vi "Text control 2 v6.7_pump-specific.vi"() -> ()   [LabVIEW 2016]
panel:
  in  "Tab Control":enum32{"Main", "Other parameters"}(tab)
  out "Line running":i32
  out "Total lines":i32
  out "Path":path=path "C:/users/rlp38/09Apr2009LTtesting/test2.txt"
  out "I vs Vg":cluster{"Y data in":dbl[], "X data in":dbl[]}[](graph)
  out "Is max":dbl format="%.2e"
  out "Id max":dbl format="%.2e"
  out "Ig max":dbl format="%.2e"
  out "Imax vs time":cluster{"Y data in":dbl[], "X data in":dbl[]}[](graph)
  out "Imin vs time":cluster{"Y data in":dbl[], "X data in":dbl[]}[](graph)
  out "I vs Vd":cluster{"Y data in":dbl[], "X data in":dbl[]}[](graph)
  in  "Script":string="#-------------------------------------------------------\n# SPM pump cleaning script\n#\n# Version: 0.5\n# Author: Dimitrios Simatos\n# Last updated: 2018-01-05\n#-------------------------------------------------------\n# Description\n#\n# This script is designed to run the cleaning sequence of the SPM OEM pump.\n# This script needs to be run 4 times!\n#-------------------------------------------------------\n# Changes\n#\n# Placed initialization and hard stop commands in the beginning.\n#-------------------------------------------------------\n# Important points\n#\n# Never leave any liquid in the pump to dry after the experiments. If they dry, the residue may block the valve.\n# Always run the cleaning cycle after the experiments.\n# Use clockwise rotation when going up in valve port numbers and vice versa.\n#-------------------------------------------------------\n# Things to do before running the script\n#\n# Set time units to minutes.\n# Set filenames.\n# Replace the tubing, if necessary.\n#-------------------------------------------------------\n# Port connections\n#\n# Port 1: Waste\n# Port 2: Waste\n# Port 3: Various cleaning liquids\n# Port 4: Waste\n# Port 5: Waste\n# Port 6: Waste\n#\n# Between each of the 4 runs, the settings of Port 3 will change, according to the cleaning protocol.\n# The settings for Port 3 are:\n# 1st run: 1% v/v solution of sodium hypochlorite in ultrapure water\n# 2nd run: 0.1% w/v solution of sodium dodecyl sulfate in ultrapure water\n# 3rd run: Ultrapure water\n# 4th run: Waste (in air, not immersed in liquid)\n#-------------------------------------------------------\n# Cleaning protocol for the SPM OEM pump (from the manual)\n#\n# A cleaning procedure should be performed at the end of each day or in between two different experiments.\n# An effective cleaning can be performed in the following manner:\n# • Bleach solution to kill microorganisms\n# 1. Prepare a solution of 1% chlorine bleach and deionized water\n#    NOTE: Prepare a 1% v/v solution of sodium hypochlorite in deionized water\n# 2. Prepare a reservoir and place 1 tubing in the bleach solution and 5 tubings in a waste recipient\n# 3. Pick up the bleach solution through 1 port to entirely fill the syringe\n# 4. Sequentially output the syringe content through the remaining ports and throw it to the waste\n# 5. Repeat operation at least 2 times\n# • Detergent solution to remove debris\n# 1. Prepare a solution of 0.1% detergent and deionized water\n#    NOTE: Prepare a 0.1% w/v solution of sodium dodecyl sulfate in deionized water\n# 2. Move the tubing from the bleach solution reservoir and place it into a reservoir of detergent solution\n# 3. Pick up the detergent solution through 1 port to entirely fill the syringe\n# 4. Sequentially output the detergent solution through the remaining ports into the waste recipient\n# 5. Repeat operation at least 2 times\n# • Rinsing water to prepare the pump for your next experiment\n# 1. Move the tubing from the detergent solution reservoir and place it into a reservoir of deionized water\n# 2. Pick up the rinsing solution through 1 port to entirely fill the syringe\n# 3. Sequentially output the rinse water through the remaining ports into the waste recipient\n# 4. Repeat operation at least 2 times\n# • Replace the tubing, if necessary\n#-------------------------------------------------------\n# Pumping cycles and execution time\n#\n# Execution time for a single cycle: 6 x (1 min + 10 sec) = 7 minutes\n# Total execution time: 4 x 7 = 28 minutes\n# Since the script has to run 4 times, the cleaning lasts for: 4 x 28 = 112 minutes\n# Air must be the last to be pumped through the valve, to remove all liquids.\n# There are 4 pumping cycles. Each one draws a different liquid through port 3 and pumps it sequentially through ports 1,2,4,5,6.\n# During the sequential pumping, each port receives 200 ml of liquid (20% of the total syringe volume = 600 \"plunger units\")\n# The device must be disconnected from the port during the cleaning procedure.\n# All cycles are similar, except cycle 1 has the initialization command uncommented and the first report valve command commented.\n#-------------------------------------------------------\n# Volume of liquid needed\n#\n# Volume of liquid needed per cycle: 1 ml\n# Total volume of liquid needed per script run: 4 x 1 = 4 ml\n# Since the script has to run 4 times, the first 3 with different liquids, I need:\n# 4 ml of 1% v/v solution of sodium hypochlorite in ultrapure water\n# 4 ml of 0.1% w/v solution of sodium dodecyl sulfate in ultrapure water\n# 4 ml of ultrapure water\n#-------------------------------------------------------\n# Parameters\n#\n# Syringe size: 1 ml\n# Step resolution N = 0.01 mm\n# Drawing flow V = 300 pulses/second (6000 ul/min)\n# Pumping flow V = 300 pulses/second (6000 ul/min)\n#-------------------------------------------------------\n# Pump initialization\npump /1T #hard stop pump\npump /1ZR #initialize pump\n#-------------------------------------------------------\n# Cycle 1\n# Fill the syringe\npump /1Q #query pump\npump /1? #report absolute plunger position\n#pump /1?6 #report valve position\nwait-min 1 #wait 1 minute\npump /1N0R #set step resolution: 0.01 mm\npump /1Q #query pump\npump /1? #report absolute plunger position (the plunger should be at 0)\npump /1?6 #report valve position\nwait 1000 #wait 1 second\npump /1V300R #choose speed: 300 steps/s (6000 ul/min)\npump /1Q #query pump\nwait 1000 #wait 1 second\npump /1I3R #go to port 3, clockwise rotation\npump /1Q #query pump\npump /1?6 #report valve position\nwait 1000 #wait 1 second\npump /1A3000R #go to absolute position 3000 (= draw 1 ml)\nwait 30000 #wait 30 seconds\npump /1Q #query pump\npump /1? #report absolute plunger position (the plunger should have finished moving)\n#pump /1?6 #report valve position\n# The sequential pumping begins\n# Port 1\npump /1O1R #switch to port 1, counterclockwise rotation\npump /1Q #query pump\npump /1?6 #report valve position\npump /1A2400R #go to absolute position 2400 (= pump 200 ul)\npump /1Q #query pump\npump /1? #report absolute plunger position (the plunger should be moving to 0)\nwait-min 1 #wait 1 minute\npump /1? #report absolute plunger position (the plunger should have finished moving)\n# Port 2\npump /1I2R #switch to port 2, clockwise rotation\npump /1Q #query pump\npump /1?6 #report valve position\npump /1A1800R #go to absolute position 1800 (= pump 200 ul)\npump /1Q #query pump\npump /1? #report absolute plunger position (the plunger should be moving to 0)\nwait-min 1 #wait 1 minute\npump /1? #report absolute plunger position (the plunger should have finished moving)\n# Port 4\npump /1I4R #switch to port 4, clockwise rotation\npump /1Q #query pump\npump /1?6 #report valve position\npump /1A1200R #go to absolute position 1200 (= pump 200 ul)\npump /1Q #query pump\npump /1? #report absolute plunger position (the plunger should be moving to 0)\nwait-min 1 #wait 1 minute\npump /1? #report absolute plunger position (the plunger should have finished moving)\n# Port 5\npump /1I5R #switch to port 5, clockwise rotation\npump /1Q #query pump\npump /1?6 #report valve position\npump /1A600R #go to absolute position 600 (= pump 200 ul)\npump /1Q #query pump\npump /1? #report absolute plunger position (the plunger should be moving to 0)\nwait-min 1 #wait 1 minute\npump /1? #report absolute plunger position (the plunger should have finished moving)\n# Port 6\npump /1I6R #switch to port 6, clockwise rotation\npump /1Q #query pump\npump /1?6 #report valve position\npump /1A0R #go to absolute position 0 (= pump 200 ul)\npump /1Q #query pump\npump /1? #report absolute plunger position (the plunger should be moving to 0)\nwait-min 1 #wait 1 minute\npump /1? #report absolute plunger position (the plunger should have finished moving)\n#-------------------------------------------------------\n# Cycle 2\n# Fill the syringe\n#pump /1ZR #initialize pump\npump /1Q #query pump\npump /1? #report absolute plunger position\npump /1?6 #report valve position\nwait-min 1 #wait 1 minute\npump /1N0R #set step resolution: 0.01 mm\npump /1Q #query pump\npump /1? #report absolute plunger position (the plunger should be at 0)\npump /1?6 #report valve position\nwait 1000 #wait 1 second\npump /1V300R #choose speed: 300 steps/s (6000 ul/min)\npump /1Q #query pump\nwait 1000 #wait 1 second\npump /1O3R #go to port 3, counterclockwise rotation\npump /1Q #query pump\npump /1?6 #report valve position\nwait 1000 #wait 1 second\npump /1A3000R #go to absolute position 3000 (= draw 1 ml)\nwait 30000 #wait 30 seconds\npump /1Q #query pump\npump /1? #report absolute plunger position (the plunger should have finished moving)\n#pump /1?6 #report valve position\n# The sequential pumping begins\n# Port 1\npump /1O1R #switch to port 1, counterclockwise rotation\npump /1Q #query pump\npump /1?6 #report valve position\npump /1A2400R #go to absolute position 2400 (= pump 200 ul)\npump /1Q #query pump\npump /1? #report absolute plunger position (the plunger should be moving to 0)\nwait-min 1 #wait 1 minute\npump /1? #report absolute plunger position (the plunger should have finished moving)\n# Port 2\npump /1I2R #switch to port 2, clockwise rotation\npump /1Q #query pump\npump /1?6 #report valve position\npump /1A1800R #go to absolute position 1800 (= pump 200 ul)\npump /1Q #query pump\npump /1? #report absolute plunger position (the plunger should be moving to 0)\nwait-min 1 #wait 1 minute\npump /1? #report absolute plunger position (the plunger should have finished moving)\n# Port 4\npump /1I4R #switch to port 4, clockwise rotation\npump /1Q #query pump\npump /1?6 #report valve position\npump /1A1200R #go to absolute position 1200 (= pump 200 ul)\npump /1Q #query pump\npump /1? #report absolute plunger position (the plunger should be moving to 0)\nwait-min 1 #wait 1 minute\npump /1? #report absolute plunger position (the plunger should have finished moving)\n# Port 5\npump /1I5R #switch to port 5, clockwise rotation\npump /1Q #query pump\npump /1?6 #report valve position\npump /1A600R #go to absolute position 600 (= pump 200 ul)\npump /1Q #query pump\npump /1? #report absolute plunger position (the plunger should be moving to 0)\nwait-min 1 #wait 1 minute\npump /1? #report absolute plunger position (the plunger should have finished moving)\n# Port 6\npump /1I6R #switch to port 6, clockwise rotation\npump /1Q #query pump\npump /1?6 #report valve position\npump /1A0R #go to absolute position 0 (= pump 200 ul)\npump /1Q #query pump\npump /1? #report absolute plunger position (the plunger should be moving to 0)\nwait-min 1 #wait 1 minute\npump /1? #report absolute plunger position (the plunger should have finished moving)\n#-------------------------------------------------------\n# Cycle 3\n# Fill the syringe\n#pump /1ZR #initialize pump\npump /1Q #query pump\npump /1? #report absolute plunger position\npump /1?6 #report valve position\nwait-min 1 #wait 1 minute\npump /1N0R #set step resolution: 0.01 mm\npump /1Q #query pump\npump /1? #report absolute plunger position (the plunger should be at 0)\npump /1?6 #report valve position\nwait 1000 #wait 1 second\npump /1V300R #choose speed: 300 steps/s (6000 ul/min)\npump /1Q #query pump\nwait 1000 #wait 1 second\npump /1O3R #go to port 3, counterclockwise rotation\npump /1Q #query pump\npump /1?6 #report valve position\nwait 1000 #wait 1 second\npump /1A3000R #go to absolute position 3000 (= draw 1 ml)\nwait 30000 #wait 30 seconds\npump /1Q #query pump\npump /1? #report absolute plunger position (the plunger should have finished moving)\n#pump /1?6 #report valve position\n# The sequential pumping begins\n# Port 1\npump /1O1R #switch to port 1, counterclockwise rotation\npump /1Q #query pump\npump /1?6 #report valve position\npump /1A2400R #go to absolute position 2400 (= pump 200 ul)\npump /1Q #query pump\npump /1? #report absolute plunger position (the plunger should be moving to 0)\nwait-min 1 #wait 1 minute\npump /1? #report absolute plunger position (the plunger should have finished moving)\n# Port 2\npump /1I2R #switch to port 2, clockwise rotation\npump /1Q #query pump\npump /1?6 #report valve position\npump /1A1800R #go to absolute position 1800 (= pump 200 ul)\npump /1Q #query pump\npump /1? #report absolute plunger position (the plunger should be moving to 0)\nwait-min 1 #wait 1 minute\npump /1? #report absolute plunger position (the plunger should have finished moving)\n# Port 4\npump /1I4R #switch to port 4, clockwise rotation\npump /1Q #query pump\npump /1?6 #report valve position\npump /1A1200R #go to absolute position 1200 (= pump 200 ul)\npump /1Q #query pump\npump /1? #report absolute plunger position (the plunger should be moving to 0)\nwait-min 1 #wait 1 minute\npump /1? #report absolute plunger position (the plunger should have finished moving)\n# Port 5\npump /1I5R #switch to port 5, clockwise rotation\npump /1Q #query pump\npump /1?6 #report valve position\npump /1A600R #go to absolute position 600 (= pump 200 ul)\npump /1Q #query pump\npump /1? #report absolute plunger position (the plunger should be moving to 0)\nwait-min 1 #wait 1 minute\npump /1? #report absolute plunger position (the plunger should have finished moving)\n# Port 6\npump /1I6R #switch to port 6, clockwise rotation\npump /1Q #query pump\npump /1?6 #report valve position\npump /1A0R #go to absolute position 0 (= pump 200 ul)\npump /1Q #query pump\npump /1? #report absolute plunger position (the plunger should be moving to 0)\nwait-min 1 #wait 1 minute\npump /1? #report absolute plunger position (the plunger should have finished moving)\n#-------------------------------------------------------\n# Cycle 4\n# Fill the syringe\n#pump /1ZR #initialize pump\npump /1Q #query pump\npump /1? #report absolute plunger position\npump /1?6 #report valve position\nwait-min 1 #wait 1 minute\npump /1N0R #set step resolution: 0.01 mm\npump /1Q #query pump\npump /1? #report absolute plunger position (the plunger should be at 0)\npump /1?6 #report valve position\nwait 1000 #wait 1 second\npump /1V300R #choose speed: 300 steps/s (6000 ul/min)\npump /1Q #query pump\nwait 1000 #wait 1 second\npump /1O3R #go to port 3, counterclockwise rotation\npump /1Q #query pump\npump /1?6 #report valve position\nwait 1000 #wait 1 second\npump /1A3000R #go to absolute position 3000 (= draw 1 ml)\nwait 30000 #wait 30 seconds\npump /1Q #query pump\npump /1? #report absolute plunger position (the plunger should have finished moving)\n#pump /1?6 #report valve position\n# The sequential pumping begins\n# Port 1\npump /1O1R #switch to port 1, counterclockwise rotation\npump /1Q #query pump\npump /1?6 #report valve position\npump /1A2400R #go to absolute position 2400 (= pump 200 ul)\npump /1Q #query pump\npump /1? #report absolute plunger position (the plunger should be moving to 0)\nwait-min 1 #wait 1 minute\npump /1? #report absolute plunger position (the plunger should have finished moving)\n# Port 2\npump /1I2R #switch to port 2, clockwise rotation\npump /1Q #query pump\npump /1?6 #report valve position\npump /1A1800R #go to absolute position 1800 (= pump 200 ul)\npump /1Q #query pump\npump /1? #report absolute plunger position (the plunger should be moving to 0)\nwait-min 1 #wait 1 minute\npump /1? #report absolute plunger position (the plunger should have finished moving)\n# Port 4\npump /1I4R #switch to port 4, clockwise rotation\npump /1Q #query pump\npump /1?6 #report valve position\npump /1A1200R #go to absolute position 1200 (= pump 200 ul)\npump /1Q #query pump\npump /1? #report absolute plunger position (the plunger should be moving to 0)\nwait-min 1 #wait 1 minute\npump /1? #report absolute plunger position (the plunger should have finished moving)\n# Port 5\npump /1I5R #switch to port 5, clockwise rotation\npump /1Q #query pump\npump /1?6 #report valve position\npump /1A600R #go to absolute position 600 (= pump 200 ul)\npump /1Q #query pump\npump /1? #report absolute plunger position (the plunger should be moving to 0)\nwait-min 1 #wait 1 minute\npump /1? #report absolute plunger position (the plunger should have finished moving)\n# Port 6\npump /1I6R #switch to port 6, clockwise rotation\npump /1Q #query pump\npump /1?6 #report valve position\npump /1A0R #go to absolute position 0 (= pump 200 ul)\npump /1Q #query pump\npump /1? #report absolute plunger position (the plunger should be moving to 0)\nwait-min 1 #wait 1 minute\npump /1? #report absolute plunger position (the plunger should have finished moving)\n#-------------------------------------------------------"
  out "Command running:":string
  out "Serial port data":string
  out "Elapsed Time":dbl caption="Elapsed Time (s)"
  in  "Time Units":u16(ring)=1 items=["Seconds", "Minutes", "Hours"]
  in  "Time Offset":dbl caption="Set Start Time (s)"
  in  "Reset":bool
  in  "Auto Reset":bool
  in  "integration time":u32(slide) max=2 step=1 scale=0.0..2.0
  in  "Interrupt scan":bool
  out "Absolute plunger position vs time":cluster{"Y data in":dbl[], "X data in":dbl[]}[](graph)
  out "Valve position vs time":cluster{"Y data in":dbl[], "X data in":dbl[]}[](graph)
  out "Is on":dbl format="%.2e"
  out "Id on":dbl format="%.2e"
  out "Ig on":dbl format="%.2e"
  out "Ion vs time":cluster{"Y data in":dbl[], "X data in":dbl[]}[](graph)
  out "Ioff vs time":cluster{"Y data in":dbl[], "X data in":dbl[]}[](graph)
  out "Ig min":dbl format="%.2e"
  out "Id min":dbl format="%.2e"
  out "Is min":dbl format="%.2e"
  out "Is off":dbl format="%.2e"
  out "Id off":dbl format="%.2e"
  out "Ig off":dbl format="%.2e"
  in  "Integration time (long)":dbl=0.32 min=0.04 max=2.0 step=0.02 format="%.2f"
  in  "Integration time (short)":dbl=0.0019 min=8e-05 max=0.0019 step=8e-05 format="%^.0e"
  in  "Gate: Compliance":dbl=0.001 format="%.8f"
  in  "Drain: Compliance":dbl=0.001 format="%.8f"
  in  "Hard stop pump":bool
  in  "Halt pump":bool
  in  "Interrupt program":bool
  in  "Suffix (script)":string="step_1_up-H2O_initial_script.txt"
  in  "Filename (variable part)":string="step_1_up-H2O_initial_"
  in  "Plot output curve extrema vs time":bool
  in  "Plot transfer curve extrema vs time":bool=TRUE
  in  "Plot sample extrema vs time":bool
  out "I vs time (Bias Stress)":cluster{"Y data in":dbl[], "X data in":dbl[]}[](graph)
  in  "Gate Range\nmode":u16(ring) items=["Auto", "Limited", "Fixed"]
  in  "Gate Range":u8(slide)=6 max=11 scale=0.0..11.0
  in  "Source/Drain\nRange mode":u16(ring) items=["Auto", "Limited", "Fixed"]
  in  "Source/Drain Range":u8(slide)=6 max=11 scale=0.0..11.0
  in  "Panel Controls":T1={"Emergency Stop"=refnum, "TransGraph Max"=1e-05, "Text/Graph (text=false)"=TRUE} {"TransGraph Max" format="%.2e"}
  in  "Panel Controls 2":T2={"Emergency Stop"=refnum, "TransGraph Max"=1e-05, "Text/Graph (text=false)"=TRUE, "TransGraph Min"=1e-11} {"TransGraph Min" format="%.2e"; "TransGraph Max" format="%.2e"}
  in  "SMU4":cluster{"on/off":bool, "Voltage":dbl} {"Voltage" min=-100.0 max=100.0 format="%.2f"}
  in  "Full Reset":bool
  in  "Standby":T3
  out "error out":errorcluster
  in  "Delay before read (ms)":u32=1000
  in  "byte count":u32=64
  in  "Serial End Mode for Reads":u16(ring)=2 items=["None", "LastBit", "TermChar"]
  in  "Timeout (ms)":u32=10000
  in  "Enable Termination\nChar (T)":bool=TRUE
  in  "Termination char\n(0xA = '\\n' = LF)\n(0xD = '\\r' = CR)":u8=13 format="%.0x"
  in  "flow control":u16(ring) items=["None"=0, "XON/XOFF"=1, "RTS/CTS"=2, "DTR/DSR"=4]
  in  "stop bits":u16(ring)=10 items=["1.0"=10, "1.5"=15, "2.0"=20]
  in  "parity":u16(ring) items=["None", "Odd", "Even", "Mark", "Space"]
  in  "data bits":u16=8 min=5 max=8 step=1
  in  "VISA resource name":refnum<visa-resource-name>="COM6"
  in  "baud rate":u32=9600
  out "Timings Indicator":T4
  in  "Timings (overwritten by the Front Panel)":T5={"integration time"=0, "Short/Long integration time"=0.00064, "hold time (sec)"=0.0, "delay time (sec)"=0.0, "Step Time (0 disables)"=0.0, "sweep method"=0, "Pulse period"=0.005, "Base voltage"=0.0, "Pulse width"=0.0005} {"Pulse width" min=0.0005 max=0.1 step=0.0001 format="%.4f"; "Base voltage" format="%^.4e"; "Pulse period" min=0.005 max=1.0 step=0.0001 format="%.4f"; "sweep method" items=["Continuous", "Pulsed"]; "Step Time (0 disables)" format="%.2f"; "delay time (sec)" format="%.4f"; "hold time (sec)" format="%.4f"; "Short/Long integration time" format="%^.0e"; "integration time" scale=0.0..2.0}
  out "SMU4 Indicator":cluster{"on/off":bool, "Voltage":dbl} {"Voltage" min=-100.0 max=100.0 format="%.2f"}
  in  "Gate":T6={"Gate Start"=0.0, "Gate Stop"=2.0, "Gate Step (linear only)"=1.0, "Gate Compliance"=0.0001, "Gate PComp"=0.0, "Range mode"=0, "Range"=6} {"Range" max=11 scale=0.0..11.0; "Range mode" items=["Auto", "Limited", "Fixed"]; "Gate PComp" format="%^.2e"; "Gate Compliance" format="%^.2e"; "Gate Step (linear only)" format="%^.4e"; "Gate Stop" format="%^.4e"; "Gate Start" format="%^.4e"}
  in  "Drain 2":T7={"Drain Start"=0.0, "Drain Stop"=2.0, "Drain Compliance"=0.0001, "Drain Step"=1.0, "Drain PComp"=0.0, "Range mode"=0, "Range"=6} {"Range" max=11 scale=0.0..11.0; "Range mode" items=["Auto", "Limited", "Fixed"]; "Drain PComp" format="%^.2e"; "Drain Step" format="%^.4e"; "Drain Compliance" format="%^.2e"; "Drain Stop" format="%^.4e"; "Drain Start" format="%^.4e"}
  # "Syntax:\nitime [s|m|l] time(sec): [s|m|l] determines the integration time setting (small|medium|long) and time sets the value.\nNOTE: The value of the integration time has to be within the range allowed by its category (s|m|l), otherwise, the closest value will be used. (e.g. if the category is set to short but the time value is very long, the actual value used will be the maximum short integration time.\nIntegration times:\n    Short: Default: 640 us. Range: 8E-5 - 1.92E-3 seconds.\n    Medium: Fixed at 1 NPL cycle (0.02 seconds).\n    Long: Default: 16 NPL cycles (0.32 seconds). Range: 2-100 NPL cycles (0.04 seconds - 2 seconds).\ngaterangemode [a|l|f]\ndrainrangemode [a|l|f]\npulsed [on|off] PulsePeriod(sec) PulseBaseVoltage PulseONWidth(sec)\nstandby [on l off]\nwait NumMilliseconds\nwait-min NumMinutes\n# texthere = comment\nSMU4 [ON|OFF] Voltage\ntransfer [s|d] VgStart VgStop VgStep VdStart VdStop VdStep\noutput [s|d] VgStart VgStop VgStep VdStart VdStop VdStep\nsample Vg Vd NumSamples Time(s) SampleInterval(s)\nsamplei Idg NumSamples Time(s) SampleInterval(s) VDGcompliance\n100 samples is approximately 13 seconds with medium integration\n# If in doubt use SampleInterval(s) = 0.004\n    NOTE: When doing bias stress measurements, set the Time Units to \"Seconds\", as the \"sample\" command has been configured to give the output to seconds.\nstressV VG VD IGcompliance IDcompliance Duration(sec)\nstressI IDG VDGcompliance Duration(sec)\nvsu2pulse Bias Duration(s)\npulsedstressV [s|d] VEstop VgON VgOFF Period(s) PulseONwidth(s) Vd\nsample-fpp Vg Vd NumSamples Time\nresample-fpp Vg Vd\ntransfer-fpp [s|d] VgStart VgStop VgStep VdStart VdStop VdStep\noutput-fpp [s|d] VgStart VgStop VgStep VdStart VdStop VdStep\nserial SerialPortCommand\npump SerialPortCommand for the SPM pump\n\nSPM Pump Syntax (<x>: pump number, use 1 if only one pump):\nif the command syntax contains [R], then append the letter R to the command\n/<x>Q: query (a query command should follow each command)\n/<x>Z[R] or /<x>Y[R]: initialize pump\n/<x>N<n>[R] (<n>=0,1): <0> (<1>) microstep 0.01 mm (0.00125 mm) resolution\n/<x>I<n> (<n>=0-6): turn to port number n (clockwise)\n/<x>O<n> (<n>=0-6): turn to port number n (counterclockwise)\n/<x>X: Re-execute last command string\n/<x>G<n>[R] (<n>=0-60000): repeat command sequence (default: 0, 0=loop forever)\n/<x>g: Mark the start of a repeat sequence (max = 10)\n/<x>M<n>[R] (<n>=0-86400000): delay command execution by n milliseconds\n/<x>H: Halt; Pause the sequence after finishing the current move\n/<x>T: Hardstop; Interrupt the current move and suppress it from the sequence\n/<x>A<n>[R] (<n>=0-3000 with N=0, 0-24000 with N=1): absolute position\n/<x>P<n>[R] (<n>=0-3000 with N=0, 0-24000 with N=1): relative pickup\n/<x>D<n>[R] (<n>=0-3000 with N=0, 0-24000 with N=1): relative dispense\n/<x>V<n>[R] (<n>=1-1600 default: 150): set peak speed (pulses/sec)\nNOTE: The lowest speed limit is 1 pulse/sec, not 5, as the manual states.\n/<x>S<n>[R] (<n>=10-40 default: 22): set speed (NOT in pulses/sec, look in manual)\nNOTE: When controlled with absolute position, one does not need to pay special attention to the syringe that is mounted on the pump.\nWithdraw from lower stage (ports 3, 5), dispense from higher stage (ports 2, 4, 6).\nConnect Port 1 to waste."
  # "Time"
  # "1\n2\n3\n4\n5\n6\n7\n8\n9\n10\n11\n12\n13\n14\n15\n16\n17\n18\n19\n20"
  # "Serial port settings"
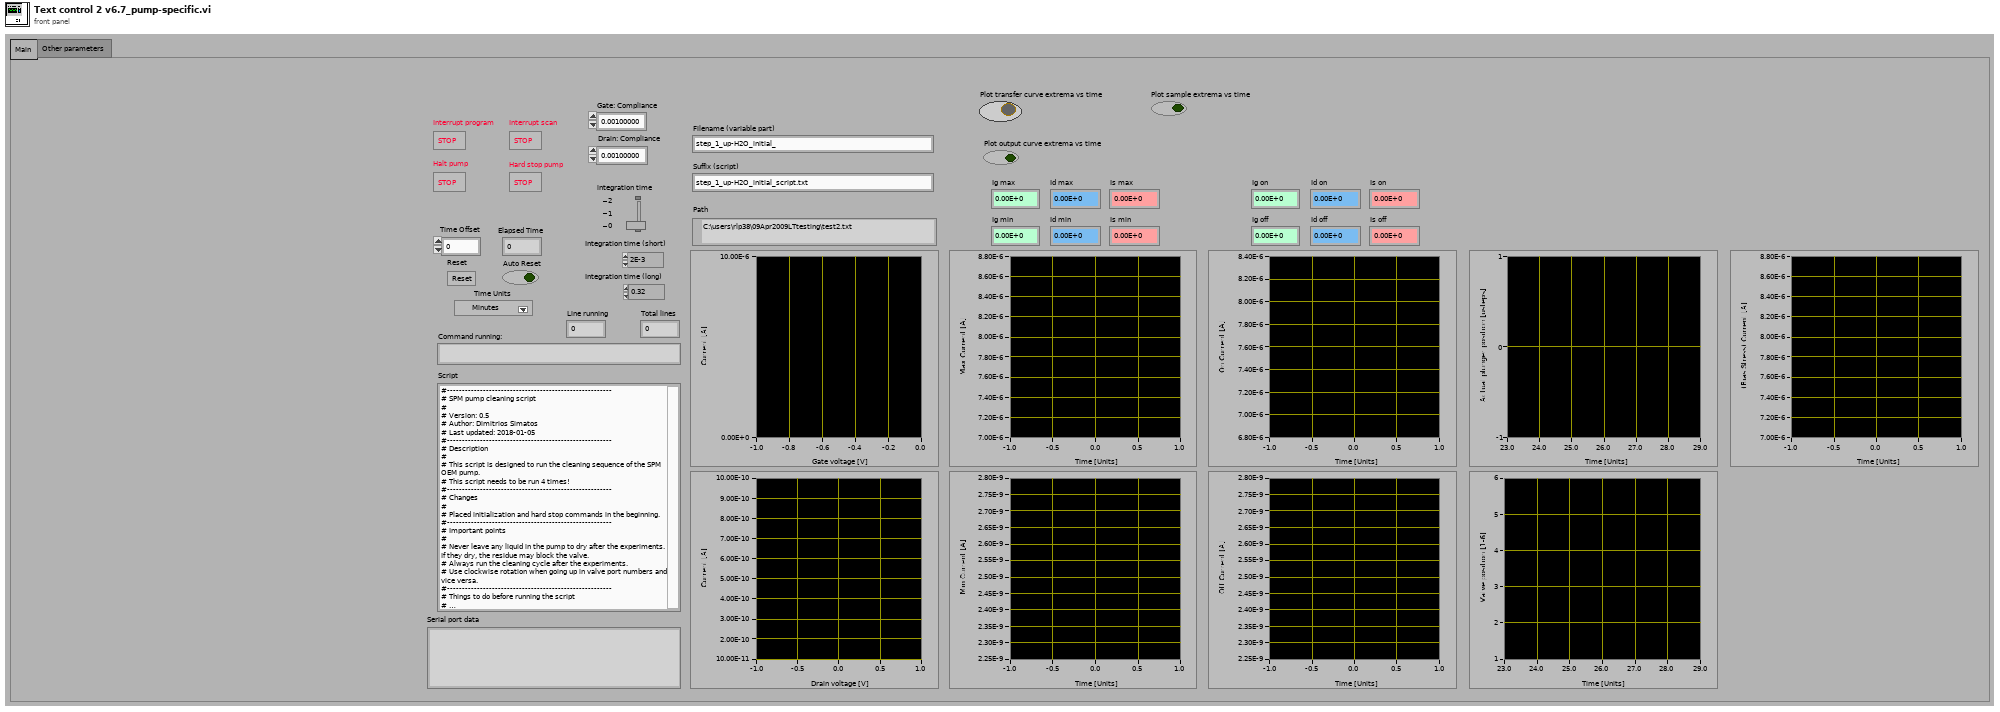
[diagram p1: front panel]
types:
  T1 = cluster{"Emergency Stop":refnum<vi>, "TransGraph Max":dbl, "Text/Graph (text=false)":bool}
  T2 = cluster{"Emergency Stop":refnum<vi>, "TransGraph Max":dbl, "Text/Graph (text=false)":bool, "TransGraph Min":dbl}
  T3 = cluster{"Gate Standby":bool, "Drain Standby":bool}
  T4 = cluster{"integration time (0:s, 1:m, 2:l)":u32, "Short/Long integration time":dbl, "hold time (sec)":dbl, "delay time (sec)":dbl, "Step Time (0 disables)":dbl, "sweep method":u16, "Pulse period":dbl, "Base voltage":dbl, "Pulse width":dbl}
  T5 = cluster{"integration time":u32, "Short/Long integration time":dbl, "hold time (sec)":dbl, "delay time (sec)":dbl, "Step Time (0 disables)":dbl, "sweep method":u16, "Pulse period":dbl, "Base voltage":dbl, "Pulse width":dbl}
  T6 = cluster{"Gate Start":dbl, "Gate Stop":dbl, "Gate Step (linear only)":dbl, "Gate Compliance":dbl, "Gate PComp":dbl, "Range mode":u16, "Range":u8}
  T7 = cluster{"Drain Start":dbl, "Drain Stop":dbl, "Drain Compliance":dbl, "Drain Step":dbl, "Drain PComp":dbl, "Range mode":u16, "Range":u8}
  T8 = enum16{"open", "replace", "create", "open or create", "replace or create", "replace or create with confirmation"}
  T9 = cluster{"V2 Start":dbl, "V2 Step":dbl, "Number of points":i32}
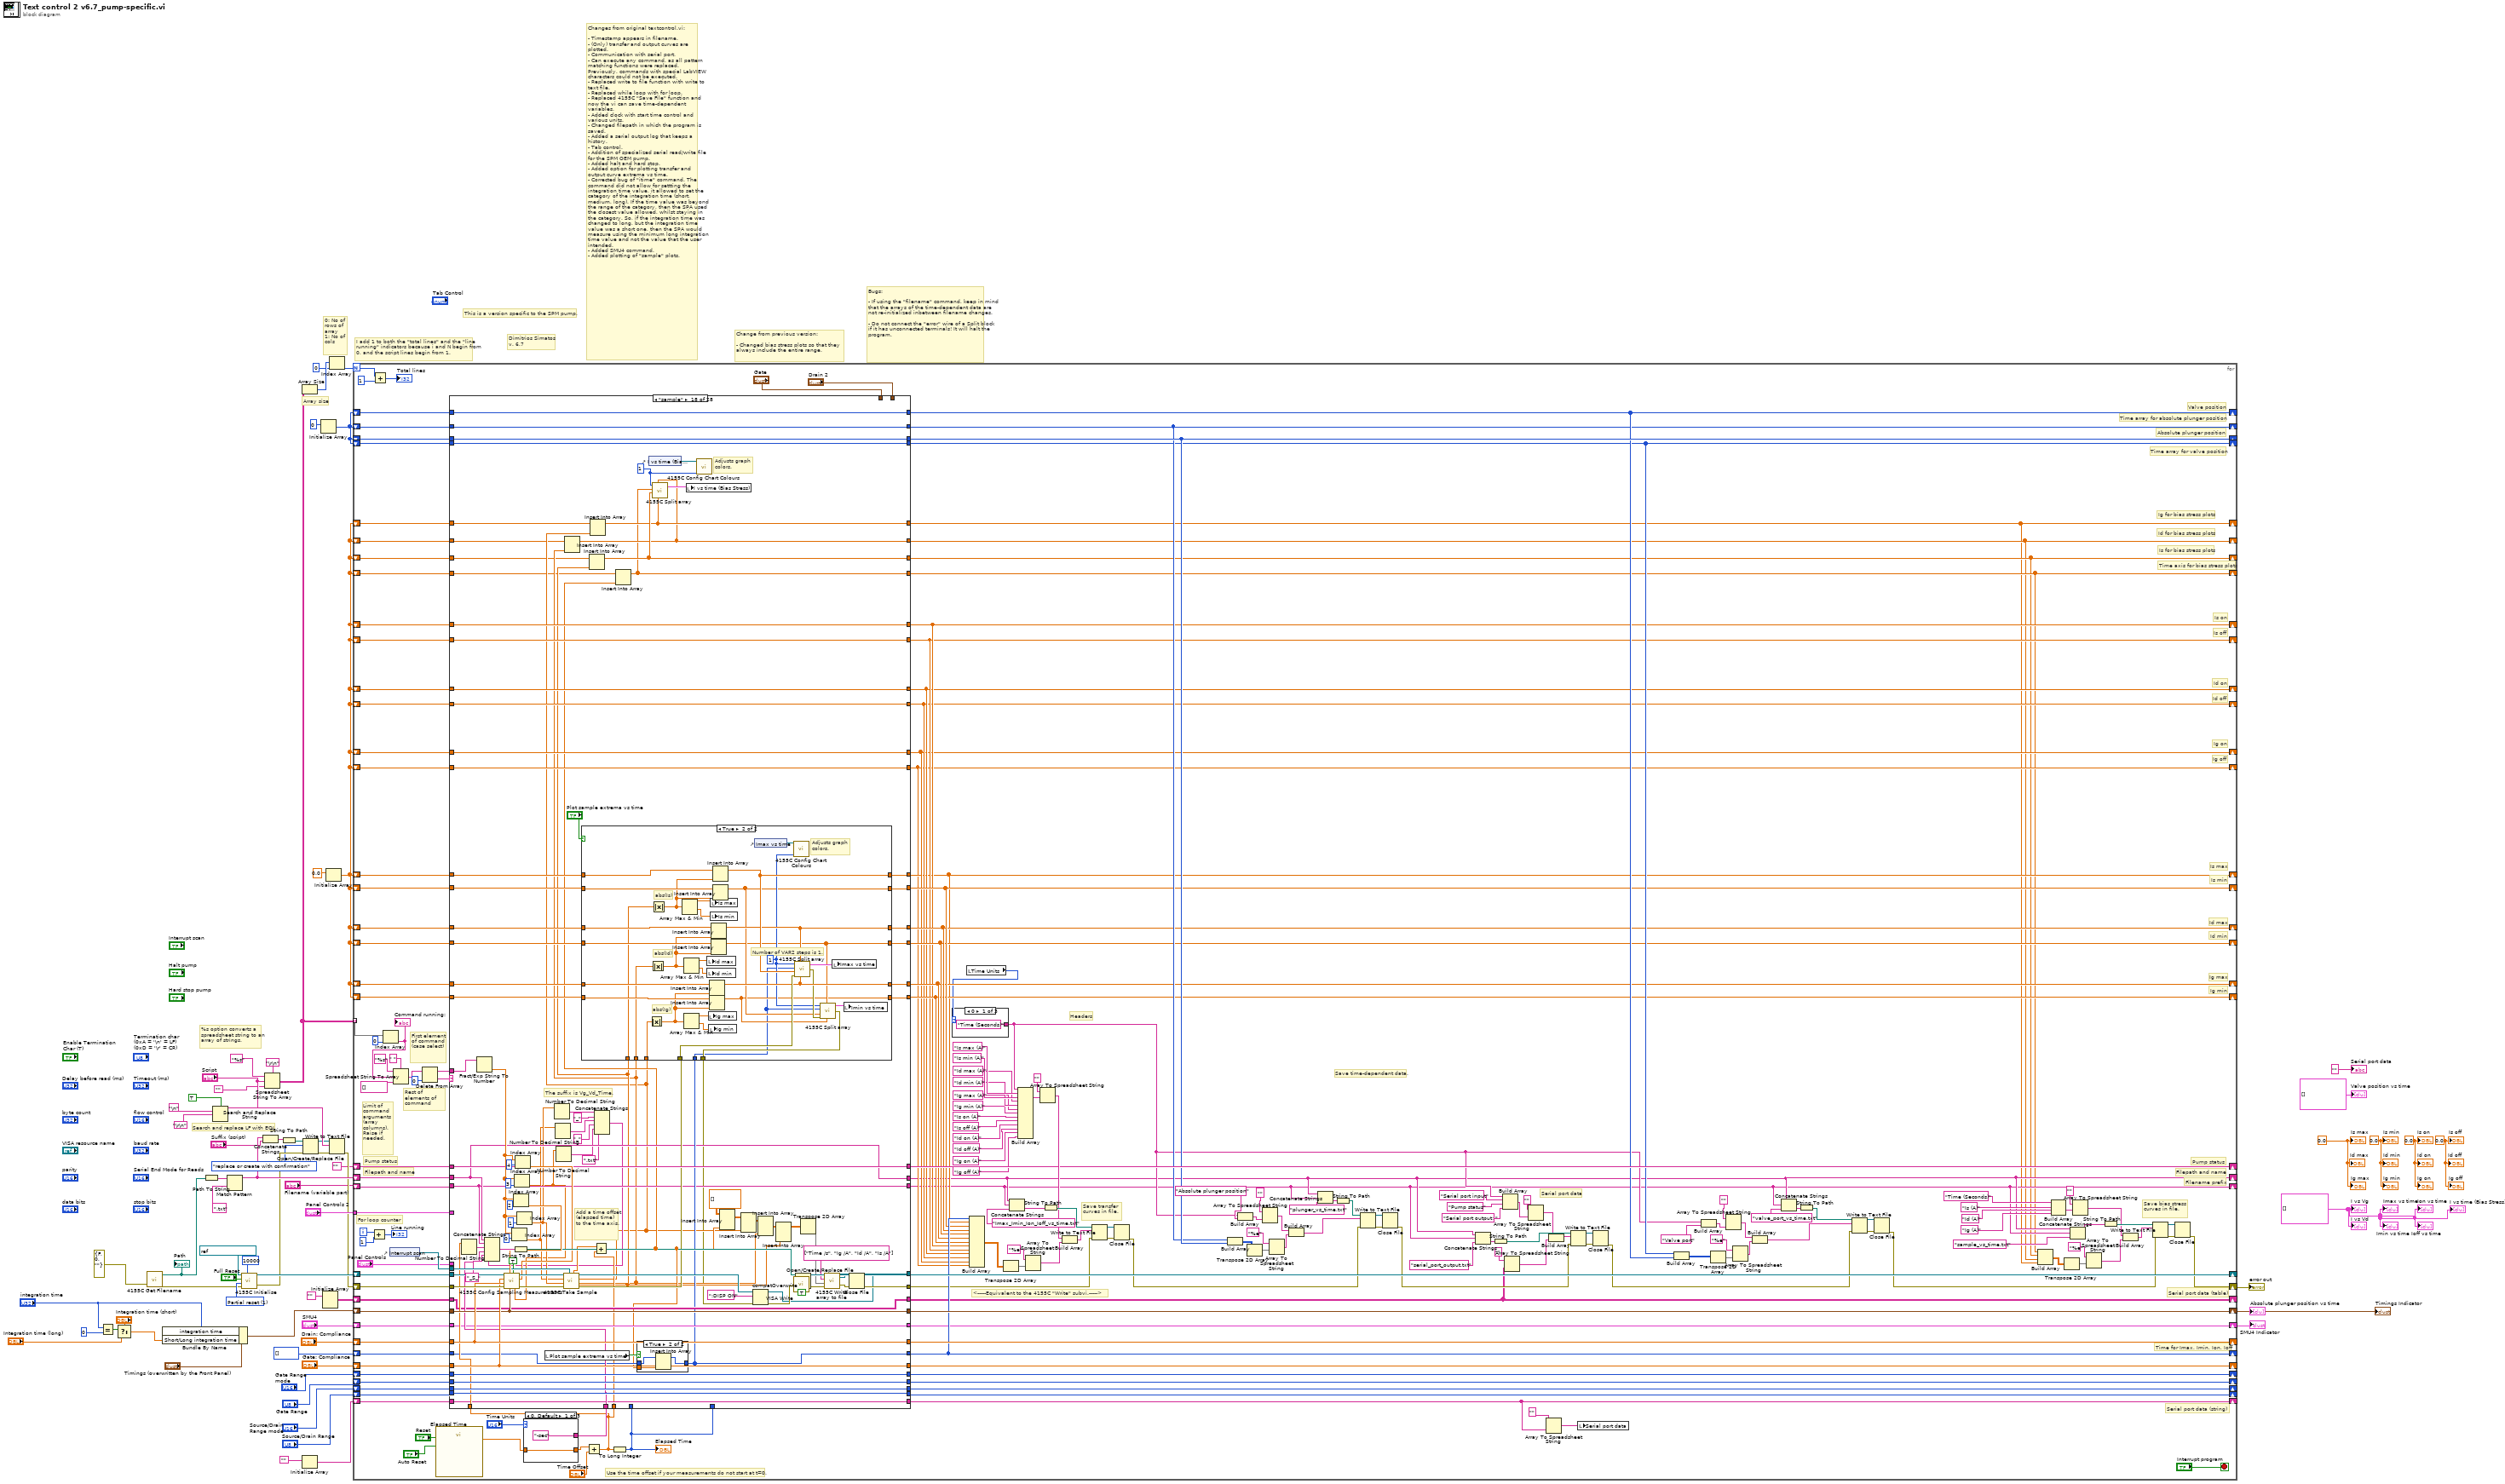
[diagram p0: block diagram]
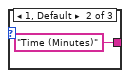
[diagram p2: hidden frame]
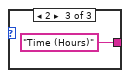
[diagram p3: hidden frame]
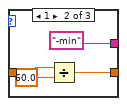
[diagram p4: hidden frame]
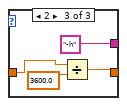
[diagram p5: hidden frame]
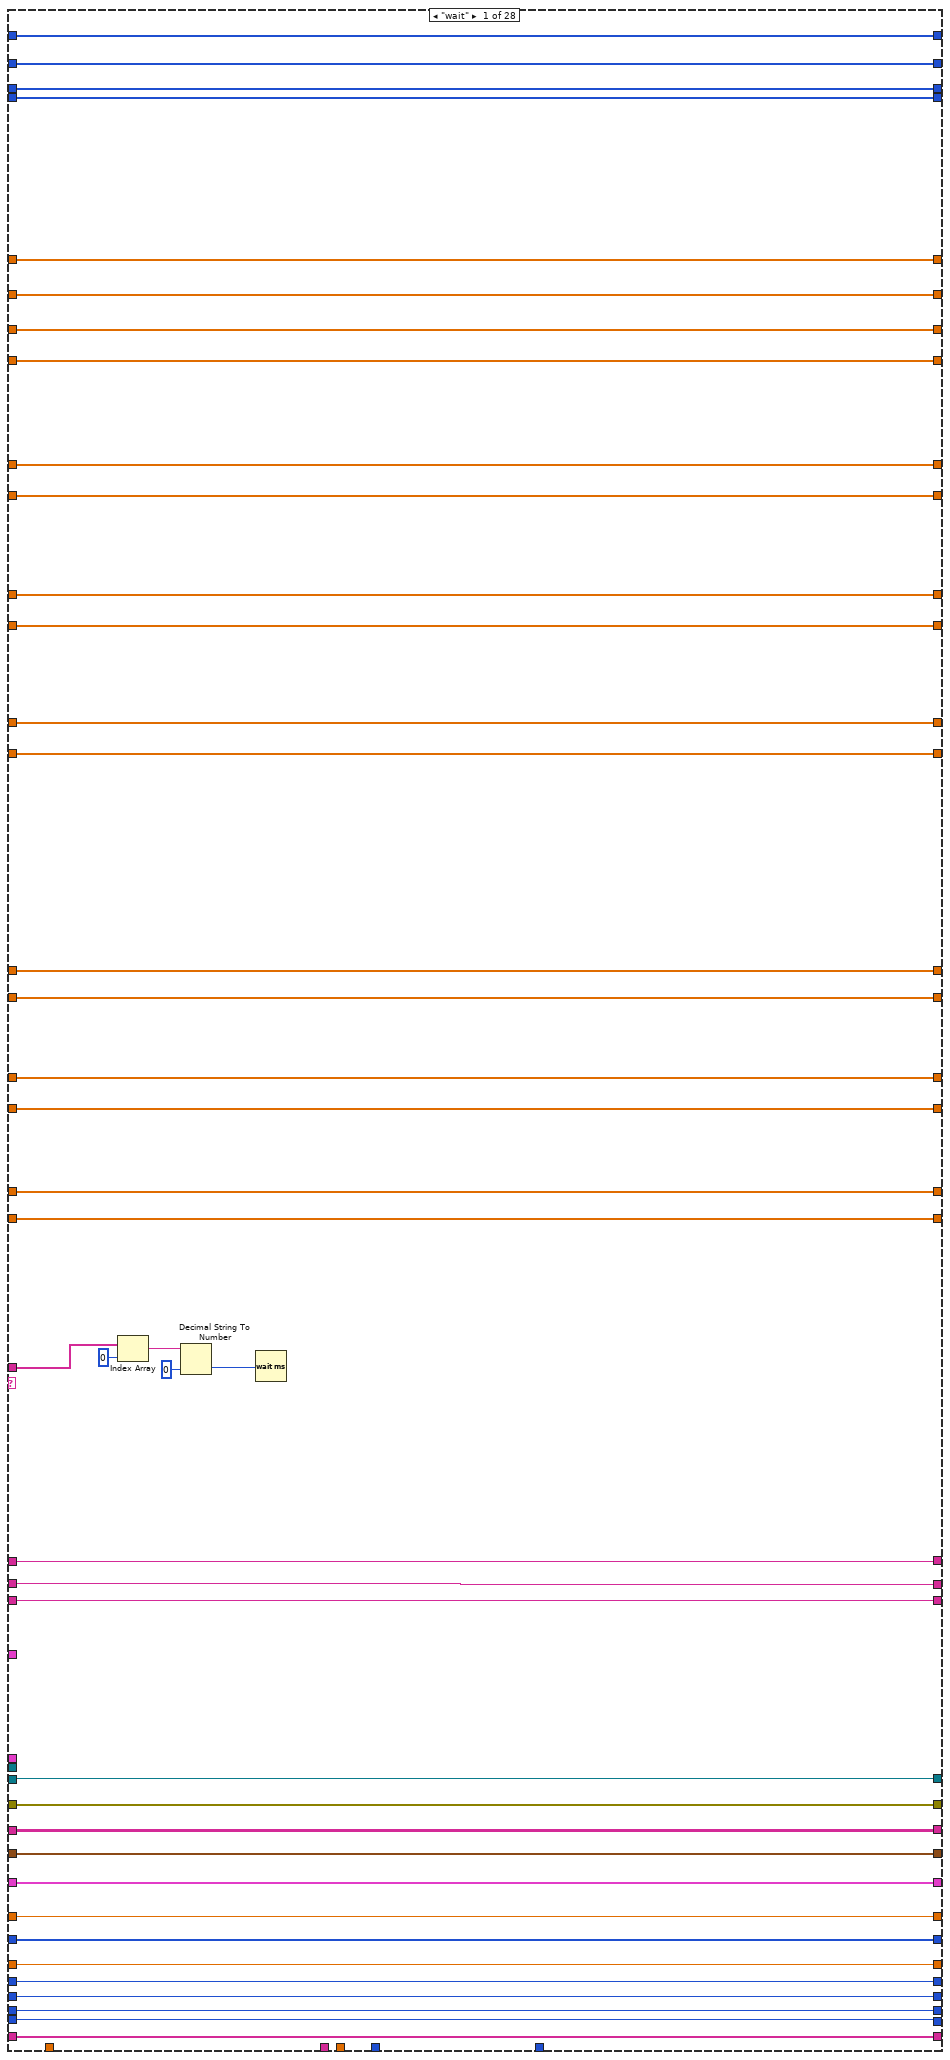
[diagram p6: hidden frame]
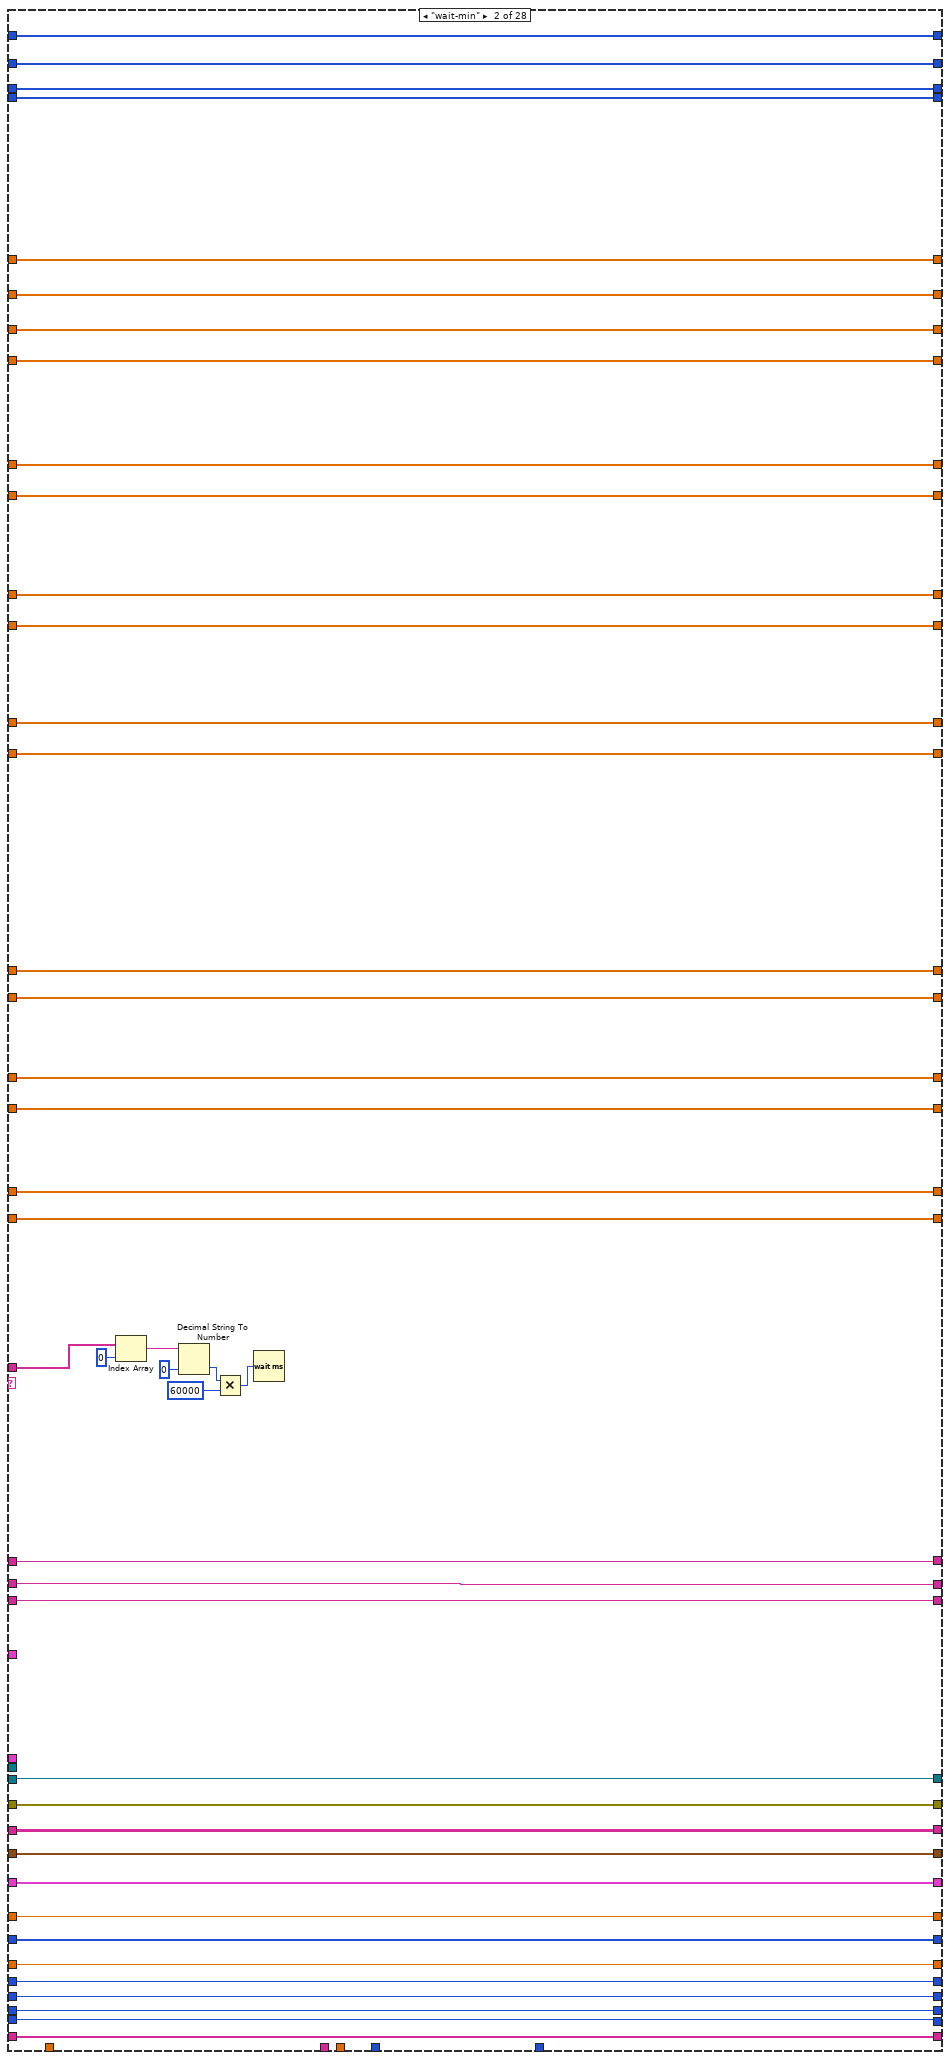
[diagram p7: hidden frame]
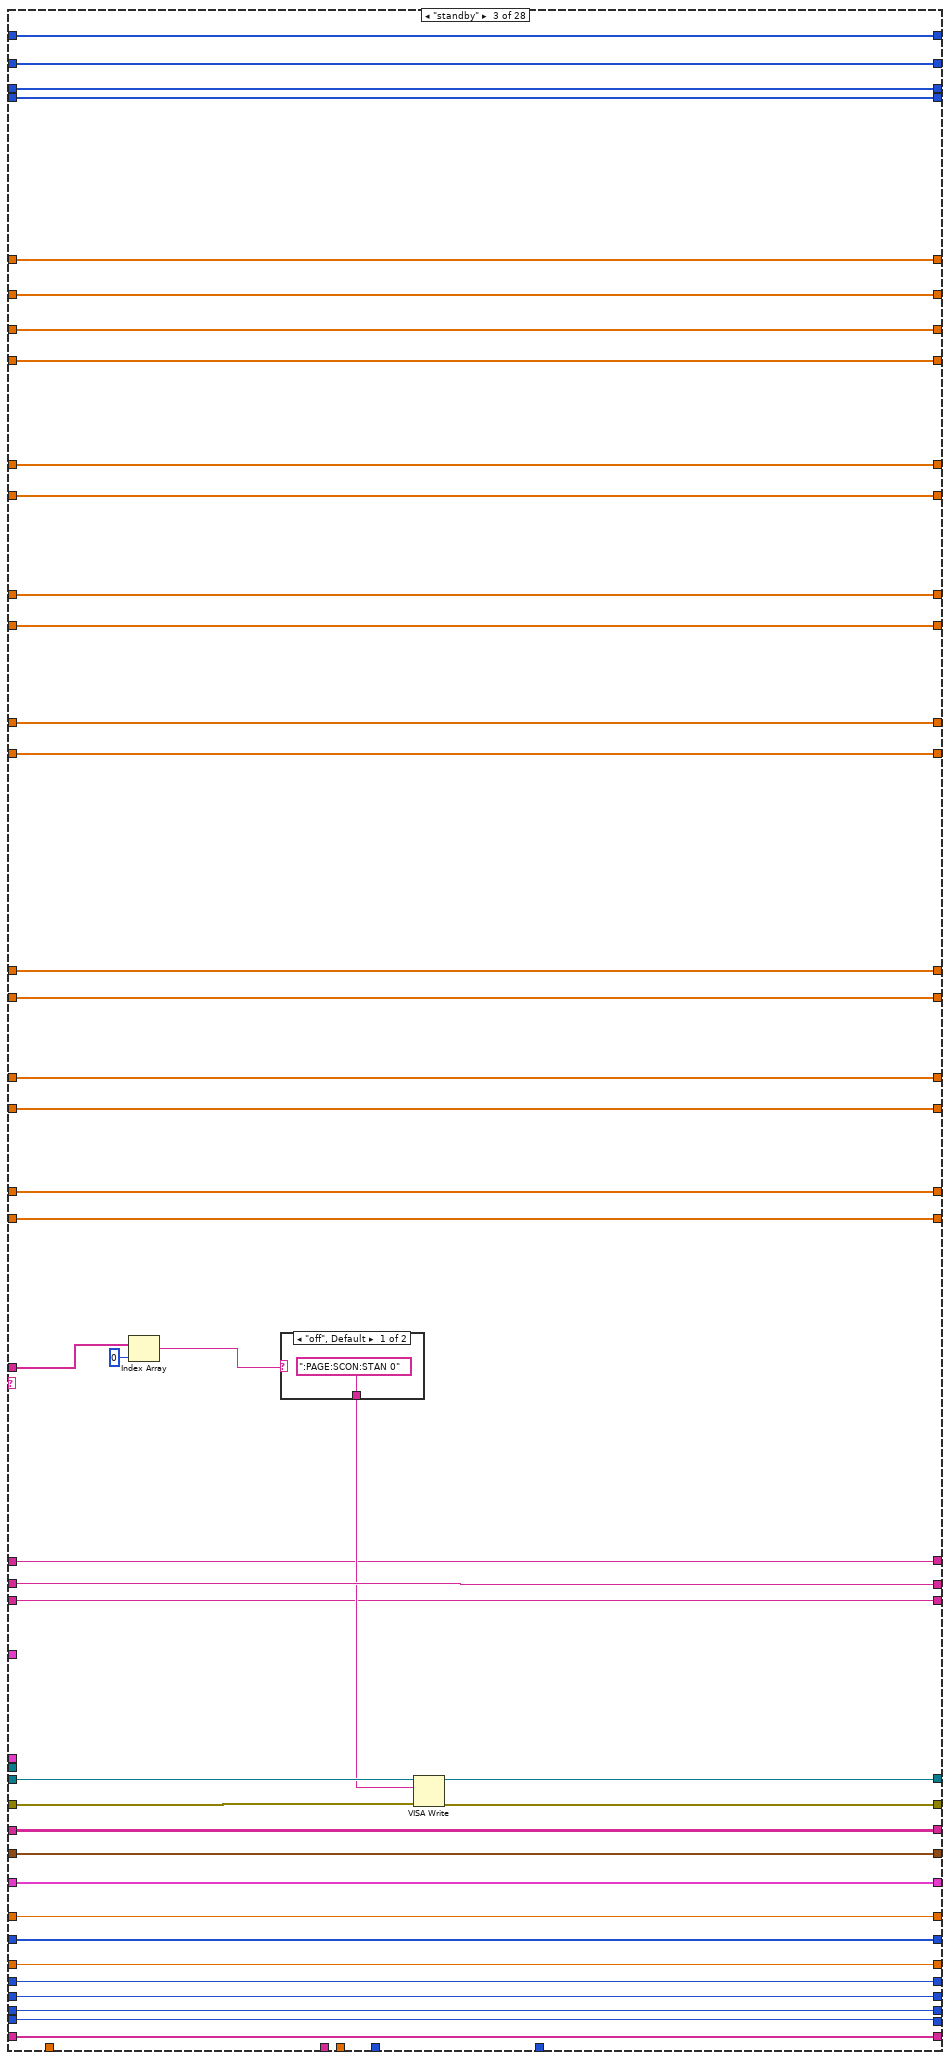
[diagram p8: hidden frame]
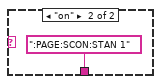
[diagram p9: hidden frame]
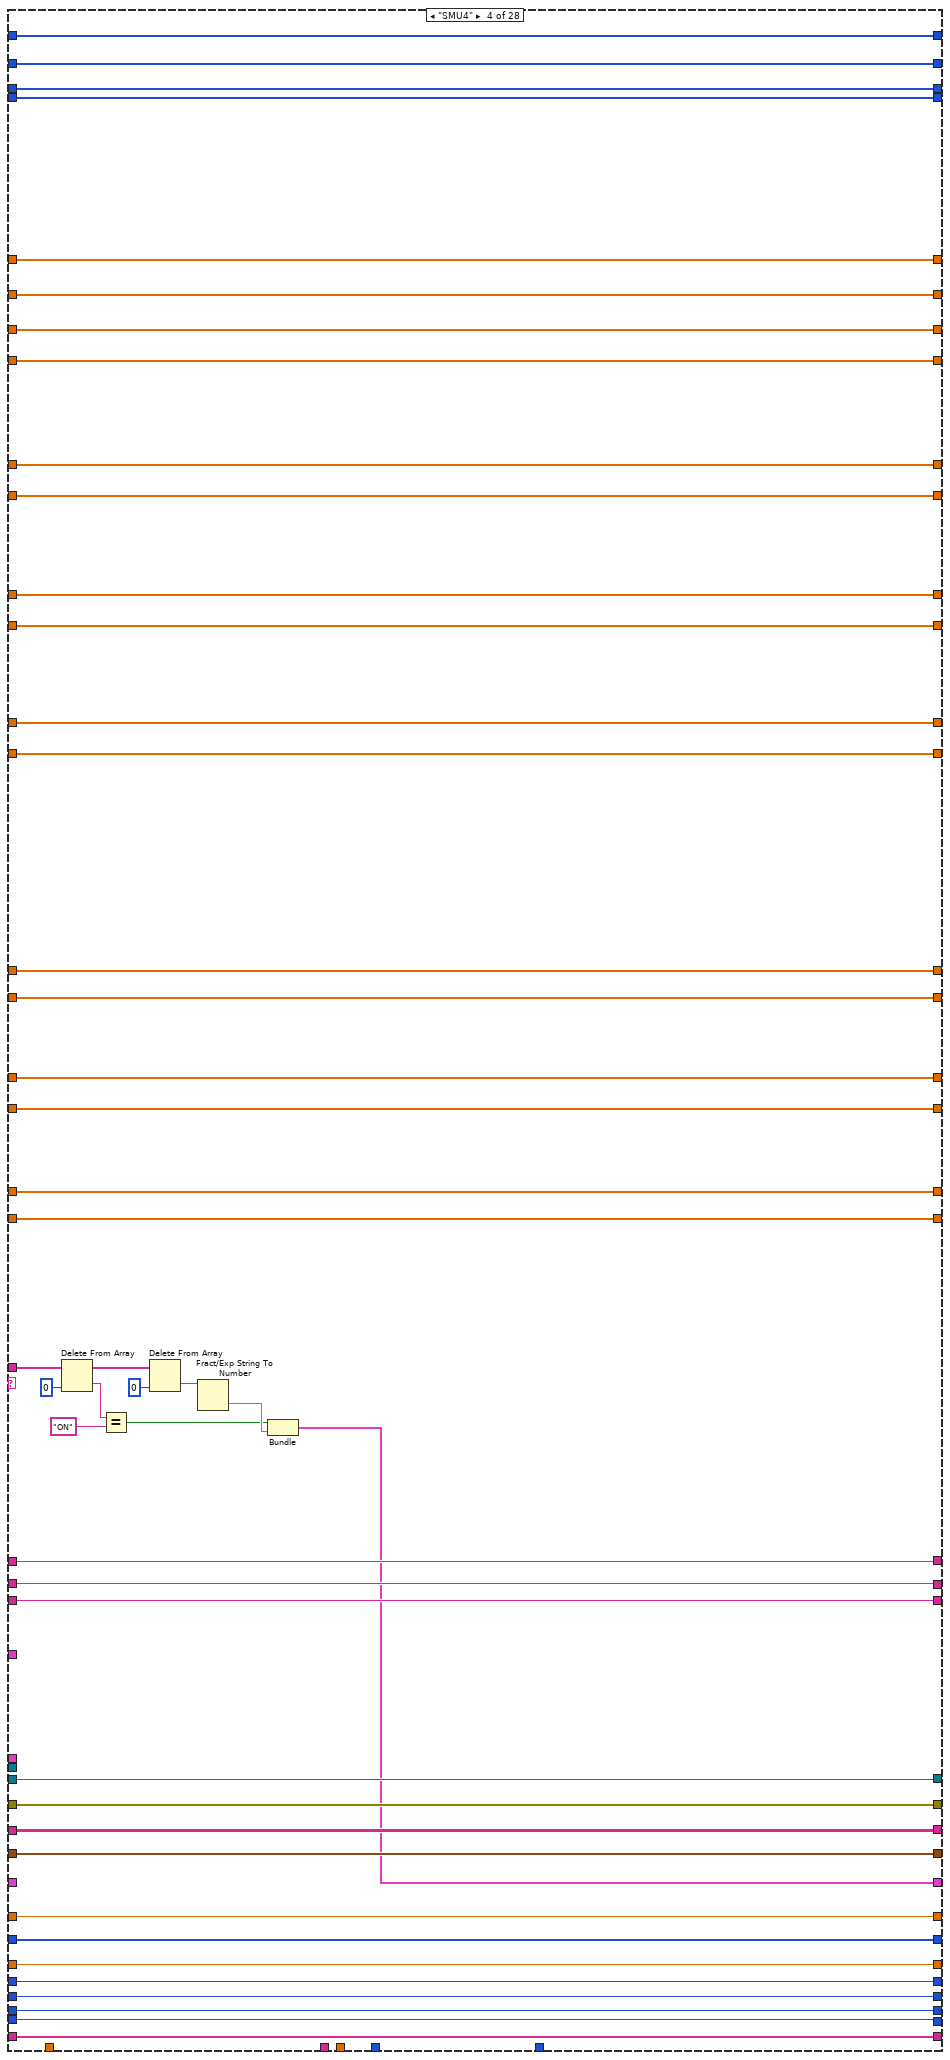
[diagram p10: hidden frame]
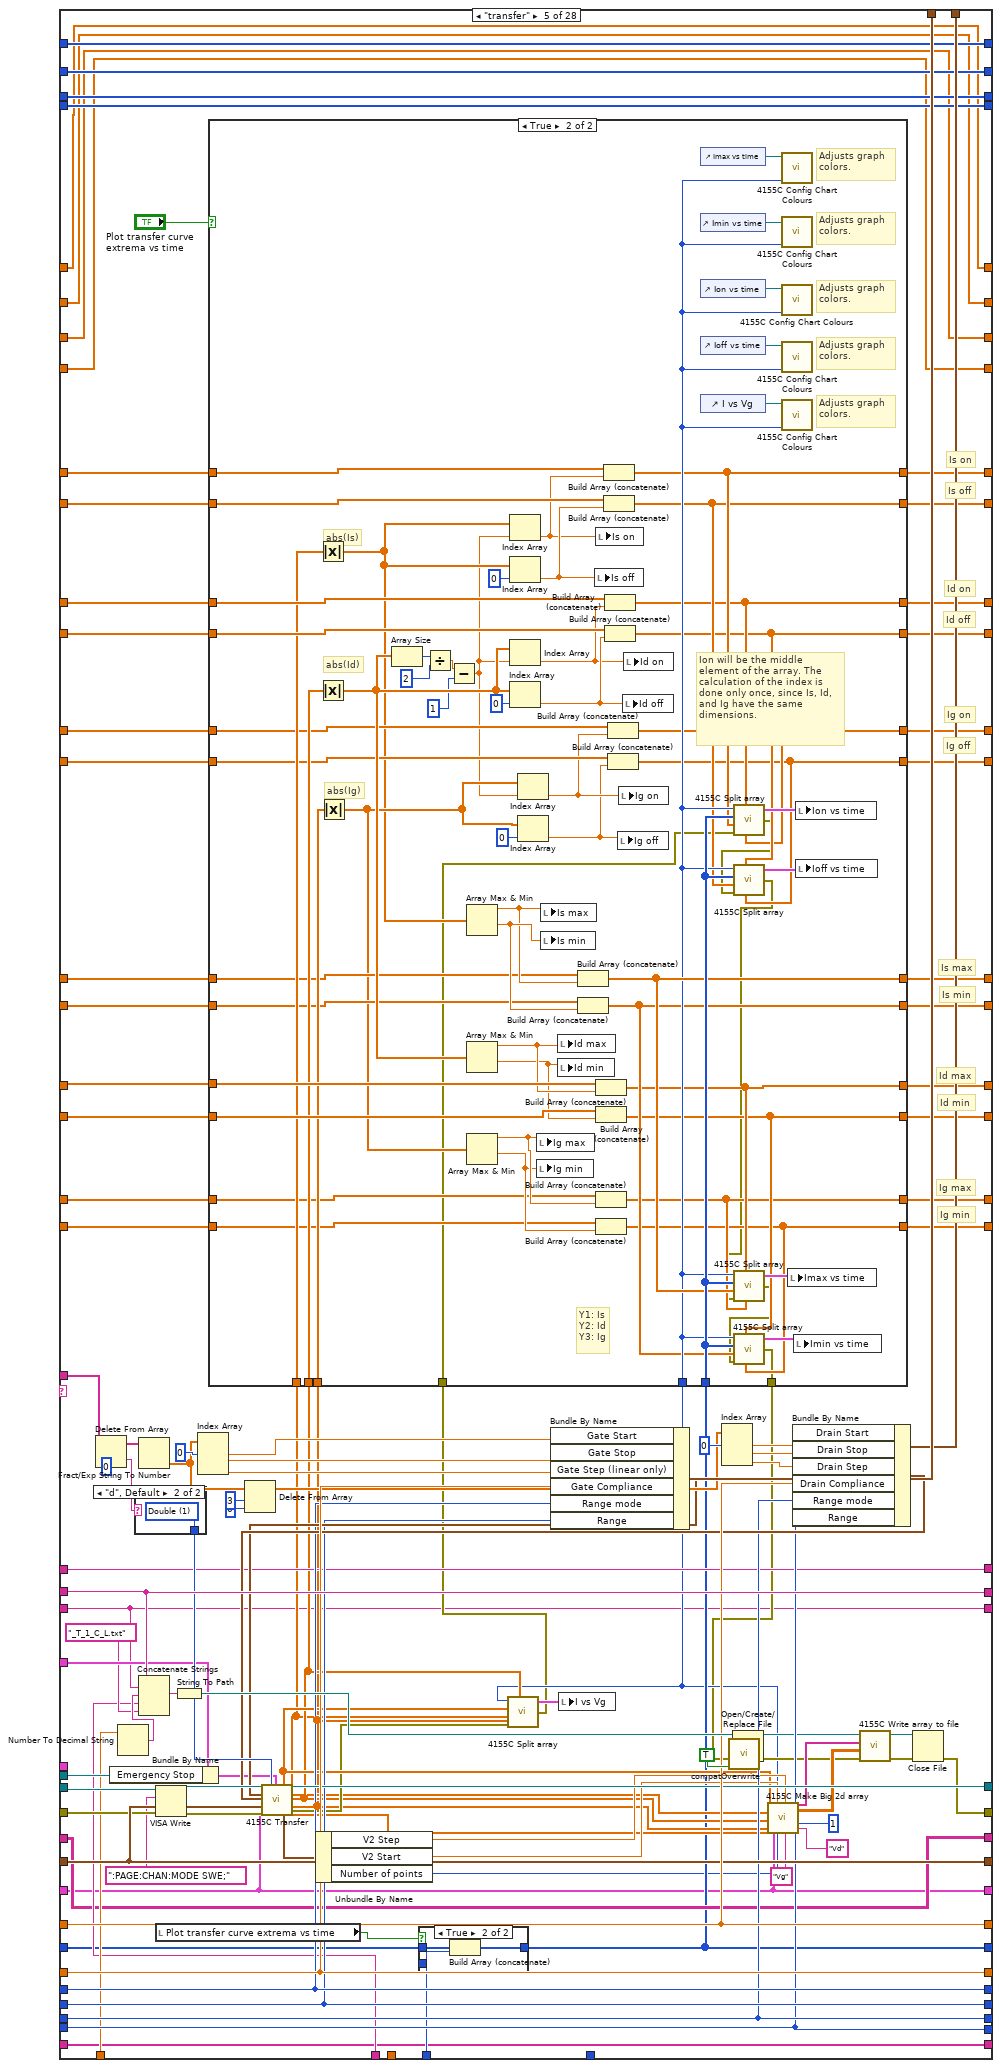
[diagram p11: hidden frame]
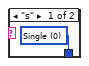
[diagram p14: hidden frame]
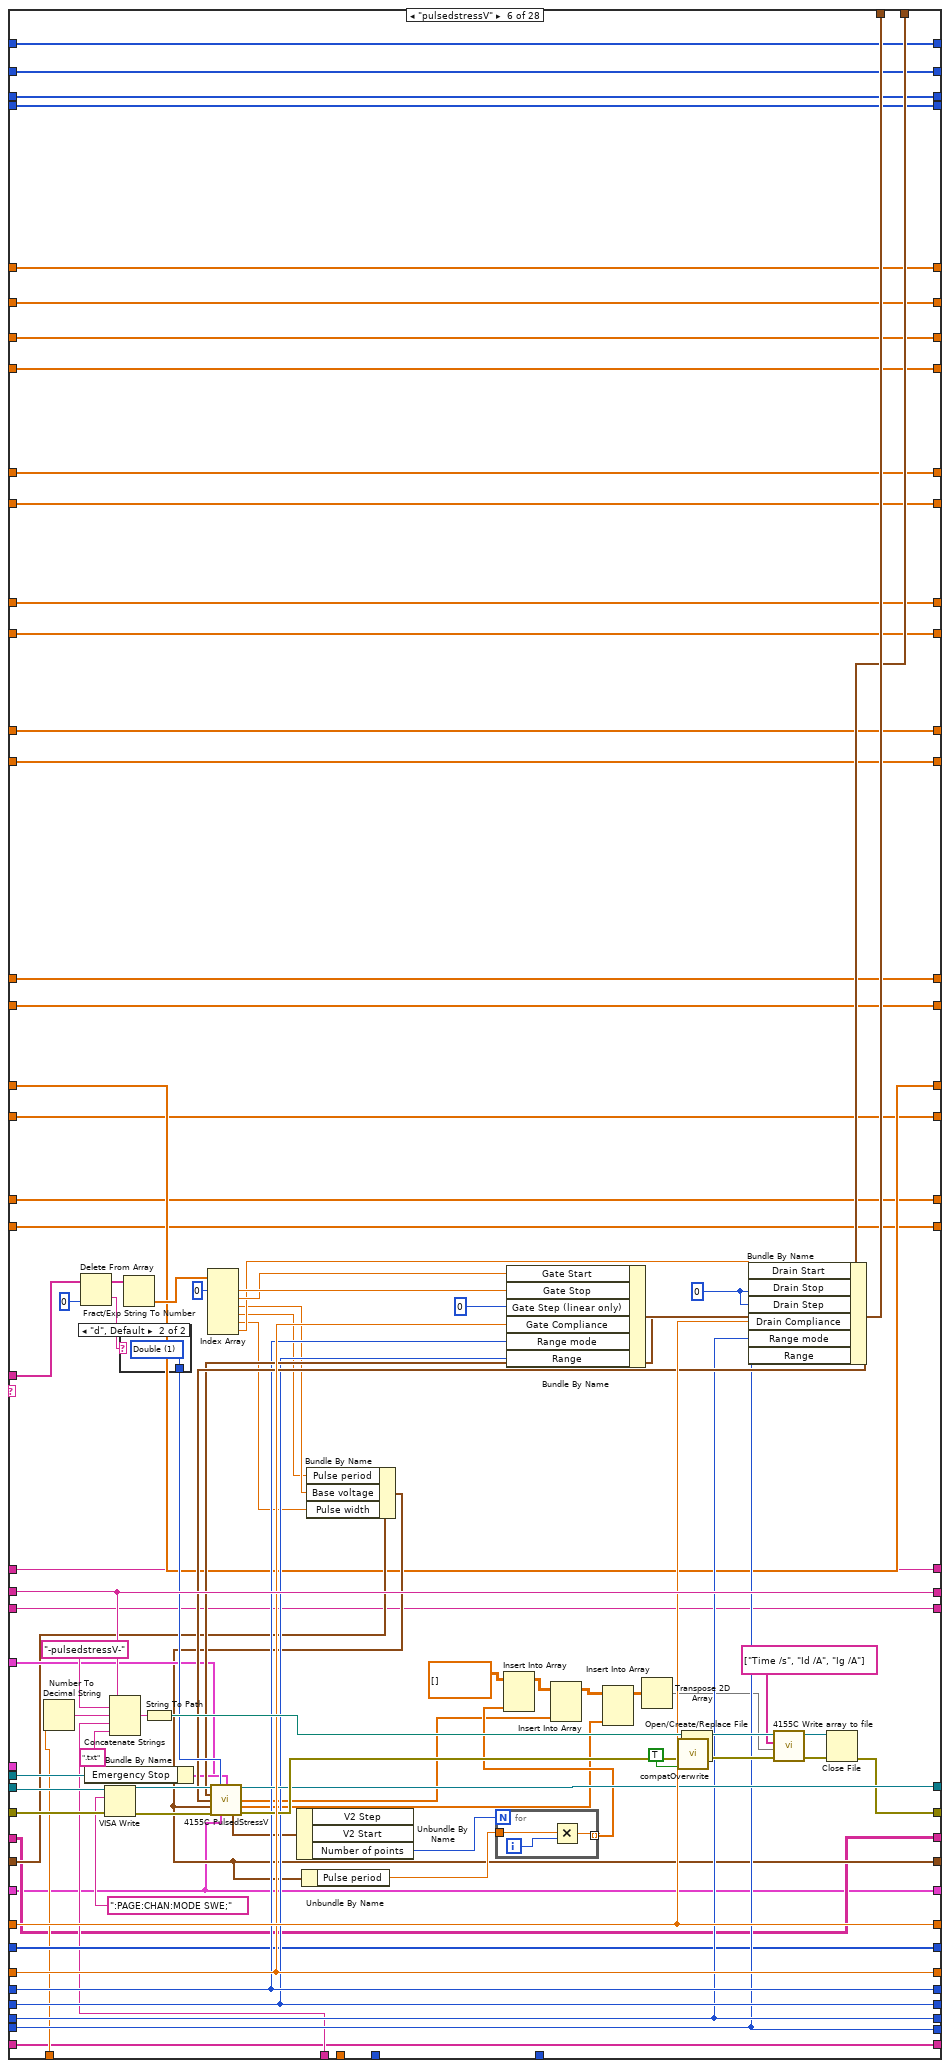
[diagram p15: hidden frame]
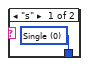
[diagram p16: hidden frame]
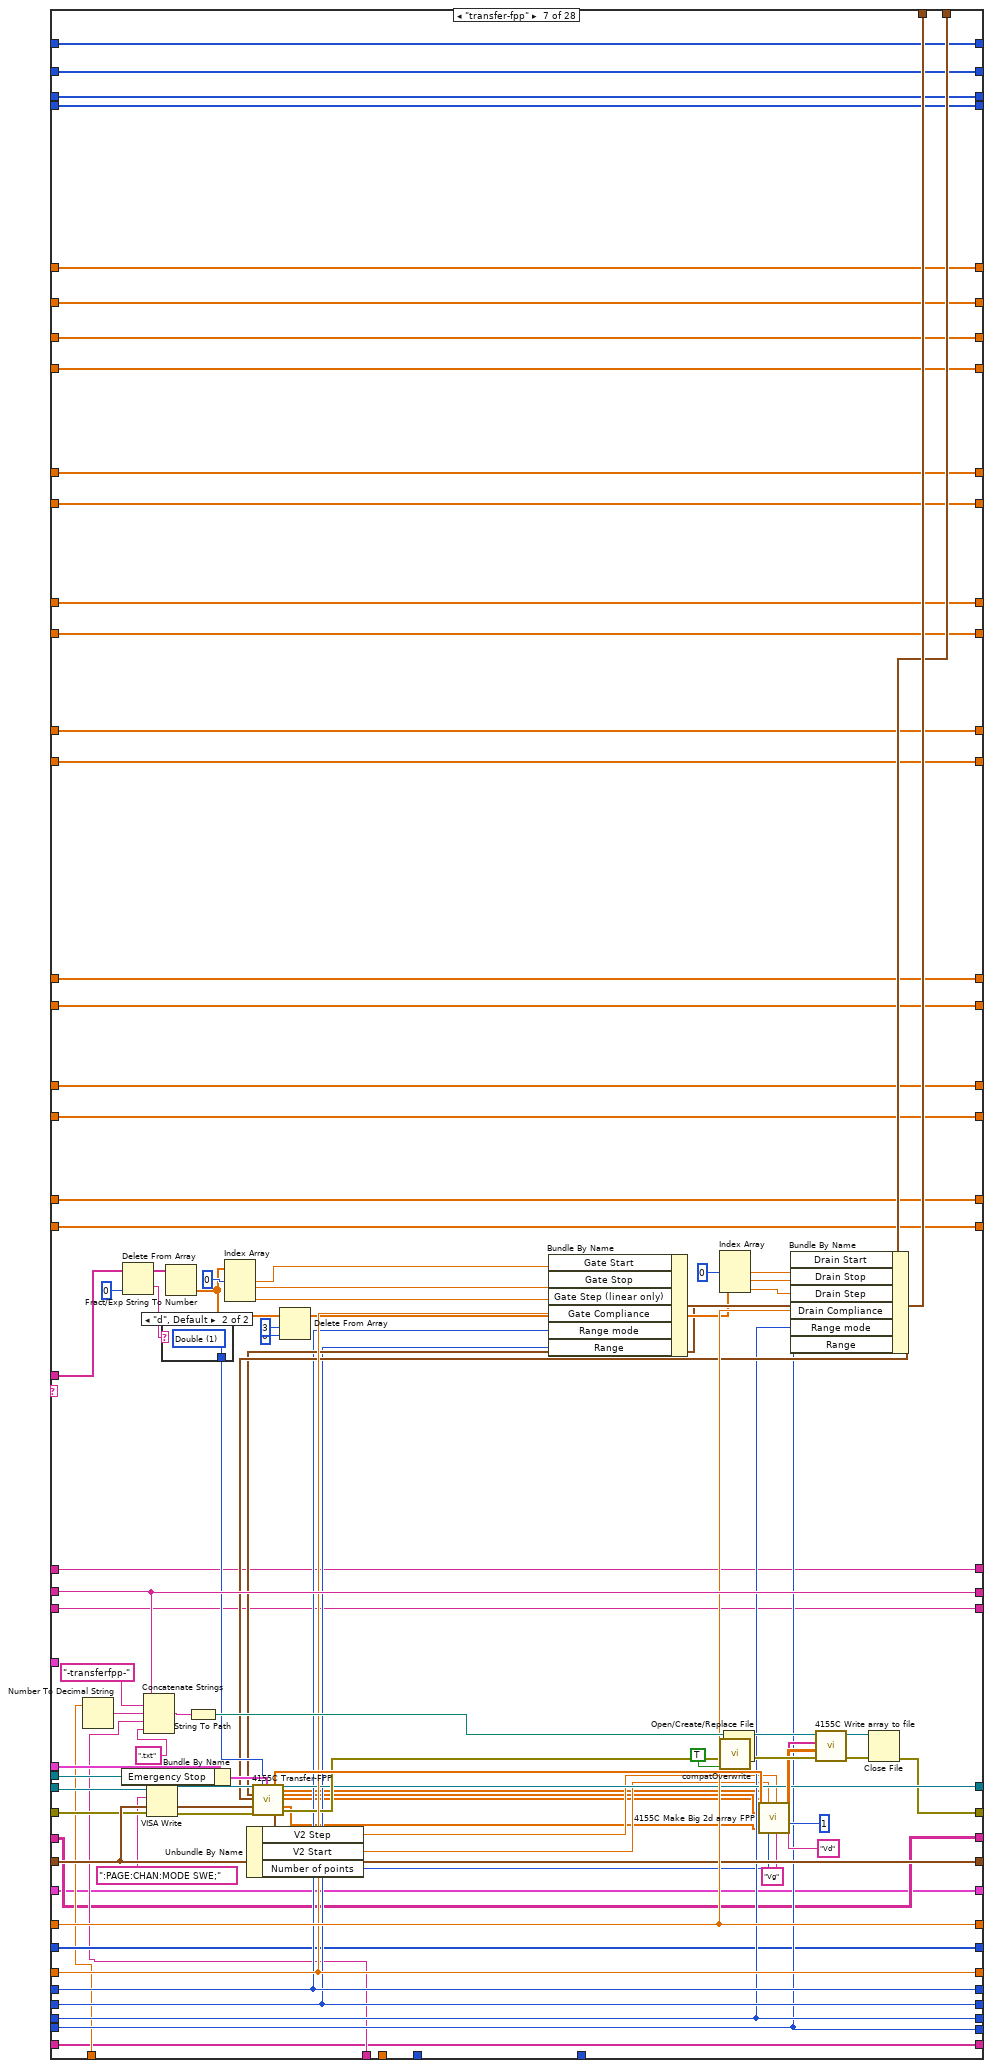
[diagram p17: hidden frame]
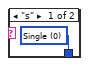
[diagram p18: hidden frame]
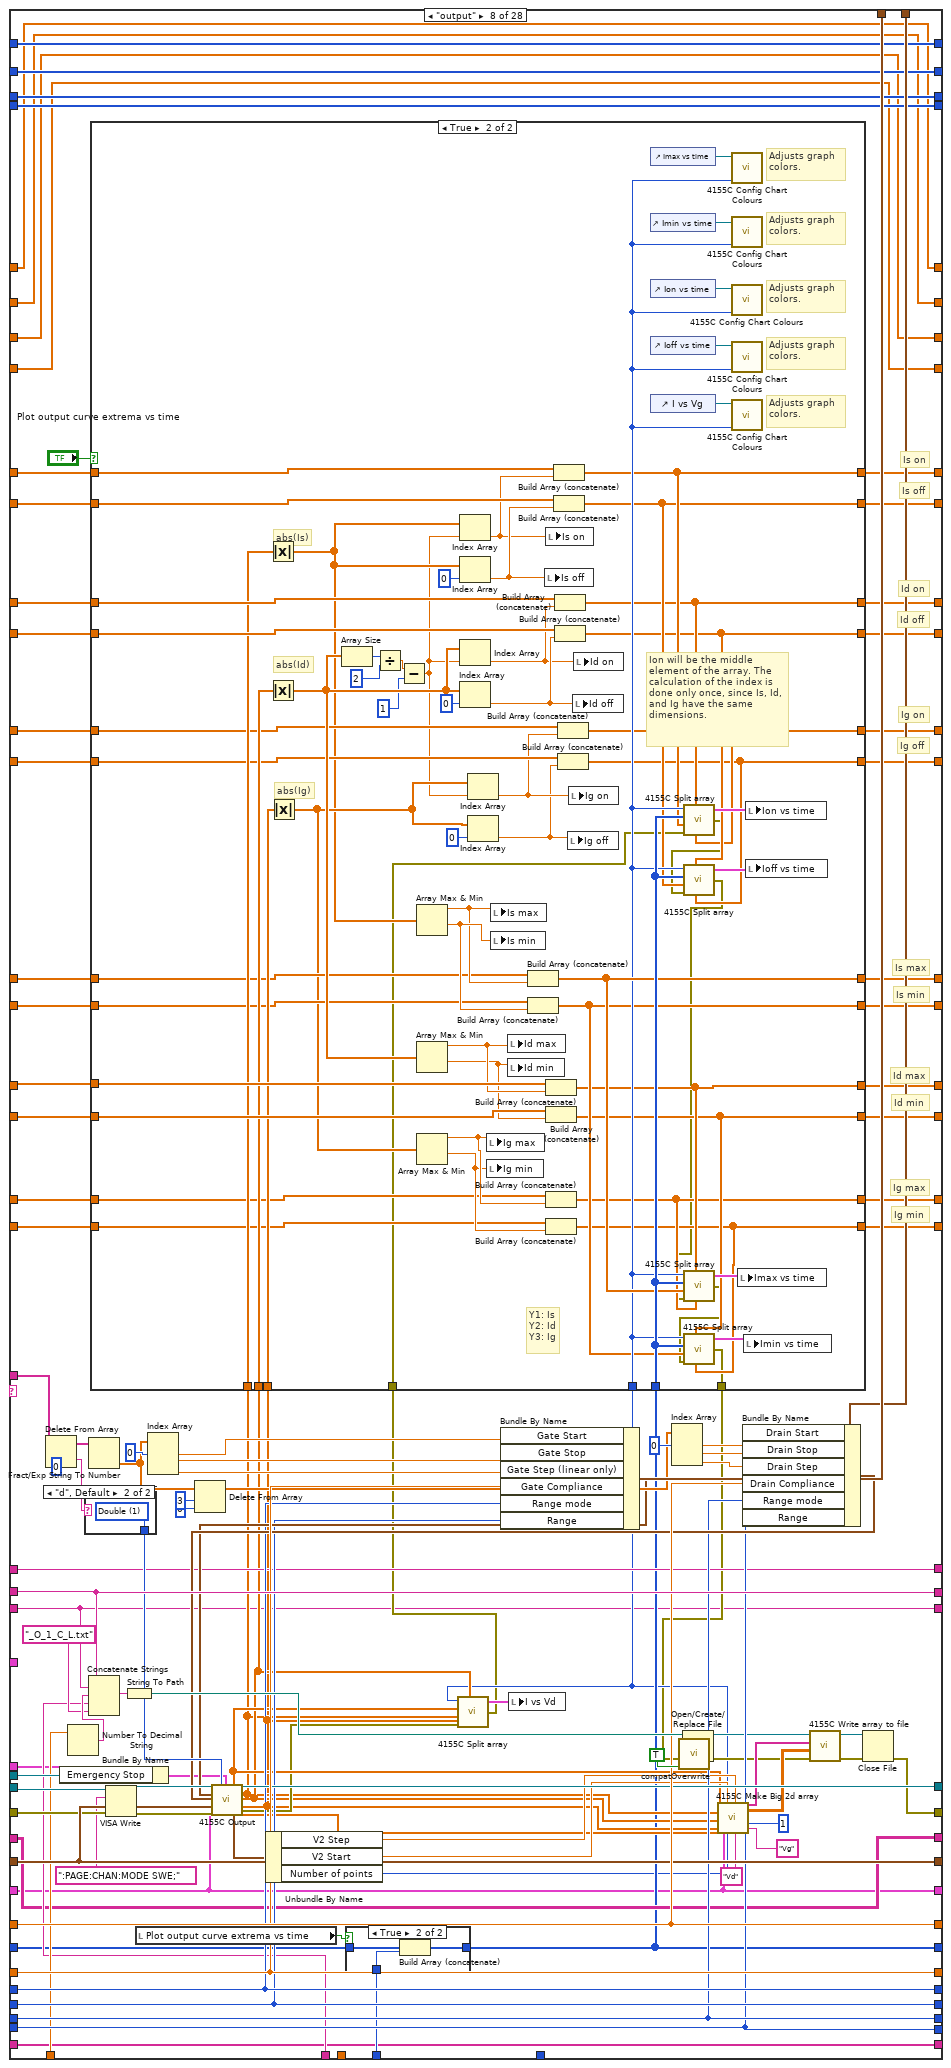
[diagram p19: hidden frame]
diagram:
  w1 = cluster{"Y data in":dbl[], "X data in":dbl[]}[] [] ("I vs Vg")
  w12 = 0.0 ("Is off")
  w13 = 0.0 ("Is on")
  w14 = 0.0 ("Is min")
  w15 = 0.0 ("Is max")
  w63 = u16 1 items=["Reset All", "Partial reset"] ("Type of reset")
  # "Change from previous version:\n\n- Changed bias stress plots so that they always include the entire range."
  # "This is a version specific to the SPM pump."
  # "I add 1 to both the \"total lines\" and the \"line running\" indicators because i and N begin from 0, and the script lines begin from 1."
  # "Bugs:\n\n- If using the \"filename\" command, keep in mind that the arrays of the time-dependent data are not re-initialized inbetween filename changes. \n\n- Do not connect the \"error\" wire of a Split block if it has unconnected terminals! It will halt the program."
  # "Array size"
  # "%s option converts a spreadsheet string to an array of strings."
  # "0: No of rows of array\n1: No of cols"
  # "Dimitrios Simatos\nv. 6.7"
  # "Changes from original textcontrol.vi:\n\n- Timestamp appears in filename.\n- (Only) transfer and output curves are plotted.\n- Communication with serial port.\n- Can execute any command, as all pattern matching functions were replaced. Previously, commands with special LabVIEW characters could not be executed.\n- Replaced write to file function with write to text file.\n- Replaced while loop with for loop.\n- Replaced 4155C \"Save File\" function and now the vi can save time-dependent variables.\n- Added clock with start time control and various units.\n- Changed filepath in which the program is saved.\n- Added a serial output log that keeps a history.\n- Tab control.\n- Addition of specialized serial read/write file for the SPM OEM pump.\n- Added halt and hard stop.\n- Added option for plotting transfer and output curve extrema vs time.\n- Corrected bug of \"itime\" command. The command did not allow for settting the integration time value, it allowed to set the category of the integration time (short, medium, long). If the time value was beyond the range of the category, then the SPA used the closest value allowed, whilst staying in the category. So, if the integration time was changed to long, but the integration time value was a short one, then the SPA would measure using the minimum long integration time value and not the value that the user intended.\n- Added SMU4 command.\n- Added plotting of \"sample\" plots."
  # "Search and replace LF with EOL"
  n1 = Equal?(x="integration time", y=u32 0) -> (x = y?=w64:bool)
  n2 = Select(t="Integration time (short)", s=w64, f="Integration time (long)") -> (s? t:f=w16:dbl)
  n3 = call "4155C Get Filename.vi"("error in (no error)"=errorcluster {"status"=FALSE, "code"=0, "source"=""}) -> ("error out"=w58:errorcluster, "path"=w33:path)  [unwired: 2 in, 1 out]
  "Path" <- w33
  n4 = Bundle By Name(cluster="Timings (overwritten by the Front Panel)", "integration time"="integration time", "Short/Long integration time"=w16) -> (w56:T5)
  n5 = Path To String(path=w33) -> (string=w34:string)
  n6 = Search and Replace String(replace all?=TRUE ("replace all? (F)"), input string="Script", search string="\n", replace string="\r\n") -> (result string=w46:string)  [unwired: 4 in, 3 out]
  n7 = Match Pattern(string=w34, regular expression=".txt") -> (before substring=w29:string)  [unwired: 1 in, 3 out]
  n8 = call "4155C Initialise.vi"("VISA resource name in"=refnum<visa-resource-name> "GPIB0::14::INSTR", "Reset"="Full Reset", "Type of reset"=w63, "error in (no error)"=w58, "VISA Timeout Value"=u32 10000) -> ("VISA Resource Name out"=w57:refnum<visa-resource-name>, "error out"=w5:errorcluster)
  n9 = Concatenate Strings(w29, "Suffix (script)") -> (w28:string)
  n10 = Spreadsheet String To Array(delimiter (Tab)="\r\n", format string="%s", spreadsheet string="Script", array type (2D Dbl)="") -> (array=w37:string[][])
  n11 = String To Path(string=w28) -> (path=w8:path)
  n12 = Array Size(array=w37) -> (size(s)=w41:i32[])
  n13 = Initialize Array("") -> (w21:string[])  [unwired: 1 in]
  n14 = Open/Create/Replace File(file path (use dialog)=w8, error in=w5, operation (0:open)=T8."replace or create with confirmation") -> (refnum out=w7:refnum<file>, error out=w6:errorcluster)  [unwired: 3 in, 1 out]
  n15 = Initialize Array(0 ("element")) -> (w23:i32[])  [unwired: 1 in]
  n16 = Initialize Array("") -> (w19:string[][])  [unwired: 2 in]
  n17 = Initialize Array(0.0 ("element")) -> (w2:dbl[])  [unwired: 1 in]
  n18 = Index Array(array=w41, index=0) -> (element=w39:i32)
  n19 = Write to Text File(file (use dialog)=w7, text=w46, error in=w6) -> (error out=w27:errorcluster)  [unwired: 1 in, 2 out]
  n20 = for {
    N: w39 -> [w207]
    shift-left: "Source/Drain Range" -> [w247]
    shift-right: [w243] -> _
    shift-left: "Source/Drain\nRange mode" -> [w248]
    shift-right: [w244] -> _
    shift-left: "Gate Range" -> [w249]
    shift-right: [w245] -> _
    shift-left: "Gate Range\nmode" -> [w250]
    shift-right: [w246] -> _
    shift-left: "Gate: Compliance" -> [w259]
    shift-right: [w255] -> _
    shift-left: "Drain: Compliance" -> [w260]
    shift-right: [w256] -> _
    shift-left: w56 -> [w261]
    shift-right: [w257] -> w17
    shift-left: w27 -> [w262]
    shift-right: [w75] -> w32
    shift-left: w57 -> [w263]
    shift-right: [w258] -> _
    shift-left: w29 -> [w264]
    shift-right: [w74] -> _
    tunnel: "Panel Controls 2" -> [w241]
    shift-right: [w119] -> _
    shift-left: w2 -> [w240]
    shift-right: [w177] -> _
    shift-left: i32[] [] -> [w236]
    tunnel: w37 -> [w235] mode=indexing
    shift-right: [w118] -> _
    shift-left: w2 -> [w212]
    shift-right: [w150] -> _
    shift-left: w21 -> [w199]
    shift-right: [w178] -> _
    shift-left: w23 -> [w194]
    shift-right: [w160] -> _
    shift-left: w23 -> [w193]
    shift-right: [w192] -> _
    shift-left: "" -> [w191]
    shift-right: [w155] -> _
    shift-left: w23 -> [w175]
    shift-right: [w154] -> _
    shift-left: w23 -> [w159]
    shift-right: [w151] -> _
    shift-left: w19 -> [w153]
    shift-right: [w112] -> _
    shift-left: w2 -> [w140]
    shift-right: [w113] -> _
    shift-left: w2 -> [w139]
    shift-right: [w117] -> _
    shift-left: w2 -> [w128]
    shift-right: [w116] -> _
    shift-left: w2 -> [w127]
    shift-right: [w110] -> _
    shift-left: w2 -> [w126]
    shift-right: [w120] -> _
    shift-left: w2 -> [w125]
    shift-right: [w111] -> _
    shift-left: w2 -> [w124]
    shift-right: [w109] -> _
    shift-left: w2 -> [w123]
    shift-right: [w115] -> _
    shift-left: w2 -> [w122]
    shift-right: [w114] -> _
    shift-left: w2 -> [w121]
    shift-right: [w73] -> _
    shift-left: "Filename (variable part)" -> [w104]
    shift-right: [w101] -> w3
    shift-left: "SMU4" -> [w242]
    shift-right: [w69] -> _
    shift-left: w2 -> [w98]
    shift-right: [w70] -> _
    shift-left: w2 -> [w97]
    shift-right: [w71] -> _
    shift-left: w2 -> [w96]
    shift-right: [w72] -> _
    shift-left: w2 -> [w95]
    i -> [w202]
    stop <- "Interrupt program" stop-if-true
    # "Ig for bias stress plots"
    # "Id for bias stress plots"
    # "Is for bias stress plots"
    # "Time axis for bias stress plots"
    # "Save bias stress curves in file."
    # "Filename prefix"
    # "Is off"
    # "Is on"
    # "Ig off"
    # "Ig on"
    # "Is min"
    # "Is max"
    # "Ig min"
    # "Ig max"
    # "Id min"
    # "Id max"
    # "Id off"
    # "Id on"
    # "Pump status"
    # "Filepath and name"
    # "Pump status"
    # "Limit of command arguments (array columns). Raise if needed."
    # "Serial port data (string)"
    # "Serial port data (table)"
    # "Time array for valve position"
    # "Time array for absolute plunger position"
    # "Valve position"
    # "Absolute plunger position"
    # "Serial port data"
    # "For loop counter"
    # "<-----Equivalent to the 4155C \"Write\" subvi.----->"
    # "Headers"
    # "Save transfer curves in file."
    # "Filepath and name"
    # "Save time-dependent data."
    # "Use the time offset if your measurements do not start at t=0."
    # "Time for Imax, Imin, Ion, Ioff"
    # "Rest of elements of command"
    # "First element of command\n(case select)"
    n21 = Add(x=w202, y=1) -> (x+y=→"Line running":i32)
    n22 = Add(x=w207, y=1) -> (x+y=→"Total lines":i32)
    n23 = Index Array(array=w235, index=0 ("line index")) -> (element=w230:string)
    "Command running:" <- w230
    n24 = control-ref of="Interrupt scan"() -> (w254:refnum<vi>)
    n25 = Spreadsheet String To Array(delimiter (Tab)=" ", format string="%s", spreadsheet string=w230, array type (2D Dbl)=string[] []) -> (array=w228:string[])
    n26 = Delete From Array(array=w228, index=0) -> (deleted portion=w141:string, array with subset deleted=w227:string[])  [unwired: 1 in]
    n27 = call "Elapsed Time"("Reset"="Reset", "Auto Reset"="Auto Reset") -> ("Elapsed Time (s)"=w237:dbl)  [unwired: 10 in, 7 out]
    n28 = case shown="0, Default" "Time Units" {
      tunnel: ["-sec" "-min" "-h"] -> w238
      tunnel: [w268 w272 w275] -> w208
      tunnel: w237 -> [w268 w271 w276]
      frame 0, Default {
      }
      frame 1 {
        n29 = Divide(x=w271, y=60.0) -> (x/y=w272:dbl)
      }
      frame 2 {
        n30 = Divide(x=w276, y=3600.0) -> (x/y=w275:dbl)
      }
    }
    n31 = Add(x=w208, y="Time Offset") -> (x+y=w99:dbl)
    n32 = To Long Integer(number=w99) -> (32bit integer=w100:i32)
    "Elapsed Time" <- w100
    n33 = case shown="\"sample\"" w141 {
      tunnel: w227 -> [w318 w361 w403 w411 w551 w663 w813 w937 w1103 w1135 w1220 w1271 w1320 w1365 w1403 _ _ w1607 w1732 _ w1845 w1913 w1979 w2073 w2159 w2203 w2278 w2337]
      tunnel: w264 -> [w313 w357 w401 w433 w558 w727 w821 w944 w1111 w1158 w1209 w1263 w1313 w1359 w1396 w1439 w1505 w1533 w1714 w1769 w1832 w1900 w1967 w2067 w2155 w2205 w2280 w2339]
      tunnel: w263 -> [w312 w356 w392 w431 w529 w712 w790 w915 w1079 w1159 w1210 w1264 w1314 w1360 w1397 w1444 w1507 w1612 w1738 w1773 w1851 w1919 w1985 w2079 w2113 w2209 w2284 w2341]
      tunnel: w262 -> [w311 w355 w391 w430 w528 w711 w789 w914 w1076 w1160 w1211 w1265 w1315 w1361 w1398 w1443 w1478 w1611 w1737 w1772 w1850 w1918 w1984 w2078 w2112 w2208 w2283 w2342]
      tunnel: w261 -> [w310 w354 w400 w428 w554 w688 w817 w940 w1107 w1168 w1219 w1262 w1312 w1358 w1395 w1442 w1502 w1582 w1706 w1778 w1825 w1893 w1960 w2066 w2154 w2210 w2285 w2344]
      tunnel: w260 -> [w309 w353 w399 w427 w556 w725 w819 w942 w1109 w1167 w1218 w1270 w1319 w1364 w1402 w1441 w1487 w1610 w1736 w1781 w1849 w1917 w1983 w2077 w2163 w2211 w2286 w2345]
      tunnel: w259 -> [w308 w352 w398 w425 w555 w724 w818 w941 w1108 w1166 w1217 w1269 w1318 w1363 w1401 w1440 w1488 w1590 w1715 w1780 w1833 w1901 w1968 w2068 w2156 w2213 w2287 w2347]
      tunnel: [w312 w356 w390 w431 w553 w722 w815 w939 w1105 w1159 w1210 w1264 w1314 w1360 w1397 w1444 w1507 w1583 w1688 w1771 w1826 w1894 w1961 w2019 w2115 w2209 w2284 w2341] -> w258
      tunnel: [w311 w355 w389 w430 w552 w721 w814 w938 w1104 w1160 w1211 w1265 w1315 w1361 w1398 w1443 w1477 w1591 w1689 w1770 w1834 w1902 w1969 w2018 w2114 w2207 w2282 w2342] -> w174
      tunnel: [w310 w354 w400 w428 w554 w684 w817 w940 w1107 w1161 w1212 w1262 w1312 w1358 w1395 w1442 w1502 w1582 w1706 w1778 w1825 w1893 w1960 w2066 w2154 w2210 w2285 w2344] -> w257
      tunnel: [w309 w353 w399 w427 w556 w725 w819 w942 w1109 w1167 w1218 w1270 w1319 w1364 w1402 w1441 w1487 w1610 w1736 w1781 w1849 w1917 w1983 w2077 w2163 w2211 w2286 w2345] -> w256
      tunnel: [w308 w352 w398 w425 w555 w724 w818 w941 w1108 w1166 w1217 w1269 w1318 w1363 w1401 w1440 w1488 w1590 w1715 w1780 w1833 w1901 w1968 w2068 w2156 w2213 w2287 w2347] -> w255
      tunnel: [w313 w357 w401 w433 w558 w727 w821 w944 w1111 w1158 w1209 w1263 w1313 w1359 w1396 w1439 w1505 w1533 w1714 w1769 w1832 w1900 w1967 w2067 w2155 w2205 w2280 w2339] -> w74
      tunnel: w254 -> [_ _ _ _ w560 w731 w826 w946 w1115 _ _ _ _ _ _ _ _ w1587 w1711 _ w1831 w1899 w1966 w2039 w2131 _ _ _]
      tunnel: "Gate" -> [_ _ _ _ w538 w715 w800 w924 w1090 _ _ _ _ _ _ _ _ _ _ _ _ _ _ _ _ _ _ _]
      tunnel: "Drain 2" -> [_ _ _ _ w537 w714 w799 w923 w1089 _ _ _ _ _ _ _ _ _ _ _ _ _ _ _ _ _ _ _]
      tunnel: "Panel Controls" -> [_ _ _ _ _ _ w798 w844 w1088 _ _ _ _ _ _ _ _ _ _ _ _ _ _ _ _ _ _ _]
      tunnel: w250 -> [w307 w351 w397 w424 w522 w705 w783 w908 w1074 w1165 w1216 _ w1311 w1357 w1394 w1438 w1489 w1578 w1702 w1774 w1821 w1889 w1956 w2062 w2150 w2214 w2288 w2348]
      tunnel: w249 -> [w306 w350 w396 w423 w521 w704 w782 w907 w1073 w1164 w1215 w1268 _ w1348 w1400 w1437 w1490 w1579 w1703 w1775 w1822 w1890 w1957 w2063 w2151 w2215 w2289 w2349]
      tunnel: w248 -> [w305 w349 w395 w422 w520 w703 w781 w906 w1072 w1163 w1214 w1267 w1317 w1362 _ w1436 w1491 w1580 w1704 w1776 w1823 w1891 w1958 w2064 w2152 w2216 w2290 w2350]
      tunnel: w247 -> [w304 w348 w394 w421 w519 w702 w780 w905 w1075 w1162 w1213 w1266 w1316 _ w1399 w1435 w1492 w1581 w1705 w1777 w1824 w1892 w1959 w2065 w2153 w2217 w2291 w2351]
      tunnel: [w307 w351 w397 w424 w522 w705 w783 w908 w1074 w1165 w1216 w1261 w1311 w1357 w1394 w1438 w1489 w1578 w1702 w1774 w1821 w1889 w1956 w2062 w2150 w2214 w2288 w2348] -> w246
      tunnel: [w306 w350 w396 w423 w521 w704 w782 w907 w1073 w1164 w1215 w1268 w1303 w1348 w1400 w1437 w1490 w1579 w1703 w1775 w1822 w1890 w1957 w2063 w2151 w2215 w2289 w2349] -> w245
      tunnel: [w305 w349 w395 w422 w520 w703 w781 w906 w1072 w1163 w1214 w1267 w1317 w1362 w1393 w1436 w1491 w1580 w1704 w1776 w1823 w1891 w1958 w2064 w2152 w2216 w2290 w2350] -> w244
      tunnel: [w304 w348 w394 w421 w519 w702 w780 w905 w1075 w1162 w1213 w1266 w1316 w1349 w1399 w1435 w1492 w1581 w1705 w1777 w1824 w1892 w1959 w2065 w2153 w2217 w2291 w2351] -> w243
      tunnel: w242 -> [w282 w323 w366 _ w455 w651 w746 w841 w1037 w1132 w1186 w1239 w1281 w1326 w1371 w1413 w1449 w1555 w1662 w1747 w1786 w1858 w1926 w1992 w2084 w2168 w2222 w2335]
      tunnel: w241 -> [_ _ _ _ w513 w699 _ _ _ _ _ _ _ _ _ _ _ _ _ _ _ _ _ _ _ _ _ _]
      tunnel: [w303 w344 w387 w438 w470 w676 w770 w857 w1061 w1157 w1207 w1260 w1302 w1347 w1392 w1434 w1473 w1544 w1667 w1768 w1810 w1882 w1950 w2016 w2108 w2206 w2281 w2356] -> w119
      tunnel: w240 -> [w303 w344 w387 w438 w510 w676 w770 w897 w1061 w1157 w1207 w1260 w1302 w1347 w1392 w1434 w1473 w1551 w1667 w1768 w1810 w1882 w1950 w2016 w2108 w2206 w2281 w2356]
      tunnel: w99 -> [_ _ _ _ w509 w673 w768 w896 w1058 _ _ _ _ _ _ _ w1471 w1571 w1684 _ w1807 w1879 w1947 w2013 w2104 _ _ _]
      tunnel: w238 -> [_ _ _ _ w506 w672 w766 w893 w1057 _ _ _ _ _ _ _ w1469 w1569 w1683 _ w1806 w1878 w1946 w2012 w2105 _ w2249 _]
      tunnel: w100 -> [_ _ _ _ w502 _ _ w889 _ _ _ _ _ _ _ _ _ _ _ _ _ _ _ _ _ _ w2252 _]
      tunnel: [w302 w343 w386 w426 w474 w675 w769 w861 w1060 w1156 w1206 w1259 w1301 w1346 w1391 w1433 w1472 w1536 w1686 w1767 w1809 w1881 w1949 w2015 w2107 w2212 w2261 w2346] -> w177
      tunnel: w236 -> [w302 w343 w386 w426 w505 w675 w769 w892 w1060 w1156 w1206 w1259 w1301 w1346 w1391 w1433 w1472 w1540 w1686 w1767 w1809 w1881 w1949 w2015 w2107 w2212 w2261 w2346]
      tunnel: [w301 w342 w385 w437 w469 w671 w765 w856 w1056 w1155 w1205 w1258 w1300 w1345 w1390 w1432 w1468 w1543 w1666 w1766 w1805 w1877 w1945 w2011 w2103 w2201 w2277 w2355] -> w118
      tunnel: w212 -> [w301 w342 w385 w437 w501 w671 w765 w888 w1056 w1155 w1205 w1258 w1300 w1345 w1390 w1432 w1468 w1550 w1666 w1766 w1805 w1877 w1945 w2011 w2103 w2201 w2277 w2355]
      tunnel: [w300 w341 w384 w420 w494 w670 w764 w881 w1055 w1154 w1204 w1257 w1299 w1344 w1389 w1431 w1467 w1568 w1682 w1765 w1804 w1876 w1944 w2010 w2102 w2200 w2276 w2352] -> w150
      tunnel: w199 -> [w300 w341 w384 w420 w494 w670 w764 w881 w1055 w1154 w1204 w1257 w1299 w1344 w1389 w1431 w1467 w1568 w1682 w1765 w1804 w1876 w1944 w2010 w2102 w2199 w2250 w2352]
      tunnel: [w299 w340 w383 w448 w493 w669 w763 w880 w1054 w1153 w1203 w1256 w1298 w1343 w1388 w1430 w1466 w1567 w1681 w1764 w1803 w1875 w1943 w2009 w2101 w2185 w2263 w2366] -> w178
      tunnel: w194 -> [w299 w340 w383 w448 w493 w669 w763 w880 w1054 w1153 w1203 w1256 w1298 w1343 w1388 w1430 w1466 w1567 w1681 w1764 w1803 w1875 w1943 w2009 w2101 w2185 w2262 w2366]
      tunnel: [w298 w339 w382 w450 w492 w668 w762 w879 w1053 w1152 w1202 w1255 w1297 w1342 w1387 w1429 w1465 w1566 w1680 w1763 w1802 w1874 w1942 w2008 w2100 w2184 w2245 w2368] -> w160
      tunnel: w193 -> [w298 w339 w382 w450 w492 w668 w762 w879 w1053 w1152 w1202 w1255 w1297 w1342 w1387 w1429 w1465 w1566 w1680 w1763 w1802 w1874 w1942 w2008 w2100 w2184 w2243 w2368]
      tunnel: [w297 w338 w381 w434 w491 w667 w761 w878 w1052 w1151 w1201 w1254 w1296 w1341 w1386 w1428 w1464 w1565 w1679 w1762 w1801 w1873 w1941 w2007 w2099 w2183 w2242 w2340] -> w192
      tunnel: w191 -> [w297 w338 w381 w434 w491 w667 w761 w878 w1052 w1151 w1201 w1254 w1296 w1341 w1386 w1428 w1464 w1565 w1679 w1762 w1801 w1873 w1941 w2007 w2099 w2183 w2253 w2340]
      tunnel: w100 -> [_ _ _ _ _ _ _ _ _ _ _ _ _ _ _ _ _ _ _ _ _ _ _ _ _ _ w2241 _]
      tunnel: w175 -> [w296 w337 w380 w449 w490 w666 w760 w877 w1051 w1150 w1200 w1253 w1295 w1340 w1385 w1427 w1463 w1564 w1678 w1761 w1800 w1872 w1940 w2006 w2098 w2182 w2240 w2367]
      tunnel: [w296 w337 w380 w449 w490 w666 w760 w877 w1051 w1150 w1200 w1253 w1295 w1340 w1385 w1427 w1463 w1564 w1678 w1761 w1800 w1872 w1940 w2006 w2098 w2182 w2239 w2367] -> w155
      tunnel: [w295 w336 w379 w447 w489 w665 w759 w876 w1050 w1149 w1199 w1252 w1294 w1339 w1384 w1426 w1462 w1563 w1677 w1760 w1799 w1871 w1939 w2005 w2097 w2181 w2238 w2365] -> w154
      tunnel: w159 -> [w295 w336 w379 w447 w489 w665 w759 w876 w1050 w1149 w1199 w1252 w1294 w1339 w1384 w1426 w1462 w1563 w1677 w1760 w1799 w1871 w1939 w2005 w2097 w2181 w2237 w2365]
      tunnel: [w294 w335 w378 w429 w488 w664 w758 w875 w1049 w1148 w1198 w1251 w1293 w1338 w1383 w1425 w1461 w1562 w1676 w1759 w1798 w1870 w1938 w2004 w2096 w2180 w2235 w2343] -> w151
      tunnel: w153 -> [w294 w335 w378 w429 w488 w664 w758 w875 w1049 w1148 w1198 w1251 w1293 w1338 w1383 w1425 w1461 w1562 w1676 w1759 w1798 w1870 w1938 w2004 w2096 w2180 w2234 w2343]
      tunnel: [w292 w333 w376 w443 w463 w661 w756 w850 w1047 w1146 w1197 w1250 w1291 w1336 w1381 w1423 w1459 w1561 w1675 w1758 w1797 w1869 w1936 w2003 w2095 w2179 w2233 w2361] -> w112
      tunnel: w140 -> [w292 w333 w376 w443 w487 w661 w756 w874 w1047 w1146 w1197 w1250 w1291 w1336 w1381 w1423 w1459 w1561 w1675 w1758 w1797 w1869 w1936 w2003 w2095 w2179 w2233 w2361]
      tunnel: [w293 w334 w377 w444 w464 w662 w757 w851 w1048 w1147 w1196 w1249 w1292 w1337 w1382 w1424 w1460 w1560 w1674 w1757 w1796 w1868 w1937 w2002 w2094 w2178 w2232 w2362] -> w113
      tunnel: w139 -> [w293 w334 w377 w444 w486 w662 w757 w873 w1048 w1147 w1196 w1249 w1292 w1337 w1382 w1424 w1460 w1560 w1674 w1757 w1796 w1868 w1937 w2002 w2094 w2178 w2232 w2362]
      tunnel: [w285 w326 w369 w436 w468 w658 w754 w855 w1045 w1139 w1194 w1247 w1289 w1334 w1379 w1421 w1452 w1542 w1665 w1756 w1789 w1861 w1929 w1995 w2089 w2171 w2231 w2354] -> w117
      tunnel: w128 -> [w285 w326 w369 w436 w482 w658 w754 w869 w1045 w1139 w1194 w1247 w1289 w1334 w1379 w1421 w1452 w1549 w1665 w1756 w1789 w1861 w1929 w1995 w2089 w2171 w2231 w2354]
      tunnel: [w284 w325 w368 w435 w467 w659 w755 w854 w1046 w1138 w1195 w1248 w1290 w1335 w1380 w1422 w1451 w1541 w1664 w1755 w1788 w1860 w1928 w1994 w2088 w2170 w2230 w2353] -> w116
      tunnel: w127 -> [w284 w325 w368 w435 w481 w659 w755 w868 w1046 w1138 w1195 w1248 w1290 w1335 w1380 w1422 w1451 w1548 w1664 w1755 w1788 w1860 w1928 w1994 w2088 w2170 w2230 w2353]
      tunnel: [w287 w328 w371 w440 w473 w657 w752 w860 w1043 w1144 w1192 w1245 w1287 w1332 w1377 w1419 w1454 w1546 w1669 w1750 w1791 w1863 w1931 w1997 w2087 w2175 w2228 w2358] -> w110
      tunnel: w126 -> [w287 w328 w371 w440 w480 w657 w752 w867 w1043 w1144 w1192 w1245 w1287 w1332 w1377 w1419 w1454 w1553 w1669 w1750 w1791 w1863 w1931 w1997 w2087 w2175 w2228 w2358]
      tunnel: [w286 w327 w370 w439 w471 w660 w753 w858 w1044 w1145 w1193 w1246 w1288 w1333 w1378 w1420 w1453 w1545 w1668 w1749 w1790 w1862 w1930 w1996 w2086 w2174 w2229 w2357] -> w120
      tunnel: w125 -> [w286 w327 w370 w439 w479 w660 w753 w866 w1044 w1145 w1193 w1246 w1288 w1333 w1378 w1420 w1453 w1552 w1668 w1749 w1790 w1862 w1930 w1996 w2086 w2174 w2229 w2357]
      tunnel: [w289 w330 w373 w442 w462 w656 w750 w849 w1041 w1142 w1190 w1243 w1285 w1330 w1375 w1417 w1456 w1557 w1671 w1752 w1793 w1865 w1933 w1999 w2091 w2177 w2226 w2360] -> w111
      tunnel: w124 -> [w289 w330 w373 w442 w478 w656 w750 w865 w1041 w1142 w1190 w1243 w1285 w1330 w1375 w1417 w1456 w1557 w1671 w1752 w1793 w1865 w1933 w1999 w2091 w2177 w2226 w2360]
      tunnel: [w288 w329 w372 w441 w461 w655 w751 w848 w1042 w1143 w1191 w1244 w1286 w1331 w1376 w1418 w1455 w1556 w1670 w1751 w1792 w1864 w1932 w1998 w2090 w2176 w2227 w2359] -> w109
      tunnel: w123 -> [w288 w329 w372 w441 w477 w655 w751 w864 w1042 w1143 w1191 w1244 w1286 w1331 w1376 w1418 w1455 w1556 w1670 w1751 w1792 w1864 w1932 w1998 w2090 w2176 w2227 w2359]
      tunnel: [w291 w332 w375 w446 w466 w654 w748 w853 w1039 w1140 w1188 w1241 w1283 w1328 w1373 w1415 w1458 w1559 w1673 w1754 w1795 w1867 w1935 w2001 w2093 w2173 w2224 w2364] -> w115
      tunnel: w122 -> [w291 w332 w375 w446 w476 w654 w748 w863 w1039 w1140 w1188 w1241 w1283 w1328 w1373 w1415 w1458 w1559 w1673 w1754 w1795 w1867 w1935 w2001 w2093 w2173 w2224 w2364]
      tunnel: [w290 w331 w374 w445 w465 w653 w749 w852 w1040 w1141 w1189 w1242 w1284 w1329 w1374 w1416 w1457 w1558 w1672 w1753 w1794 w1866 w1934 w2000 w2092 w2172 w2225 w2363] -> w114
      tunnel: w121 -> [w290 w331 w374 w445 w475 w653 w749 w862 w1040 w1141 w1189 w1242 w1284 w1329 w1374 w1416 w1457 w1558 w1672 w1753 w1794 w1866 w1934 w2000 w2092 w2172 w2225 w2363]
      tunnel: w104 -> [w283 w324 w367 w432 w458 w652 w747 w845 w1038 w1137 w1187 w1240 w1282 w1327 w1372 w1414 w1450 w1532 w1663 w1748 w1787 w1859 w1927 w1993 w2085 w2169 w2223 _]
      tunnel: [w283 w324 w367 w432 w458 w652 w747 w845 w1038 w1137 w1187 w1240 w1282 w1327 w1372 w1414 w1450 w1532 w1663 w1748 w1787 w1859 w1927 w1993 w2085 w2169 w2223 w2336] -> w73
      tunnel: [w282 w323 w366 w410 w455 w651 w746 w841 w1037 w1132 w1186 w1239 w1281 w1326 w1371 w1413 w1449 w1555 w1662 w1747 w1786 w1858 w1926 w1992 w2084 w2168 w2222 w2335] -> w101
      tunnel: w99 -> [_ _ _ _ _ _ _ _ _ _ _ _ _ _ _ _ _ w1531 _ _ _ _ _ _ _ _ _ _]
      tunnel: [w281 w322 w365 w409 w454 w650 w745 w840 w1036 w1131 w1185 w1238 w1280 w1325 w1370 w1412 w1448 w1515 w1661 w1746 w1785 w1857 w1925 w1991 w2083 w2167 w2221 w2334] -> w69
      tunnel: [w280 w321 w364 w408 w453 w649 w744 w839 w1035 w1130 w1184 w1237 w1279 w1324 w1369 w1411 w1447 w1514 w1660 w1745 w1784 w1856 w1924 w1990 w2082 w2166 w2220 w2333] -> w70
      tunnel: [w279 w320 w363 w407 w452 w648 w743 w838 w1034 w1129 w1183 w1236 w1278 w1323 w1368 w1410 w1446 w1516 w1659 w1744 w1783 w1855 w1923 w1989 w2081 w2165 w2219 w2332] -> w71
      tunnel: [w278 w319 w362 w406 w451 w647 w742 w837 w1033 w1128 w1182 w1235 w1277 w1322 w1367 w1409 w1445 w1513 w1658 w1743 w1782 w1854 w1922 w1988 w2080 w2164 w2218 w2331] -> w72
      tunnel: w98 -> [w281 w322 w365 w409 w454 w650 w745 w840 w1036 w1131 w1185 w1238 w1280 w1325 w1370 w1412 w1448 w1512 w1661 w1746 w1785 w1857 w1925 w1991 w2083 w2167 w2221 w2334]
      tunnel: w97 -> [w280 w321 w364 w408 w453 w649 w744 w839 w1035 w1130 w1184 w1237 w1279 w1324 w1369 w1411 w1447 w1511 w1660 w1745 w1784 w1856 w1924 w1990 w2082 w2166 w2220 w2333]
      tunnel: w96 -> [w279 w320 w363 w407 w452 w648 w743 w838 w1034 w1129 w1183 w1236 w1278 w1323 w1368 w1410 w1446 w1510 w1659 w1744 w1783 w1855 w1923 w1989 w2081 w2165 w2219 w2332]
      tunnel: w95 -> [w278 w319 w362 w406 w451 w647 w742 w837 w1033 w1128 w1182 w1235 w1277 w1322 w1367 w1409 w1445 w1509 w1658 w1743 w1782 w1854 w1922 w1988 w2080 w2164 w2218 w2331]
      frame "wait" {
        n34 = Index Array(array=w318, index=0 ("Index")) -> (element=w316:string)
        n35 = Decimal String To Number(string=w316, default (0L)=u32 0) -> (number=w315:u32)  [unwired: 1 in, 1 out]
        n36 = Wait (ms)(milliseconds to wait=w315) -> ()  [unwired: 1 out]
      }
      frame "wait-min" {
        n37 = Index Array(array=w361, index=0 ("Index")) -> (element=w359:string)
        n38 = Decimal String To Number(string=w359, default (0L)=u32 0) -> (number=w347:u32)  [unwired: 1 in, 1 out]
        n39 = Multiply(x=w347, y=u32 60000) -> (x*y=w346:u32)
        n40 = Wait (ms)(milliseconds to wait=w346) -> ()  [unwired: 1 out]
      }
      frame "standby" {
        n41 = Index Array(array=w403, index=0 ("Index")) -> (element=w393:string)
        n42 = case shown="\"off\", Default" w393 {
          tunnel: [":PAGE:SCON:STAN 0" ":PAGE:SCON:STAN 1"] -> w388
          frame "off", Default {
          }
          frame "on" {
          }
        }
        n43 = VISA Write(VISA resource name=w392, write buffer=w388, error in (no error)=w391) -> (VISA resource name out=w390:refnum<visa-resource-name>, error out=w389:errorcluster)  [unwired: 1 out]
      }
      frame "SMU4" {
        n44 = Delete From Array(array=w411, index=0) -> (deleted portion=w414:string, array with subset deleted=w417:string[])  [unwired: 1 in]
        n45 = Equal?(x=w414, y="ON") -> (x = y?=w412:bool)
        n46 = Delete From Array(array=w417, index=0) -> (deleted portion=w416:string)  [unwired: 1 in, 1 out]
        n47 = Fract/Exp String To Number(string=w416) -> (number=w413:dbl)  [unwired: 3 in, 1 out]
        n48 = Bundle(w412, w413) -> (w410:cluster{bool, dbl})  [unwired: 1 in]
      }
      frame "transfer" {
        # "Is off"
        # "Is on"
        # "Ig off"
        # "Ig on"
        # "Is min"
        # "Is max"
        # "Ig min"
        # "Ig max"
        # "Id min"
        # "Id max"
        # "Id off"
        # "Id on"
        n49 = Delete From Array(array=w551, index=0 ("Index")) -> (deleted portion=w549:string, array with subset deleted=w548:string[])  [unwired: 1 in]
        n50 = Bundle By Name(cluster=w513, "Emergency Stop"=w560) -> (w514:T2)
        n51 = Number To Decimal String(number=w509) -> (decimal integer string=w508:string)  [unwired: 1 in]
        n52 = case shown="\"d\", Default" w549 {
          tunnel: [w645 w646] -> w547
          frame "s" {
            w645 = u16 0 items=["Single", "Double"] ("sweep mode")
          }
          frame "d", Default {
            w646 = u16 1 items=["Single", "Double"] ("sweep mode")
          }
        }
        n53 = Fract/Exp String To Number(string=w548) -> (number=w533:dbl[])  [unwired: 3 in, 1 out]
        n54 = Concatenate Strings(w558, w458, w508, w506, "_T_1_C_L.txt" ("Suffix (transfer)")) -> (w559:string)
        n55 = VISA Write(VISA resource name=w529, write buffer=":PAGE:CHAN:MODE SWE;" ("write buffer (\"\")"), error in (no error)=w528) -> (VISA resource name out=w526:refnum<visa-resource-name>, error out=w527:errorcluster)  [unwired: 1 out]
        n56 = local read "Plot transfer curve extrema vs time"() -> (w456:bool)
        n57 = String To Path(string=w559) -> (path=w557:path)
        n58 = Index Array(array=w533, index #1=0 ("Index")) -> (element #1=w546:dbl, element #2=w545:dbl, element #3=w544:dbl)  [unwired: 2 in]
        n59 = Delete From Array(array=w533, length=3 ("Length"), index=0 ("Index")) -> (array with subset deleted=w531:dbl[])  [unwired: 1 out]
        n60 = case shown="True" w456 {
          tunnel: w505 -> [w562 w565]
          tunnel: w502 -> [_ w564]
          tunnel: [w562 w563] -> w474
          frame False {
          }
          frame True {
            n61 = Build Array (concatenate)(w565, w564) -> (w563:i32[])
          }
        }
        n62 = Bundle By Name(cluster=w538, "Gate Start"=w546, "Gate Stop"=w545, "Gate Step (linear only)"=w544, "Gate Compliance"=w555, "Range mode"=w522, "Range"=w521) -> (w523:T6)
        n63 = Index Array(array=w531, index #1=0 ("Index")) -> (element #1=w541:dbl, element #2=w540:dbl, element #3=w539:dbl)  [unwired: 2 in]
        n64 = call <vilib>:"compatOverwrite.vi"("overwrite (F)"=TRUE) -> ("overwrite?"=w512:T8)
        n65 = Bundle By Name(cluster=w537, "Drain Start"=w541, "Drain Stop"=w540, "Drain Step"=w539, "Drain Compliance"=w556, "Range mode"=w520, "Range"=w519) -> (w524:T7)
        n66 = call "4155C Transfer.vi"("VISA resource name in"=w526, "Gate"=w523, "Drain"=w524, "Timings"=w554, "error in (no error)"=w527, "SMU4"=w455, "sweep mode"=w547, "Panel Controls"=w514) -> ("VG"=w511:dbl[], "Outparams"=w518:T9, "VISA Resource Name out"=w553:refnum<visa-resource-name>, "IS"=w484:dbl[], "ID"=w485:dbl[], "IG"=w483:dbl[], "error out"=w503:errorcluster, "SMU4"=w515:dbl[])  [unwired: 12 in]
        n67 = Unbundle By Name(w518) -> ("V2 Step"=w517:dbl, "V2 Start"=w516:dbl, "Number of points"=w472:i32)
        n68 = call "4155C Split array.vi"("Number of VAR2 steps"=w472, "Y2 data in"=w485, "X data in"=w511, "Y1 data in"=w484, "Y3 data in"=w483, "error in (no error)"=w503) -> ("Array of clusters"=w504:cluster{"Y data in":dbl[], "X data in":dbl[]}[], "error out"=w460:errorcluster)  [unwired: 1 in]
        n69 = case shown="True" "Plot transfer curve extrema vs time" {
          tunnel: w510 -> [w574 w644]
          tunnel: w501 -> [w575 w639]
          tunnel: w487 -> [w568 w635]
          tunnel: w486 -> [w569 w634]
          tunnel: w485 -> [_ w631]
          tunnel: w484 -> [_ w629]
          tunnel: w483 -> [_ w628]
          tunnel: w482 -> [w576 w624]
          tunnel: w481 -> [w577 w623]
          tunnel: w480 -> [w572 w620]
          tunnel: w479 -> [w573 w619]
          tunnel: w478 -> [w567 w616]
          tunnel: w477 -> [w566 w615]
          tunnel: w476 -> [w571 w612]
          tunnel: w475 -> [w570 w611]
          tunnel: w474 -> [_ w604]
          tunnel: [w572 w599] -> w473
          tunnel: w472 -> [_ w598]
          tunnel: [w573 w597] -> w471
          tunnel: [w574 w596] -> w470
          tunnel: [w575 w595] -> w469
          tunnel: [w576 w594] -> w468
          tunnel: [w577 w593] -> w467
          tunnel: [w571 w592] -> w466
          tunnel: [w570 w591] -> w465
          tunnel: [w569 w590] -> w464
          tunnel: [w568 w589] -> w463
          tunnel: [w567 w588] -> w462
          tunnel: [w566 w587] -> w461
          tunnel: w460 -> [w578 w586]
          tunnel: [w578 w582] -> w459
          frame False {
          }
          frame True {
            # "Adjusts graph colors."
            # "Adjusts graph colors."
            # "Ion will be the middle element of the array. The calculation of the index is done only once, since Is, Id, and Ig have the same dimensions."
            # "abs(Ig)"
            # "abs(Is)"
            # "Y1: Is\nY2: Id\nY3: Ig"
            # "abs(Id)"
            # "Adjusts graph colors."
            # "Adjusts graph colors."
            # "Adjusts graph colors."
            n70 = Absolute Value(x=w629) -> (abs(x)=w614:dbl[])
            n71 = Absolute Value(x=w631) -> (abs(x)=w630:dbl[])
            n72 = Absolute Value(x=w628) -> (abs(x)=w617:dbl[])
            n73 = Array Size(array=w630) -> (size(s)=w638:i32)
            n74 = Divide(x=w638, y=2) -> (x/y=w581:dbl)
            n75 = Subtract(x=w581, y=1) -> (x-y=w580:dbl)
            n76 = Array Max & Min(array=w614) -> (max value=w621:dbl, min value=w622:dbl)  [unwired: 2 out]
            n77 = Array Max & Min(array=w630) -> (max value=w643:dbl, min value=w627:dbl)  [unwired: 2 out]
            n78 = Array Max & Min(array=w617) -> (max value=w626:dbl, min value=w625:dbl)  [unwired: 2 out]
            n79 = Index Array(array=w614, index=w580) -> (element=w605:dbl)
            n80 = Index Array(array=w614, index=0) -> (element=w606:dbl)
            n81 = Index Array(array=w630, index=w580) -> (element=w607:dbl)
            n82 = Index Array(array=w630, index=0) -> (element=w608:dbl)
            n83 = Index Array(array=w617, index=w580) -> (element=w610:dbl)
            n84 = Index Array(array=w617, index=0) -> (element=w609:dbl)
            n85 = local write "Ig max"(w626) -> ()
            n86 = local write "Ig min"(w625) -> ()
            n87 = local write "Is max"(w621) -> ()
            n88 = local write "Is min"(w622) -> ()
            n89 = local write "Id max"(w643) -> ()
            n90 = local write "Id min"(w627) -> ()
            n91 = Build Array (concatenate)(w620, w621) -> (w599:dbl[])
            n92 = Build Array (concatenate)(w619, w622) -> (w597:dbl[])
            n93 = local write "Is off"(w606) -> ()
            n94 = local write "Is on"(w605) -> ()
            n95 = Build Array (concatenate)(w644, w643) -> (w596:dbl[])
            n96 = Build Array (concatenate)(w639, w627) -> (w595:dbl[])
            n97 = Build Array (concatenate)(w624, w626) -> (w594:dbl[])
            n98 = Build Array (concatenate)(w623, w625) -> (w593:dbl[])
            n99 = Build Array (concatenate)(w612, w605) -> (w592:dbl[])
            n100 = Build Array (concatenate)(w611, w606) -> (w591:dbl[])
            n101 = Build Array (concatenate)(w634, w607) -> (w590:dbl[])
            n102 = Build Array (concatenate)(w635, w608) -> (w589:dbl[])
            n103 = Build Array (concatenate)(w616, w610) -> (w588:dbl[])
            n104 = Build Array (concatenate)(w615, w609) -> (w587:dbl[])
            n105 = local write "Ig off"(w609) -> ()
            n106 = local write "Ig on"(w610) -> ()
            n107 = local write "Id off"(w608) -> ()
            n108 = local write "Id on"(w607) -> ()
            n109 = control-ref of="Imax vs time"() -> (w633:refnum<vi>)
            n110 = control-ref of="Imin vs time"() -> (w632:refnum<vi>)
            n111 = control-ref of="Ion vs time"() -> (w601:refnum<vi>)
            n112 = control-ref of="Ioff vs time"() -> (w600:refnum<vi>)
            n113 = control-ref of="I vs Vg"() -> (w642:refnum<vi>)
            n114 = call "4155C Split array.vi"("Number of VAR2 steps"=w598, "Y2 data in"=w590, "X data in"=w604, "Y1 data in"=w592, "Y3 data in"=w588, "error in (no error)"=w586) -> ("Array of clusters"=w602:cluster{"Y data in":dbl[], "X data in":dbl[]}[], "error out"=w585:errorcluster)  [unwired: 1 in]
            n115 = call "4155C Split array.vi"("Number of VAR2 steps"=w598, "Y2 data in"=w589, "X data in"=w604, "Y1 data in"=w591, "Y3 data in"=w587, "error in (no error)"=w585) -> ("Array of clusters"=w603:cluster{"Y data in":dbl[], "X data in":dbl[]}[], "error out"=w584:errorcluster)  [unwired: 1 in]
            n116 = call "4155C Split array.vi"("Number of VAR2 steps"=w598, "Y2 data in"=w596, "X data in"=w604, "Y1 data in"=w599, "Y3 data in"=w594, "error in (no error)"=w584) -> ("Array of clusters"=w641:cluster{"Y data in":dbl[], "X data in":dbl[]}[], "error out"=w583:errorcluster)  [unwired: 1 in]
            n117 = call "4155C Split array.vi"("Number of VAR2 steps"=w598, "Y2 data in"=w595, "X data in"=w604, "Y1 data in"=w597, "Y3 data in"=w593, "error in (no error)"=w583) -> ("Array of clusters"=w640:cluster{"Y data in":dbl[], "X data in":dbl[]}[], "error out"=w582:errorcluster)  [unwired: 1 in]
            n118 = call "4155C Config Chart Colours.vi"("Numeric"=w598, "XY Graph 2"=w633) -> ()  [unwired: 6 in]
            n119 = call "4155C Config Chart Colours.vi"("Numeric"=w598, "XY Graph 2"=w632) -> ()  [unwired: 6 in]
            n120 = call "4155C Config Chart Colours.vi"("Numeric"=w598, "XY Graph 2"=w601) -> ()  [unwired: 6 in]
            n121 = call "4155C Config Chart Colours.vi"("Numeric"=w598, "XY Graph 2"=w600) -> ()  [unwired: 6 in]
            n122 = call "4155C Config Chart Colours.vi"("Numeric"=w598, "XY Graph 2"=w642) -> ()  [unwired: 6 in]
            n123 = local write "Imax vs time"(w641) -> ()
            n124 = local write "Imin vs time"(w640) -> ()
            n125 = local write "Ion vs time"(w602) -> ()
            n126 = local write "Ioff vs time"(w603) -> ()
          }
        }
        n127 = local write "I vs Vg"(w504) -> ()
        n128 = Open/Create/Replace File(file path (use dialog)=w557, error in=w459, operation (0:open)=w512) -> (refnum out=w499:refnum<file>, error out=w497:errorcluster)  [unwired: 3 in, 1 out]
        n129 = call "4155C Make Big 2d array.vi"("1D Var1"=w511, "1d IS"=w484, "1d ID"=w485, "1d IG"=w483, "1d SMU4"=w515, "SMU4"=w455, "VAR2 START"=w516, "Number of VAR2 steps"=w472, "VAR2 STEP"=w517, "VAR1 Name"="Vg", "Decimal places in header"=i8 1, "VAR2 Name"="Vd") -> ("Header array"=w500:string[], "Data array"=w498:dbl[][])  [unwired: 14 in]
        n130 = call "4155C Write array to file.vi"("Byte Stream File Refnum"=w499, "Header"=w500, "Data Array"=w498, "error in (no error)"=w497) -> ("dup refnum"=w496:refnum<file>, "error out"=w495:errorcluster)  [unwired: 1 in]
        n131 = Close File(refnum=w496, error in=w495) -> (error out=w552:errorcluster)  [unwired: 1 out]
      }
      frame "pulsedstressV" {
        w682 = 0
        n132 = Number To Decimal String(number=w673) -> (decimal integer string=w728:string)  [unwired: 1 in]
        n133 = Delete From Array(array=w663, index=0 ("Index")) -> (deleted portion=w719:string, array with subset deleted=w718:string[])  [unwired: 1 in]
        n134 = Bundle By Name(cluster=w699, "Emergency Stop"=w731) -> (w700:T2)
        n135 = VISA Write(VISA resource name=w712, write buffer=":PAGE:CHAN:MODE SWE;" ("write buffer (\"\")"), error in (no error)=w711) -> (VISA resource name out=w709:refnum<visa-resource-name>, error out=w710:errorcluster)  [unwired: 1 out]
        n136 = Concatenate Strings(w727, "-pulsedstressV-" ("Substring"), w728, w672, ".txt" ("Substring")) -> (w730:string)
        n137 = case shown="\"d\", Default" w719 {
          tunnel: [w740 w741] -> w717
          frame "s" {
            w740 = u16 0 items=["Single", "Double"] ("sweep mode")
          }
          frame "d", Default {
            w741 = u16 1 items=["Single", "Double"] ("sweep mode")
          }
        }
        n138 = Fract/Exp String To Number(string=w718) -> (number=w713:dbl[])  [unwired: 3 in, 1 out]
        n139 = String To Path(string=w730) -> (path=w726:path)
        n140 = Index Array(array=w713, index #1=0 ("Index")) -> (element #1=w691:dbl, element #2=w690:dbl, element #3=w687:dbl, element #4=w686:dbl, element #5=w685:dbl, element #6=w689:dbl)  [unwired: 5 in]
        n141 = Bundle By Name(cluster=w688, "Pulse period"=w686, "Base voltage"=w687, "Pulse width"=w685) -> (w684:T5)
        n142 = Unbundle By Name(w684) -> ("Pulse period"=w692:dbl)
        n143 = Bundle By Name(cluster=w715, "Gate Start"=w690, "Gate Stop"=w691, "Gate Step (linear only)"=0, "Gate Compliance"=w724, "Range mode"=w705, "Range"=w704) -> (w706:T6)
        n144 = call <vilib>:"compatOverwrite.vi"("overwrite (F)"=TRUE) -> ("overwrite?"=w677:T8)
        n145 = Bundle By Name(cluster=w714, "Drain Start"=w689, "Drain Stop"=w682, "Drain Step"=w682, "Drain Compliance"=w725, "Range mode"=w703, "Range"=w702) -> (w707:T7)
        n146 = call "4155C PulsedStressV.vi"("VISA resource name in"=w709, "sweep mode"=w717, "Panel Controls"=w700, "Gate"=w706, "Drain"=w707, "Timings"=w684, "error in (no error)"=w710, "SMU4"=w651) -> ("VISA Resource Name out"=w722:refnum<visa-resource-name>, "ID"=w680:dbl[], "IG"=w678:dbl[], "Outparams"=w701:T9, "error out"=w723:errorcluster)  [unwired: 3 in]
        n147 = Unbundle By Name(w701) -> ("Number of points"=w679:i32)  [unwired: 2 out]
        n148 = for {
          N: w679 -> [_]
          tunnel: [w737] -> w681 mode=indexing
          tunnel: w692 -> [w739]
          i -> [w738]
          n149 = Multiply(x=w739, y=w738) -> (x*y=w737:dbl)
        }
        n150 = Insert Into Array(array=dbl[][] [] ("Input Array"), new element=w681) -> (w693:dbl[][])  [unwired: 2 in]
        n151 = Insert Into Array(array=w693, new element=w680) -> (w698:dbl[][])  [unwired: 2 in]
        n152 = Insert Into Array(array=w698, new element=w678) -> (w697:dbl[][])  [unwired: 2 in]
        n153 = Transpose 2D Array(2D array=w697) -> (transposed array=w696:dbl[][])
        n154 = Open/Create/Replace File(file path (use dialog)=w726, error in=w723, operation (0:open)=w677) -> (refnum out=w734:refnum<file>, error out=w735:errorcluster)  [unwired: 3 in, 1 out]
        n155 = call "4155C Write array to file.vi"("Byte Stream File Refnum"=w734, "Header"=string[] ["Time /s", "Id /A", "Ig /A"], "Data Array"=w696, "error in (no error)"=w735) -> ("dup refnum"=w732:refnum<file>, "error out"=w733:errorcluster)  [unwired: 1 in]
        n156 = Close File(refnum=w732, error in=w733) -> (error out=w721:errorcluster)  [unwired: 1 out]
      }
      frame "transfer-fpp" {
        n157 = Number To Decimal String(number=w768) -> (decimal integer string=w822:string)  [unwired: 1 in]
        n158 = Bundle By Name(cluster=w798, "Emergency Stop"=w826) -> (w834:T1)
        n159 = Delete From Array(array=w813, index=0 ("Index")) -> (deleted portion=w811:string, array with subset deleted=w810:string[])  [unwired: 1 in]
        n160 = Concatenate Strings(w821, "-transferfpp-" ("Substring"), w822, w766, ".txt" ("Substring")) -> (w824:string)
        n161 = VISA Write(VISA resource name=w790, write buffer=":PAGE:CHAN:MODE SWE;" ("write buffer (\"\")"), error in (no error)=w789) -> (VISA resource name out=w787:refnum<visa-resource-name>, error out=w788:errorcluster)  [unwired: 1 out]
        n162 = case shown="\"d\", Default" w811 {
          tunnel: [w835 w836] -> w809
          frame "s" {
            w835 = u16 0 items=["Single", "Double"] ("sweep mode")
          }
          frame "d", Default {
            w836 = u16 1 items=["Single", "Double"] ("sweep mode")
          }
        }
        n163 = Fract/Exp String To Number(string=w810) -> (number=w794:dbl[])  [unwired: 3 in, 1 out]
        n164 = String To Path(string=w824) -> (path=w820:path)
        n165 = Index Array(array=w794, index #1=0 ("Index")) -> (element #1=w808:dbl, element #2=w807:dbl, element #3=w806:dbl)  [unwired: 2 in]
        n166 = Delete From Array(array=w794, length=3 ("Length"), index=0 ("Index")) -> (array with subset deleted=w792:dbl[])  [unwired: 1 out]
        n167 = Bundle By Name(cluster=w800, "Gate Start"=w808, "Gate Stop"=w807, "Gate Step (linear only)"=w806, "Gate Compliance"=w818, "Range mode"=w783, "Range"=w782) -> (w784:T6)
        n168 = Index Array(array=w792, index #1=0 ("Index")) -> (element #1=w803:dbl, element #2=w802:dbl, element #3=w801:dbl)  [unwired: 2 in]
        n169 = call <vilib>:"compatOverwrite.vi"("overwrite (F)"=TRUE) -> ("overwrite?"=w771:T8)
        n170 = Bundle By Name(cluster=w799, "Drain Start"=w803, "Drain Stop"=w802, "Drain Step"=w801, "Drain Compliance"=w819, "Range mode"=w781, "Range"=w780) -> (w785:T7)
        n171 = call "4155C Transfer-FPP.vi"("VISA resource name in"=w787, "Gate"=w784, "Drain"=w785, "Timings"=w817, "error in (no error)"=w788, "sweep mode"=w809, "Panel Controls"=w834) -> ("VG"=w825:dbl[], "Outparams"=w779:T9, "VISA Resource Name out"=w815:refnum<visa-resource-name>, "Vprobe2"=w775:dbl[], "ID"=w774:dbl[], "IG"=w773:dbl[], "Vprobe1"=w772:dbl[], "error out"=w816:errorcluster)  [unwired: 13 in]
        n172 = Unbundle By Name(w779) -> ("V2 Step"=w778:dbl, "V2 Start"=w777:dbl, "Number of points"=w776:i32)
        n173 = Open/Create/Replace File(file path (use dialog)=w820, error in=w816, operation (0:open)=w771) -> (refnum out=w831:refnum<file>, error out=w832:errorcluster)  [unwired: 3 in, 1 out]
        n174 = call "4155C Make Big 2d array FPP.vi"("1D Var1"=w825, "1d ID"=w774, "1d Vp2"=w775, "1d IG"=w773, "1d Vp1"=w772, "VAR2 START"=w777, "Number of VAR2 steps"=w776, "VAR2 STEP"=w778, "VAR1 Name"="Vg", "Decimal places in header"=i8 1, "VAR2 Name"="Vd") -> ("Header array"=w827:string[], "Data array"=w828:dbl[][])  [unwired: 15 in]
        n175 = call "4155C Write array to file.vi"("Byte Stream File Refnum"=w831, "Header"=w827, "Data Array"=w828, "error in (no error)"=w832) -> ("dup refnum"=w829:refnum<file>, "error out"=w830:errorcluster)  [unwired: 1 in]
        n176 = Close File(refnum=w829, error in=w830) -> (error out=w814:errorcluster)  [unwired: 1 out]
      }
      frame "output" {
        # "Is off"
        # "Is on"
        # "Ig off"
        # "Ig on"
        # "Is min"
        # "Is max"
        # "Ig min"
        # "Ig max"
        # "Id min"
        # "Id max"
        # "Id off"
        # "Id on"
        n177 = Delete From Array(array=w937, index=0 ("Index")) -> (deleted portion=w935:string, array with subset deleted=w934:string[])  [unwired: 1 in]
        n178 = Bundle By Name(cluster=w844, "Emergency Stop"=w946) -> (w900:T1)
        n179 = Number To Decimal String(number=w896) -> (decimal integer string=w895:string)  [unwired: 1 in]
        n180 = case shown="\"d\", Default" w935 {
          tunnel: [w1031 w1032] -> w933
          frame "s" {
            w1031 = u16 0 items=["Single", "Double"] ("sweep mode")
          }
          frame "d", Default {
            w1032 = u16 1 items=["Single", "Double"] ("sweep mode")
          }
        }
        n181 = Fract/Exp String To Number(string=w934) -> (number=w919:dbl[])  [unwired: 3 in, 1 out]
        n182 = Concatenate Strings(w944, w845, w895, w893, "_O_1_C_L.txt" ("Suffix (transfer)")) -> (w945:string)
        n183 = VISA Write(VISA resource name=w915, write buffer=":PAGE:CHAN:MODE SWE;" ("write buffer (\"\")"), error in (no error)=w914) -> (VISA resource name out=w912:refnum<visa-resource-name>, error out=w913:errorcluster)  [unwired: 1 out]
        n184 = String To Path(string=w945) -> (path=w943:path)
        n185 = local read "Plot output curve extrema vs time"() -> (w842:bool)
        n186 = Index Array(array=w919, index #1=0 ("Index")) -> (element #1=w932:dbl, element #2=w931:dbl, element #3=w930:dbl)  [unwired: 2 in]
        n187 = Delete From Array(array=w919, length=3 ("Length"), index=0 ("Index")) -> (array with subset deleted=w917:dbl[])  [unwired: 1 out]
        n188 = case shown="True" w842 {
          tunnel: w892 -> [w948 w951]
          tunnel: w889 -> [_ w950]
          tunnel: [w948 w949] -> w861
          frame False {
          }
          frame True {
            n189 = Build Array (concatenate)(w951, w950) -> (w949:i32[])
          }
        }
        n190 = Bundle By Name(cluster=w924, "Gate Start"=w932, "Gate Stop"=w931, "Gate Step (linear only)"=w930, "Gate Compliance"=w941, "Range mode"=w908, "Range"=w907) -> (w909:T6)
        n191 = Index Array(array=w917, index #1=0 ("Index")) -> (element #1=w927:dbl, element #2=w926:dbl, element #3=w925:dbl)  [unwired: 2 in]
        n192 = call <vilib>:"compatOverwrite.vi"("overwrite (F)"=TRUE) -> ("overwrite?"=w899:T8)
        n193 = Bundle By Name(cluster=w923, "Drain Start"=w927, "Drain Stop"=w926, "Drain Step"=w925, "Drain Compliance"=w942, "Range mode"=w906, "Range"=w905) -> (w910:T7)
        n194 = call "4155C Output.vi"("VISA resource name in"=w912, "Gate"=w909, "Drain"=w910, "Timings"=w940, "error in (no error)"=w913, "SMU4"=w841, "sweep mode"=w933, "Panel controls"=w900) -> ("VD"=w898:dbl[], "Outparams"=w904:T9, "VISA Resource Name out"=w939:refnum<visa-resource-name>, "IS"=w871:dbl[], "ID"=w872:dbl[], "IG"=w870:dbl[], "error out"=w890:errorcluster, "SMU4"=w901:dbl[])  [unwired: 12 in]
        n195 = Unbundle By Name(w904) -> ("V2 Step"=w903:dbl, "V2 Start"=w902:dbl, "Number of points"=w859:i32)
        n196 = call "4155C Split array.vi"("Number of VAR2 steps"=w859, "Y2 data in"=w872, "X data in"=w898, "Y1 data in"=w871, "Y3 data in"=w870, "error in (no error)"=w890) -> ("Array of clusters"=w891:cluster{"Y data in":dbl[], "X data in":dbl[]}[], "error out"=w847:errorcluster)  [unwired: 1 in]
        n197 = case shown="True" "Plot output curve extrema vs time" {
          tunnel: w897 -> [w955 w1030]
          tunnel: w888 -> [w954 w1025]
          tunnel: w874 -> [w960 w1021]
          tunnel: w873 -> [w961 w1020]
          tunnel: w872 -> [_ w1017]
          tunnel: w871 -> [_ w1015]
          tunnel: w870 -> [_ w1014]
          tunnel: w869 -> [w953 w1010]
          tunnel: w868 -> [w952 w1009]
          tunnel: w867 -> [w957 w1006]
          tunnel: w866 -> [w956 w1005]
          tunnel: w865 -> [w959 w1002]
          tunnel: w864 -> [w958 w1001]
          tunnel: w863 -> [w963 w998]
          tunnel: w862 -> [w962 w997]
          tunnel: w861 -> [_ w990]
          tunnel: [w957 w985] -> w860
          tunnel: w859 -> [_ w984]
          tunnel: [w956 w983] -> w858
          tunnel: [w955 w982] -> w857
          tunnel: [w954 w981] -> w856
          tunnel: [w953 w980] -> w855
          tunnel: [w952 w979] -> w854
          tunnel: [w963 w978] -> w853
          tunnel: [w962 w977] -> w852
          tunnel: [w961 w976] -> w851
          tunnel: [w960 w975] -> w850
          tunnel: [w959 w974] -> w849
          tunnel: [w958 w973] -> w848
          tunnel: w847 -> [w964 w972]
          tunnel: [w964 w968] -> w846
          frame False {
          }
          frame True {
            # "Adjusts graph colors."
            # "Adjusts graph colors."
            # "Ion will be the middle element of the array. The calculation of the index is done only once, since Is, Id, and Ig have the same dimensions."
            # "abs(Ig)"
            # "abs(Is)"
            # "Y1: Is\nY2: Id\nY3: Ig"
            # "abs(Id)"
            # "Adjusts graph colors."
            # "Adjusts graph colors."
            # "Adjusts graph colors."
            n198 = Absolute Value(x=w1015) -> (abs(x)=w1000:dbl[])
            n199 = Absolute Value(x=w1017) -> (abs(x)=w1016:dbl[])
            n200 = Absolute Value(x=w1014) -> (abs(x)=w1003:dbl[])
            n201 = Array Size(array=w1016) -> (size(s)=w1024:i32)
            n202 = Divide(x=w1024, y=2) -> (x/y=w967:dbl)
            n203 = Subtract(x=w967, y=1) -> (x-y=w966:dbl)
            n204 = Array Max & Min(array=w1000) -> (max value=w1007:dbl, min value=w1008:dbl)  [unwired: 2 out]
            n205 = Array Max & Min(array=w1016) -> (max value=w1029:dbl, min value=w1013:dbl)  [unwired: 2 out]
            n206 = Array Max & Min(array=w1003) -> (max value=w1012:dbl, min value=w1011:dbl)  [unwired: 2 out]
            n207 = Index Array(array=w1000, index=w966) -> (element=w991:dbl)
            n208 = Index Array(array=w1000, index=0) -> (element=w992:dbl)
            n209 = Index Array(array=w1016, index=w966) -> (element=w993:dbl)
            n210 = Index Array(array=w1016, index=0) -> (element=w994:dbl)
            n211 = Index Array(array=w1003, index=w966) -> (element=w996:dbl)
            n212 = Index Array(array=w1003, index=0) -> (element=w995:dbl)
            n213 = local write "Ig max"(w1012) -> ()
            n214 = local write "Ig min"(w1011) -> ()
            n215 = local write "Is max"(w1007) -> ()
            n216 = local write "Is min"(w1008) -> ()
            n217 = local write "Id max"(w1029) -> ()
            n218 = local write "Id min"(w1013) -> ()
            n219 = Build Array (concatenate)(w1006, w1007) -> (w985:dbl[])
            n220 = Build Array (concatenate)(w1005, w1008) -> (w983:dbl[])
            n221 = local write "Is off"(w992) -> ()
            n222 = local write "Is on"(w991) -> ()
            n223 = Build Array (concatenate)(w1030, w1029) -> (w982:dbl[])
            n224 = Build Array (concatenate)(w1025, w1013) -> (w981:dbl[])
            n225 = Build Array (concatenate)(w1010, w1012) -> (w980:dbl[])
            n226 = Build Array (concatenate)(w1009, w1011) -> (w979:dbl[])
            n227 = Build Array (concatenate)(w998, w991) -> (w978:dbl[])
            n228 = Build Array (concatenate)(w997, w992) -> (w977:dbl[])
            n229 = Build Array (concatenate)(w1020, w993) -> (w976:dbl[])
            n230 = Build Array (concatenate)(w1021, w994) -> (w975:dbl[])
            n231 = Build Array (concatenate)(w1002, w996) -> (w974:dbl[])
            n232 = Build Array (concatenate)(w1001, w995) -> (w973:dbl[])
            n233 = local write "Ig off"(w995) -> ()
            n234 = local write "Ig on"(w996) -> ()
            n235 = local write "Id off"(w994) -> ()
            n236 = local write "Id on"(w993) -> ()
            n237 = control-ref of="Imax vs time"() -> (w1019:refnum<vi>)
            n238 = control-ref of="Imin vs time"() -> (w1018:refnum<vi>)
            n239 = control-ref of="Ion vs time"() -> (w987:refnum<vi>)
            n240 = control-ref of="Ioff vs time"() -> (w986:refnum<vi>)
            n241 = control-ref of="I vs Vg"() -> (w1028:refnum<vi>)
            n242 = call "4155C Split array.vi"("Number of VAR2 steps"=w984, "Y2 data in"=w976, "X data in"=w990, "Y1 data in"=w978, "Y3 data in"=w974, "error in (no error)"=w972) -> ("Array of clusters"=w988:cluster{"Y data in":dbl[], "X data in":dbl[]}[], "error out"=w971:errorcluster)  [unwired: 1 in]
            n243 = call "4155C Split array.vi"("Number of VAR2 steps"=w984, "Y2 data in"=w975, "X data in"=w990, "Y1 data in"=w977, "Y3 data in"=w973, "error in (no error)"=w971) -> ("Array of clusters"=w989:cluster{"Y data in":dbl[], "X data in":dbl[]}[], "error out"=w970:errorcluster)  [unwired: 1 in]
            n244 = call "4155C Split array.vi"("Number of VAR2 steps"=w984, "Y2 data in"=w982, "X data in"=w990, "Y1 data in"=w985, "Y3 data in"=w980, "error in (no error)"=w970) -> ("Array of clusters"=w1027:cluster{"Y data in":dbl[], "X data in":dbl[]}[], "error out"=w969:errorcluster)  [unwired: 1 in]
            n245 = call "4155C Split array.vi"("Number of VAR2 steps"=w984, "Y2 data in"=w981, "X data in"=w990, "Y1 data in"=w983, "Y3 data in"=w979, "error in (no error)"=w969) -> ("Array of clusters"=w1026:cluster{"Y data in":dbl[], "X data in":dbl[]}[], "error out"=w968:errorcluster)  [unwired: 1 in]
            n246 = call "4155C Config Chart Colours.vi"("Numeric"=w984, "XY Graph 2"=w1019) -> ()  [unwired: 6 in]
            n247 = call "4155C Config Chart Colours.vi"("Numeric"=w984, "XY Graph 2"=w1018) -> ()  [unwired: 6 in]
            n248 = call "4155C Config Chart Colours.vi"("Numeric"=w984, "XY Graph 2"=w987) -> ()  [unwired: 6 in]
            n249 = call "4155C Config Chart Colours.vi"("Numeric"=w984, "XY Graph 2"=w986) -> ()  [unwired: 6 in]
            n250 = call "4155C Config Chart Colours.vi"("Numeric"=w984, "XY Graph 2"=w1028) -> ()  [unwired: 6 in]
            n251 = local write "Imax vs time"(w1027) -> ()
            n252 = local write "Imin vs time"(w1026) -> ()
            n253 = local write "Ion vs time"(w988) -> ()
            n254 = local write "Ioff vs time"(w989) -> ()
          }
        }
        n255 = local write "I vs Vd"(w891) -> ()
        n256 = Open/Create/Replace File(file path (use dialog)=w943, error in=w846, operation (0:open)=w899) -> (refnum out=w886:refnum<file>, error out=w884:errorcluster)  [unwired: 3 in, 1 out]
        n257 = call "4155C Make Big 2d array.vi"("1D Var1"=w898, "1d IS"=w871, "1d ID"=w872, "1d IG"=w870, "1d SMU4"=w901, "SMU4"=w841, "VAR2 START"=w902, "Number of VAR2 steps"=w859, "VAR2 STEP"=w903, "VAR1 Name"="Vd", "Decimal places in header"=i8 1, "VAR2 Name"="Vg") -> ("Header array"=w887:string[], "Data array"=w885:dbl[][])  [unwired: 14 in]
        n258 = call "4155C Write array to file.vi"("Byte Stream File Refnum"=w886, "Header"=w887, "Data Array"=w885, "error in (no error)"=w884) -> ("dup refnum"=w883:refnum<file>, "error out"=w882:errorcluster)  [unwired: 1 in]
        n259 = Close File(refnum=w883, error in=w882) -> (error out=w938:errorcluster)  [unwired: 1 out]
      }
      frame "output-fpp" {
        n260 = Number To Decimal String(number=w1058) -> (decimal integer string=w1112:string)  [unwired: 1 in]
        n261 = Bundle By Name(cluster=w1088, "Emergency Stop"=w1115) -> (w1125:T1)
        n262 = Delete From Array(array=w1103, index=0 ("Index")) -> (deleted portion=w1101:string, array with subset deleted=w1100:string[])  [unwired: 1 in]
        n263 = VISA Write(VISA resource name=w1079, write buffer=":PAGE:CHAN:MODE SWE;" ("write buffer (\"\")"), error in (no error)=w1076) -> (VISA resource name out=w1078:refnum<visa-resource-name>, error out=w1077:errorcluster)  [unwired: 1 out]
        n264 = Concatenate Strings(w1111, "-outputfpp-" ("Substring"), w1112, w1057, ".txt" ("Substring")) -> (w1114:string)
        n265 = case shown="\"d\", Default" w1101 {
          tunnel: [w1126 w1127] -> w1099
          frame "s" {
            w1126 = u16 0 items=["Single", "Double"] ("sweep mode")
          }
          frame "d", Default {
            w1127 = u16 1 items=["Single", "Double"] ("sweep mode")
          }
        }
        n266 = Fract/Exp String To Number(string=w1100) -> (number=w1082:dbl[])  [unwired: 3 in, 1 out]
        n267 = String To Path(string=w1114) -> (path=w1110:path)
        n268 = Index Array(array=w1082, index #1=0 ("Index")) -> (element #1=w1098:dbl, element #2=w1097:dbl, element #3=w1096:dbl)  [unwired: 2 in]
        n269 = Delete From Array(array=w1082, length=3 ("Length"), index=0 ("Index")) -> (array with subset deleted=w1081:dbl[])  [unwired: 1 out]
        n270 = Bundle By Name(cluster=w1090, "Gate Start"=w1098, "Gate Stop"=w1097, "Gate Step (linear only)"=w1096, "Gate Compliance"=w1108, "Range mode"=w1074, "Range"=w1073) -> (w1124:T6)
        n271 = Index Array(array=w1081, index #1=0 ("Index")) -> (element #1=w1093:dbl, element #2=w1092:dbl, element #3=w1091:dbl)  [unwired: 2 in]
        n272 = call <vilib>:"compatOverwrite.vi"("overwrite (F)"=TRUE) -> ("overwrite?"=w1062:T8)
        n273 = Bundle By Name(cluster=w1089, "Drain Start"=w1093, "Drain Stop"=w1092, "Drain Step"=w1091, "Drain Compliance"=w1109, "Range mode"=w1072, "Range"=w1075) -> (w1123:T7)
        n274 = call "4155C Output-FPP.vi"("VISA resource name in"=w1078, "Gate"=w1124, "Drain"=w1123, "Timings"=w1107, "error in (no error)"=w1077, "sweep mode"=w1099, "Panel controls"=w1125) -> ("VD"=w1067:dbl[], "Outparams"=w1070:T9, "VISA Resource Name out"=w1105:refnum<visa-resource-name>, "Vprobe2"=w1066:dbl[], "ID"=w1065:dbl[], "IG"=w1064:dbl[], "Vprobe1"=w1063:dbl[], "error out"=w1106:errorcluster)  [unwired: 13 in]
        n275 = Unbundle By Name(w1070) -> ("V2 Step"=w1071:dbl, "V2 Start"=w1069:dbl, "Number of points"=w1068:i32)
        n276 = Open/Create/Replace File(file path (use dialog)=w1110, error in=w1106, operation (0:open)=w1062) -> (refnum out=w1120:refnum<file>, error out=w1121:errorcluster)  [unwired: 3 in, 1 out]
        n277 = call "4155C Make Big 2d array FPP.vi"("1D Var1"=w1067, "1d ID"=w1065, "1d Vp2"=w1066, "1d IG"=w1064, "1d Vp1"=w1063, "VAR2 START"=w1069, "Number of VAR2 steps"=w1068, "VAR2 STEP"=w1071, "VAR1 Name"="Vd", "Decimal places in header"=i8 1, "VAR2 Name"="Vg") -> ("Header array"=w1116:string[], "Data array"=w1117:dbl[][])  [unwired: 15 in]
        n278 = call "4155C Write array to file.vi"("Byte Stream File Refnum"=w1120, "Header"=w1116, "Data Array"=w1117, "error in (no error)"=w1121) -> ("dup refnum"=w1118:refnum<file>, "error out"=w1119:errorcluster)  [unwired: 1 in]
        n279 = Close File(refnum=w1118, error in=w1119) -> (error out=w1104:errorcluster)  [unwired: 1 out]
      }
      frame "itime" {
        n280 = Delete From Array(array=w1135, index=1) -> (deleted portion=w1134:string)  [unwired: 1 in, 1 out]
        n281 = Delete From Array(array=w1135, index=0 ("Index")) -> (deleted portion=w1169:string)  [unwired: 1 in, 1 out]
        n282 = Fract/Exp String To Number(string=w1134) -> (number=w1133:dbl)  [unwired: 3 in, 1 out]
        n283 = case shown="\"l\"" w1169 {
          tunnel: w1168 -> [w1174 w1176 w1180]
          tunnel: [w1173 w1175 w1179] -> w1161
          tunnel: w1133 -> [w1171 _ w1178]
          frame "s" {
            w1172 = u32 0 items=["short  ", "medium  ", "long  "] ("integration time 2")
            n284 = Bundle By Name(cluster=w1174, "integration time"=w1172, "Short/Long integration time"=w1171) -> (w1173:T5)
          }
          frame "m", Default {
            w1177 = u32 1 items=["short  ", "medium  ", "long  "] ("integration time 2")
            n285 = Bundle By Name(cluster=w1176, "integration time"=w1177) -> (w1175:T5)
          }
          frame "l" {
            w1181 = u32 2 items=["short  ", "medium  ", "long  "] ("integration time 2")
            n286 = Bundle By Name(cluster=w1180, "integration time"=w1181, "Short/Long integration time"=w1178) -> (w1179:T5)
          }
        }
      }
      frame "pulsed" {
        n287 = Delete From Array(array=w1220, index=0 ("Index")) -> (deleted portion=w1221:string, array with subset deleted=w1208:string[])  [unwired: 1 in]
        n288 = case shown="\"on\", Default" w1221 {
          tunnel: w1219 -> [w1231 w1234]
          tunnel: [w1230 w1233] -> w1212
          tunnel: w1208 -> [w1228 _]
          frame "on", Default {
            w1229 = u16 1 items=["Continuous", "Pulsed"] ("sweep method")
            n289 = Fract/Exp String To Number(string=w1228) -> (number=w1226:dbl[])  [unwired: 3 in, 1 out]
            n290 = Index Array(array=w1226, index #1=0 ("Index")) -> (element #1=w1225:dbl, element #2=w1224:dbl, element #3=w1223:dbl)  [unwired: 2 in]
            n291 = Bundle By Name(cluster=w1231, "sweep method"=w1229, "Pulse period"=w1225, "Base voltage"=w1224, "Pulse width"=w1223) -> (w1230:T5)
          }
          frame "off" {
            w1232 = u16 0 items=["Continuous", "Pulsed"] ("sweep method")
            n292 = Bundle By Name(cluster=w1234, "sweep method"=w1232) -> (w1233:T5)
          }
        }
      }
      frame "gaterangemode" {
        n293 = Delete From Array(array=w1271, index=0 ("Index")) -> (deleted portion=w1272:string)  [unwired: 1 in, 1 out]
        n294 = case shown="\"f\"" w1272 {
          tunnel: [w1274 w1275 w1276] -> w1261
          frame "a", Default {
            w1274 = u16 0 items=["Auto", "Limited", "Fixed"] ("Gate Range\nmode 2")
          }
          frame "f" {
            w1275 = u16 2 items=["Auto", "Limited", "Fixed"] ("Gate Range\nmode 2")
          }
          frame "l" {
            w1276 = u16 1 items=["Auto", "Limited", "Fixed"] ("Gate Range\nmode 2")
          }
        }
      }
      frame "gaterange" {
        (unwired) u8 11 items=["10fA  ", "100fA  ", "1nA  ", "10nA", "100nA", "1uA", "10uA", "100uA", "1mA", "10mA", "100mA", "1A"] ("Gate Range 2")
        n295 = Delete From Array(array=w1320, index=0 ("Index")) -> (deleted portion=w1310:string)  [unwired: 1 in, 1 out]
        n296 = Scan Value(string=w1310, format string="") -> (value=w1308:dbl)  [unwired: 1 in, 1 out]
        n297 = Logarithm Base 10(1:w1308) -> (0:w1307:dbl)
        n298 = Round To Nearest(number=w1307) -> (nearest integer value=w1306:dbl)
        n299 = Add(x=w1306, y=11.0) -> (x+y=w1304:dbl)
        n300 = To Unsigned Byte Integer(number=w1304) -> (unsigned 8bit integer=w1303:u8)
      }
      frame "drainrange" {
        (unwired) u8 11 items=["10fA  ", "100fA  ", "1nA  ", "10nA", "100nA", "1uA", "10uA", "100uA", "1mA", "10mA", "100mA", "1A"] ("Gate Range 2")
        n301 = Delete From Array(array=w1365, index=0 ("Index")) -> (deleted portion=w1356:string)  [unwired: 1 in, 1 out]
        n302 = Scan Value(string=w1356, format string="") -> (value=w1354:dbl)  [unwired: 1 in, 1 out]
        n303 = Logarithm Base 10(1:w1354) -> (0:w1353:dbl)
        n304 = Round To Nearest(number=w1353) -> (nearest integer value=w1352:dbl)
        n305 = Add(x=w1352, y=11.0) -> (x+y=w1350:dbl)
        n306 = To Unsigned Byte Integer(number=w1350) -> (unsigned 8bit integer=w1349:u8)
      }
      frame "drainrangemode" {
        n307 = Delete From Array(array=w1403, index=0 ("Index")) -> (deleted portion=w1404:string)  [unwired: 1 in, 1 out]
        n308 = case shown="\"f\"" w1404 {
          tunnel: [w1406 w1407 w1408] -> w1393
          frame "a", Default {
            w1406 = u16 0 items=["Auto", "Limited", "Fixed"] ("Gate Range\nmode 2")
          }
          frame "f" {
            w1407 = u16 2 items=["Auto", "Limited", "Fixed"] ("Gate Range\nmode 2")
          }
          frame "l" {
            w1408 = u16 1 items=["Auto", "Limited", "Fixed"] ("Gate Range\nmode 2")
          }
        }
      }
      frame "Error", Default {
      }
      frame "logfile" {
        n309 = Number To Decimal String(number=w1471) -> (decimal integer string=w1506:string)  [unwired: 1 in]
        n310 = Concatenate Strings(w1505, "logfile" ("Substring"), w1506, w1469, ".txt" ("Substring")) -> (w1503:string)
        n311 = String To Path(string=w1503) -> (path=w1476:path)
        n312 = Unbundle(w1502) -> ("integration time"=w1501:u32, "Short/Long integration time"=w1500:dbl, "hold time (sec)"=w1499:dbl, "delay time (sec)"=w1498:dbl, "Step Time (0 disables)"=w1497:dbl, "sweep method"=w1496:u16, "Pulse period"=w1495:dbl, "Base voltage"=w1494:dbl, "Pulse width"=w1493:dbl)
        n313 = Build Array(w1501, w1500, w1499, w1498, w1497, w1496, w1495, w1494, w1493, w1487, w1488, w1489, w1490, w1491, w1492) -> (w1480:dbl[])
        n314 = Insert Into Array(array=dbl[][] [] ("Input Array"), new element=w1480) -> (w1479:dbl[][])  [unwired: 2 in]
        n315 = call <vilib>:"compatOverwrite.vi"("overwrite (F)"=TRUE) -> ("overwrite?"=w1474:T8)
        n316 = Open/Create/Replace File(file path (use dialog)=w1476, error in=w1478, operation (0:open)=w1474) -> (refnum out=w1484:refnum<file>, error out=w1483:errorcluster)  [unwired: 3 in, 1 out]
        n317 = call "4155C Write array to file.vi"("Byte Stream File Refnum"=w1484, "Header"=string[] ["Int Time", "Short/Long Itime", "Hold time", "Delay time", "Step time", "Sweep method", "Pulse period", "Base Voltage", "Pulse width", "Drain compliance", "Gate compliance", "Gate range mode", "Gate range", "S/D range mode", "S/D range"], "Data Array"=w1479, "error in (no error)"=w1483) -> ("dup refnum"=w1486:refnum<file>, "error out"=w1485:errorcluster)  [unwired: 1 in]
        n318 = Close File(refnum=w1486, error in=w1485) -> (error out=w1477:errorcluster)  [unwired: 1 out]
      }
      frame "sample" {
        w1537 = 1
        # "The suffix is Vg_Vd_Time."
        # "Add a time offset (elapsed time) to the time axis."
        # "Adjusts graph colors."
        n319 = Number To Decimal String(number=w1571) -> (decimal integer string=w1609:string)  [unwired: 1 in]
        n320 = Fract/Exp String To Number(string=w1607) -> (number=w1575:dbl[])  [unwired: 3 in, 1 out]
        n321 = Index Array(array=w1575, index=0 ("Index")) -> (element=w1527:dbl)
        n322 = Index Array(array=w1575, index=2 ("Index")) -> (element=w1603:dbl)
        n323 = Index Array(array=w1575, index=3 ("Index")) -> (element=w1524:dbl)
        n324 = Index Array(array=w1575, index=4 ("Index")) -> (element=w1574:dbl)
        n325 = call "4155C Config Sampling Measurements.vi"("Sampling interval"=w1574, "Sample time"=w1524, "Display on/off"=TRUE, "Timings"=w1582, "Num Points"=w1603, "error in (no error)"=w1611, "Drain Compliance"=w1610, "Gate Compliance"=w1590, "VISA session"=w1612) -> ("error out"=w1613:errorcluster, "dup VISA resource name"=w1614:refnum<visa-resource-name>)  [unwired: 1 in]
        n326 = Index Array(array=w1575, index=1 ("Index")) -> (element=w1529:dbl)
        n327 = local read "Plot sample extrema vs time"() -> (w1539:bool)
        n328 = Number To Decimal String(number=w1529) -> (decimal integer string=w1530:string)  [unwired: 1 in]
        n329 = Number To Decimal String(number=w1527) -> (decimal integer string=w1526:string)  [unwired: 1 in]
        n330 = Number To Decimal String(number=w1524) -> (decimal integer string=w1523:string)  [unwired: 1 in]
        n331 = call "4155C Take Sample.vi"("Emergency Stop"=w1587, "error in (no error)"=w1613, "Vd"=w1529, "Vg"=w1527, "VISA resource name in"=w1614) -> ("error out"=w1547:errorcluster, "Id"=w1518:dbl[], "Ig"=w1517:dbl[], "VISA Resource Name out"=w1584:refnum<visa-resource-name>, "Is"=w1519:dbl[], "Time"=w1535:dbl[])  [unwired: 1 in]
        n332 = Insert Into Array(array=w1511, new element=w1518) -> (w1514:dbl[])  [unwired: 1 in]
        n333 = Insert Into Array(array=w1510, new element=w1519) -> (w1516:dbl[])  [unwired: 1 in]
        n334 = Insert Into Array(array=w1512, new element=w1517) -> (w1515:dbl[])  [unwired: 1 in]
        n335 = Add(x=w1535, y=w1531) -> (x+y=w1520:dbl[])
        n336 = Concatenate Strings(w1530, "_" ("Substring"), w1526, "_" ("Substring"), w1523, ".txt" ("Substring")) -> (w1521:string)
        n337 = Concatenate Strings(w1533, w1532, w1609, w1569, "_S_" ("Substring"), w1521) -> (w1608:string)
        n338 = String To Path(string=w1608) -> (path=w1593:path)
        n339 = Insert Into Array(array=w1509, new element=w1520) -> (w1513:dbl[])  [unwired: 1 in]
        n340 = case shown="True" w1539 {
          tunnel: w1520 -> [_ w1617]
          tunnel: [w1615 w1618] -> w1536
          tunnel: w1540 -> [w1615 w1616]
          frame False {
          }
          frame True {
            n341 = Insert Into Array(array=w1616, new element=w1617) -> (w1618:i32[])  [unwired: 1 in]
          }
        }
        n342 = case shown="True" "Plot sample extrema vs time" {
          tunnel: w1519 -> [_ w1647]
          tunnel: w1518 -> [_ w1648]
          tunnel: w1517 -> [_ w1649]
          tunnel: [w1625 w1635] -> w1508
          tunnel: w1547 -> [w1625 w1640]
          tunnel: w1553 -> [w1624 w1652]
          tunnel: w1552 -> [w1623 w1651]
          tunnel: w1551 -> [w1622 w1653]
          tunnel: w1550 -> [w1621 w1650]
          tunnel: w1549 -> [w1620 w1655]
          tunnel: w1548 -> [w1619 w1654]
          tunnel: [w1624 w1639] -> w1546
          tunnel: [w1623 w1633] -> w1545
          tunnel: [w1622 w1637] -> w1544
          tunnel: [w1621 w1632] -> w1543
          tunnel: [w1620 w1638] -> w1542
          tunnel: [w1619 w1631] -> w1541
          tunnel: w1536 -> [_ w1629]
          frame False {
          }
          frame True {
            w1634 = 1
            # "Number of VAR2 steps is 1."
            # "abs(Ig)"
            # "abs(Is)"
            # "abs(Id)"
            # "Adjusts graph colors."
            n343 = Absolute Value(x=w1649) -> (abs(x)=w1626:dbl[])
            n344 = Absolute Value(x=w1648) -> (abs(x)=w1627:dbl[])
            n345 = Absolute Value(x=w1647) -> (abs(x)=w1628:dbl[])
            n346 = Array Max & Min(array=w1628) -> (max value=w1646:dbl, min value=w1643:dbl)  [unwired: 2 out]
            n347 = Array Max & Min(array=w1627) -> (max value=w1645:dbl, min value=w1642:dbl)  [unwired: 2 out]
            n348 = Array Max & Min(array=w1626) -> (max value=w1644:dbl, min value=w1641:dbl)  [unwired: 2 out]
            n349 = local write "Id max"(w1645) -> ()
            n350 = local write "Id min"(w1642) -> ()
            n351 = local write "Ig max"(w1644) -> ()
            n352 = local write "Ig min"(w1641) -> ()
            n353 = Insert Into Array(array=w1655, new element=w1626) -> (w1638:dbl[])  [unwired: 1 in]
            n354 = Insert Into Array(array=w1654, new element=w1626) -> (w1631:dbl[])  [unwired: 1 in]
            n355 = local write "Is max"(w1646) -> ()
            n356 = local write "Is min"(w1643) -> ()
            n357 = Insert Into Array(array=w1653, new element=w1627) -> (w1637:dbl[])  [unwired: 1 in]
            n358 = Insert Into Array(array=w1650, new element=w1627) -> (w1632:dbl[])  [unwired: 1 in]
            n359 = Insert Into Array(array=w1652, new element=w1628) -> (w1639:dbl[])  [unwired: 1 in]
            n360 = Insert Into Array(array=w1651, new element=w1628) -> (w1633:dbl[])  [unwired: 1 in]
            n361 = control-ref of="Imax vs time"() -> (w1656:refnum<vi>)
            n362 = call "4155C Config Chart Colours.vi"("Numeric"=w1634, "XY Graph 2"=w1656) -> ()  [unwired: 6 in]
            n363 = call "4155C Split array.vi"("Number of VAR2 steps"=w1634, "Y2 data in"=w1637, "X data in"=w1629, "Y1 data in"=w1639, "Y3 data in"=w1638, "error in (no error)"=w1640) -> ("Array of clusters"=w1657:cluster{"Y data in":dbl[], "X data in":dbl[]}[], "error out"=w1636:errorcluster)  [unwired: 1 in]
            n364 = call "4155C Split array.vi"("Number of VAR2 steps"=w1634, "Y2 data in"=w1632, "X data in"=w1629, "Y1 data in"=w1633, "Y3 data in"=w1631, "error in (no error)"=w1636) -> ("Array of clusters"=w1630:cluster{"Y data in":dbl[], "X data in":dbl[]}[], "error out"=w1635:errorcluster)  [unwired: 1 in]
            n365 = local write "Imax vs time"(w1657) -> ()
            n366 = local write "Imin vs time"(w1630) -> ()
          }
        }
        n367 = control-ref of="I vs time (Bias Stress)"() -> (w1534:refnum<vi>)
        n368 = call "4155C Split array.vi"("Number of VAR2 steps"=w1537, "Y2 data in"=w1514, "X data in"=w1513, "Y1 data in"=w1516, "Y3 data in"=w1515) -> ("Array of clusters"=w1538:cluster{"Y data in":dbl[], "X data in":dbl[]}[])  [unwired: 2 in, 1 out]
        n369 = local write "I vs time (Bias Stress)"(w1538) -> ()
        n370 = call "4155C Config Chart Colours.vi"("Numeric"=w1537, "XY Graph 2"=w1534) -> ()  [unwired: 6 in]
        n371 = Insert Into Array(array=dbl[][] [] ("Input Array"), new element=w1520) -> (w1597:dbl[][])  [unwired: 2 in]
        n372 = Insert Into Array(array=w1597, new element=w1517) -> (w1596:dbl[][])  [unwired: 2 in]
        n373 = VISA Write(VISA resource name=w1584, write buffer=":DISP ON" ("write buffer (\"\")"), error in (no error)=w1508) -> (VISA resource name out=w1583:refnum<visa-resource-name>, error out=w1585:errorcluster)  [unwired: 1 out]
        n374 = Insert Into Array(array=w1596, new element=w1518) -> (w1595:dbl[][])  [unwired: 2 in]
        n375 = Insert Into Array(array=w1595, new element=w1519) -> (w1589:dbl[][])  [unwired: 2 in]
        n376 = call <vilib>:"compatOverwrite.vi"("overwrite (F)"=TRUE) -> ("overwrite?"=w1572:T8)
        n377 = Open/Create/Replace File(file path (use dialog)=w1593, error in=w1585, operation (0:open)=w1572) -> (refnum out=w1600:refnum<file>, error out=w1599:errorcluster)  [unwired: 3 in, 1 out]
        n378 = Transpose 2D Array(2D array=w1589) -> (transposed array=w1588:dbl[][])
        n379 = call "4155C Write array to file.vi"("Byte Stream File Refnum"=w1600, "Header"=string[] ["Time /s", "Ig /A", "Id /A", "Is /A"], "Data Array"=w1588, "error in (no error)"=w1599) -> ("dup refnum"=w1602:refnum<file>, "error out"=w1601:errorcluster)  [unwired: 1 in]
        n380 = Close File(refnum=w1602, error in=w1601) -> (error out=w1591:errorcluster)  [unwired: 1 out]
      }
      frame "samplei" {
        n381 = Number To Decimal String(number=w1684) -> (decimal integer string=w1735:string)  [unwired: 1 in]
        n382 = Concatenate Strings(w1714, "-samplei-" ("Substring"), w1735, w1683, ".txt" ("Substring")) -> (w1733:string)
        n383 = Fract/Exp String To Number(string=w1732) -> (number=w1699:dbl[])  [unwired: 3 in, 1 out]
        n384 = String To Path(string=w1733) -> (path=w1717:path)
        n385 = Index Array(array=w1699, index=4 ("Index")) -> (element=w1693:dbl)
        n386 = Index Array(array=w1699, index=3 ("Index")) -> (element=w1694:dbl)
        n387 = Index Array(array=w1699, index=1 ("Index")) -> (element=w1696:dbl)
        n388 = Index Array(array=w1699, index=0 ("Index")) -> (element=w1697:dbl)
        n389 = Index Array(array=w1699, index=2 ("Index")) -> (element=w1695:dbl)
        n390 = call "4155C Config SamplingI Measurements.vi"("Sample time"=w1695, "Display on/off"=TRUE, "Timings"=w1706, "Num Points"=w1696, "error in (no error)"=w1737, "Sampling interval"=w1694, "VISA session"=w1738) -> ("error out"=w1739:errorcluster, "dup VISA resource name"=w1740:refnum<visa-resource-name>)  [unwired: 3 in]
        n391 = call "4155C Take SampleI.vi"("Emergency Stop"=w1711, "error in (no error)"=w1739, "Idg 2"=w1697, "Vdg compliance 2"=w1693, "VISA resource name in"=w1740) -> ("error out"=w1709:errorcluster, "Idg"=w1742:dbl[], "Vdg"=w1719:dbl[], "VISA Resource Name out"=w1707:refnum<visa-resource-name>, "Is"=w1741:dbl[], "Time"=w1723:dbl[])  [unwired: 1 in]
        n392 = Insert Into Array(array=dbl[][] [] ("Input Array"), new element=w1723) -> (w1722:dbl[][])  [unwired: 2 in]
        n393 = Insert Into Array(array=w1722, new element=w1719) -> (w1721:dbl[][])  [unwired: 2 in]
        n394 = Insert Into Array(array=w1721, new element=w1742) -> (w1720:dbl[][])  [unwired: 2 in]
        n395 = VISA Write(VISA resource name=w1707, write buffer=":DISP ON" ("write buffer (\"\")"), error in (no error)=w1709) -> (VISA resource name out=w1692:refnum<visa-resource-name>, error out=w1708:errorcluster)  [unwired: 1 out]
        n396 = Insert Into Array(array=w1720, new element=w1741) -> (w1713:dbl[][])  [unwired: 2 in]
        n397 = call <vilib>:"compatOverwrite.vi"("overwrite (F)"=TRUE) -> ("overwrite?"=w1687:T8)
        n398 = Open/Create/Replace File(file path (use dialog)=w1717, error in=w1708, operation (0:open)=w1687) -> (refnum out=w1726:refnum<file>, error out=w1725:errorcluster)  [unwired: 3 in, 1 out]
        n399 = Transpose 2D Array(2D array=w1713) -> (transposed array=w1712:dbl[][])
        n400 = call "4155C Write array to file.vi"("Byte Stream File Refnum"=w1726, "Header"=string[] ["Time /s", "Vdg /V", "Idg /A", "Is /A"], "Data Array"=w1712, "error in (no error)"=w1725) -> ("dup refnum"=w1728:refnum<file>, "error out"=w1727:errorcluster)  [unwired: 1 in]
        n401 = Close File(refnum=w1728, error in=w1727) -> (error out=w1690:errorcluster)  [unwired: 1 out]
        n402 = VISA Write(VISA resource name=w1692, write buffer=";:PAGE:SCON:STAN OFF;:PAGE:CHAN:VSU2:DIS;" ("write buffer (\"\")"), error in (no error)=w1690) -> (VISA resource name out=w1688:refnum<visa-resource-name>, error out=w1689:errorcluster)  [unwired: 1 out]
      }
      frame "#" {
        n403 = VISA Write(VISA resource name=w1773, write buffer=":DISP ON" ("write buffer (\"\")"), error in (no error)=w1772) -> (VISA resource name out=w1771:refnum<visa-resource-name>, error out=w1770:errorcluster)  [unwired: 1 out]
      }
      frame "stressV" {
        n404 = Number To Decimal String(number=w1807) -> (decimal integer string=w1848:string)  [unwired: 1 in]
        n405 = Concatenate Strings(w1832, "-stressV-" ("Substring"), w1848, w1806, ".txt" ("Substring")) -> (w1846:string)
        n406 = Fract/Exp String To Number(string=w1845) -> (number=w1818:dbl[])  [unwired: 3 in, 1 out]
        n407 = String To Path(string=w1846) -> (path=w1836:path)
        n408 = Index Array(array=w1818, index=3 ("Index")) -> (element=w1815:dbl)
        n409 = Index Array(array=w1818, index=1 ("Index")) -> (element=w1813:dbl)
        n410 = Index Array(array=w1818, index=0 ("Index")) -> (element=w1812:dbl)
        n411 = Index Array(array=w1818, index=4 ("Index")) -> (element=w1817:dbl)
        n412 = Index Array(array=w1818, index=2 ("Index")) -> (element=w1814:dbl)
        n413 = call "4155C Config V Stress.vi"("VISA session"=w1851, "ID compliance"=w1815, "VD"=w1813, "VG"=w1812, "IG compliance"=w1814, "error in (no error)"=w1850, "Display on/off"=TRUE) -> ("dup VISA resource name"=w1853:refnum<visa-resource-name>, "error out"=w1852:errorcluster)
        n414 = call "4155C Apply Stress.vi"("error in (no error)"=w1852, "Duration"=w1817, "Emergency Stop"=w1831, "VISA resource name in"=w1853) -> ("error out"=w1829:errorcluster, "VISA Resource Name out"=w1827:refnum<visa-resource-name>)
        n415 = VISA Write(VISA resource name=w1827, write buffer=":DISP ON" ("write buffer (\"\")"), error in (no error)=w1829) -> (VISA resource name out=w1826:refnum<visa-resource-name>, error out=w1828:errorcluster)  [unwired: 1 out]
        n416 = call <vilib>:"compatOverwrite.vi"("overwrite (F)"=TRUE) -> ("overwrite?"=w1811:T8)
        n417 = Open/Create/Replace File(file path (use dialog)=w1836, error in=w1828, operation (0:open)=w1811) -> (refnum out=w1839:refnum<file>, error out=w1838:errorcluster)  [unwired: 3 in, 1 out]
        n418 = call "4155C Write array to file.vi"("Byte Stream File Refnum"=w1839, "Header"=string[] ["V stress completed successfully", ""], "error in (no error)"=w1838) -> ("dup refnum"=w1841:refnum<file>, "error out"=w1840:errorcluster)  [unwired: 2 in]
        n419 = Close File(refnum=w1841, error in=w1840) -> (error out=w1834:errorcluster)  [unwired: 1 out]
      }
      frame "stressI" {
        n420 = Number To Decimal String(number=w1879) -> (decimal integer string=w1916:string)  [unwired: 1 in]
        n421 = Concatenate Strings(w1900, "-stressI-" ("Substring"), w1916, w1878, ".txt" ("Substring")) -> (w1914:string)
        n422 = Fract/Exp String To Number(string=w1913) -> (number=w1888:dbl[])  [unwired: 3 in, 1 out]
        n423 = Index Array(array=w1888, index=1 ("Index")) -> (element=w1884:dbl)
        n424 = Index Array(array=w1888, index=0 ("Index")) -> (element=w1885:dbl)
        n425 = call "4155C Config I Stress.vi"("VISA session"=w1919, "IDG"=w1885, "VDG compliance"=w1884, "error in (no error)"=w1918, "Display on/off"=TRUE) -> ("dup VISA resource name"=w1921:refnum<visa-resource-name>, "error out"=w1920:errorcluster)
        n426 = Index Array(array=w1888, index=2 ("Index")) -> (element=w1886:dbl)
        n427 = String To Path(string=w1914) -> (path=w1904:path)
        n428 = call "4155C Apply Stress.vi"("error in (no error)"=w1920, "Duration"=w1886, "Emergency Stop"=w1899, "VISA resource name in"=w1921) -> ("error out"=w1897:errorcluster, "VISA Resource Name out"=w1895:refnum<visa-resource-name>)
        n429 = VISA Write(VISA resource name=w1895, write buffer=":DISP ON" ("write buffer (\"\")"), error in (no error)=w1897) -> (VISA resource name out=w1894:refnum<visa-resource-name>, error out=w1896:errorcluster)  [unwired: 1 out]
        n430 = call <vilib>:"compatOverwrite.vi"("overwrite (F)"=TRUE) -> ("overwrite?"=w1883:T8)
        n431 = Open/Create/Replace File(file path (use dialog)=w1904, error in=w1896, operation (0:open)=w1883) -> (refnum out=w1907:refnum<file>, error out=w1906:errorcluster)  [unwired: 3 in, 1 out]
        n432 = call "4155C Write array to file.vi"("Byte Stream File Refnum"=w1907, "Header"=string[] ["I stress completed successfully", ""], "error in (no error)"=w1906) -> ("dup refnum"=w1909:refnum<file>, "error out"=w1908:errorcluster)  [unwired: 2 in]
        n433 = Close File(refnum=w1909, error in=w1908) -> (error out=w1902:errorcluster)  [unwired: 1 out]
      }
      frame "vsu2pulse" {
        n434 = Number To Decimal String(number=w1947) -> (decimal integer string=w1982:string)  [unwired: 1 in]
        n435 = Concatenate Strings(w1967, "-vsu2-" ("Substring"), w1982, w1946, ".txt" ("Substring")) -> (w1980:string)
        n436 = Fract/Exp String To Number(string=w1979) -> (number=w1955:dbl[])  [unwired: 3 in, 1 out]
        n437 = String To Path(string=w1980) -> (path=w1971:path)
        n438 = Index Array(array=w1955, index=1 ("Index")) -> (element=w1954:dbl)
        n439 = Index Array(array=w1955, index=0 ("Index")) -> (element=w1952:dbl)
        n440 = call "4155C Config VSU2 Stress.vi"("error in (no error)"=w1984, "VSU2"=w1952, "Display on/off"=TRUE, "VISA session"=w1985) -> ("error out"=w1986:errorcluster, "dup VISA resource name"=w1987:refnum<visa-resource-name>)
        n441 = call "4155C Apply Stress.vi"("error in (no error)"=w1986, "Duration"=w1954, "Emergency Stop"=w1966, "VISA resource name in"=w1987) -> ("error out"=w1964:errorcluster, "VISA Resource Name out"=w1962:refnum<visa-resource-name>)
        n442 = VISA Write(VISA resource name=w1962, write buffer=":DISP ON" ("write buffer (\"\")"), error in (no error)=w1964) -> (VISA resource name out=w1961:refnum<visa-resource-name>, error out=w1963:errorcluster)  [unwired: 1 out]
        n443 = call <vilib>:"compatOverwrite.vi"("overwrite (F)"=TRUE) -> ("overwrite?"=w1951:T8)
        n444 = Open/Create/Replace File(file path (use dialog)=w1971, error in=w1963, operation (0:open)=w1951) -> (refnum out=w1974:refnum<file>, error out=w1973:errorcluster)  [unwired: 3 in, 1 out]
        n445 = call "4155C Write array to file.vi"("Byte Stream File Refnum"=w1974, "Header"=string[] ["VSU2 pulse completed successfully", ""], "error in (no error)"=w1973) -> ("dup refnum"=w1976:refnum<file>, "error out"=w1975:errorcluster)  [unwired: 2 in]
        n446 = Close File(refnum=w1976, error in=w1975) -> (error out=w1969:errorcluster)  [unwired: 1 out]
      }
      frame "sample-fpp" {
        w2024 = string[] ["Time /s", "Id VgVd /A", "Ig VgVd /A", "Vp1 VgVd /V", "Vp2 VgVd /V"] ("Header")
        w2028 = "%d" ("format string")
        n447 = Number To Decimal String(number=w2013) -> (decimal integer string=w2076:string)  [unwired: 1 in]
        n448 = Fract/Exp String To Number(string=w2073) -> (number=w2061:dbl[])  [unwired: 3 in, 1 out]
        n449 = Concatenate Strings(w2067, "-samplefpp-" ("Substring"), w2076, w2012, ".txt" ("Substring")) -> (w2074:string)
        n450 = String To Path(string=w2074) -> (path=w2036:path)
        n451 = Index Array(array=w2061, index=0 ("Index")) -> (element=w2022:dbl)
        n452 = Index Array(array=w2061, index=1 ("Index")) -> (element=w2021:dbl)
        n453 = Index Array(array=w2061, index=2 ("Index")) -> (element=w2069:dbl)
        n454 = Index Array(array=w2061, index=3 ("Index")) -> (element=w2059:dbl)
        n455 = call "4155C Config Sampling Measurements FPP.vi"("VISA session"=w2079, "Num Points"=w2069, "Vg"=w2022, "Display on/off"=TRUE, "Gate Compliance"=w2068, "Drain Compliance"=w2077, "Standby"="Standby", "error in (no error)"=w2078, "Timings"=w2066, "Vd"=w2021, "Sample time"=w2059) -> ("dup VISA resource name"=w2038:refnum<visa-resource-name>, "error out"=w2037:errorcluster)  [unwired: 3 in]
        n456 = Number To Decimal String(number=w2022) -> (decimal integer string=w2048:string)  [unwired: 1 in]
        n457 = call "4155C Take Sample FPP.vi"("VISA resource name in"=w2038, "error in (no error)"=w2037, "Emergency Stop"=w2039) -> ("Time"=w2043:dbl[], "Vp1"=w2053:dbl[], "VISA Resource Name out"=w2019:refnum<visa-resource-name>, "Ig"=w2041:dbl[], "Id"=w2042:dbl[], "Vp2"=w2051:dbl[], "error out"=w2040:errorcluster)  [unwired: 10 in]
        n458 = Insert Into Array(array=dbl[][] [] ("Input Array"), new element=w2043) -> (w2057:dbl[][])  [unwired: 2 in]
        n459 = Number To Decimal String(number=w2021) -> (decimal integer string=w2046:string)  [unwired: 1 in]
        n460 = Insert Into Array(array=w2057, new element=w2042) -> (w2056:dbl[][])  [unwired: 2 in]
        n461 = Concatenate Strings("(Vg = " ("Substring"), w2048, "V, Vd = " ("Substring"), w2046, "V)" ("Substring")) -> (w2044:string)
        n462 = Insert Into Array(array=w2056, new element=w2041) -> (w2055:dbl[][])  [unwired: 2 in]
        n463 = Insert Into Array(array=w2055, new element=w2053) -> (w2052:dbl[][])  [unwired: 2 in]
        n464 = Insert Into Array(array=w2052, new element=w2051) -> (w2020:dbl[][])  [unwired: 2 in]
        n465 = Transpose 2D Array(2D array=w2020) -> (transposed array=w2050:dbl[][])
        n466 = call <vilib>:"compatOverwrite.vi"("overwrite (F)"=TRUE) -> ("overwrite?"=w2017:T8)
        n467 = Open/Create/Replace File(file path (use dialog)=w2036, error in=w2040, operation (0:open)=w2017) -> (refnum out=w2033:refnum<file>, error out=w2034:errorcluster)  [unwired: 3 in, 1 out]
        n468 = Array To Spreadsheet String(array=w2024, 3:w2028) -> (spreadsheet string=w2030:string)  [unwired: 1 in]
        n469 = Search and Replace String(replace all?=TRUE ("replace all? (F)"), input string=w2030, search string="VgVd", replace string=w2044) -> (result string=w2026:string)  [unwired: 4 in, 3 out]
        n470 = Spreadsheet String To Array(format string=w2028, spreadsheet string=w2026, array type (2D Dbl)=w2024) -> (array=w2025:string[])  [unwired: 1 in]
        n471 = call "4155C Write array to file.vi"("Byte Stream File Refnum"=w2033, "Header"=w2025, "Data Array"=w2050, "error in (no error)"=w2034) -> ("dup refnum"=w2031:refnum<file>, "error out"=w2032:errorcluster)  [unwired: 1 in]
        n472 = Close File(refnum=w2031, error in=w2032) -> (error out=w2018:errorcluster)  [unwired: 1 out]
      }
      frame "resample-fpp" {
        w2118 = string[] ["Time /s", "Id VgVd /A", "Ig VgVd /A", "Vp1 VgVd /V", "Vp2 VgVd /V"] ("Header")
        w2122 = "%d" ("format string")
        n473 = Number To Decimal String(number=w2104) -> (decimal integer string=w2162:string)  [unwired: 1 in]
        n474 = Fract/Exp String To Number(string=w2159) -> (number=w2111:dbl[])  [unwired: 3 in, 1 out]
        n475 = Concatenate Strings(w2155, "-resamplefpp-" ("Substring"), w2162, w2105, ".txt" ("Substring")) -> (w2160:string)
        n476 = String To Path(string=w2160) -> (path=w2130:path)
        n477 = Index Array(array=w2111, index=0 ("Index")) -> (element=w2117:dbl)
        n478 = Index Array(array=w2111, index=1 ("Index")) -> (element=w2116:dbl)
        n479 = Number To Decimal String(number=w2117) -> (decimal integer string=w2140:string)  [unwired: 1 in]
        n480 = call "4155C Take Sample FPP.vi"("VISA resource name in"=w2113, "error in (no error)"=w2112, "Emergency Stop"=w2131) -> ("Time"=w2135:dbl[], "Vp1"=w2145:dbl[], "VISA Resource Name out"=w2115:refnum<visa-resource-name>, "Ig"=w2133:dbl[], "Id"=w2134:dbl[], "Vp2"=w2143:dbl[], "error out"=w2132:errorcluster)  [unwired: 10 in]
        n481 = Insert Into Array(array=dbl[][] [] ("Input Array"), new element=w2135) -> (w2149:dbl[][])  [unwired: 2 in]
        n482 = Number To Decimal String(number=w2116) -> (decimal integer string=w2138:string)  [unwired: 1 in]
        n483 = Insert Into Array(array=w2149, new element=w2134) -> (w2148:dbl[][])  [unwired: 2 in]
        n484 = Concatenate Strings("(Vg = " ("Substring"), w2140, "V, Vd = " ("Substring"), w2138, "V)" ("Substring")) -> (w2136:string)
        n485 = Insert Into Array(array=w2148, new element=w2133) -> (w2147:dbl[][])  [unwired: 2 in]
        n486 = Insert Into Array(array=w2147, new element=w2145) -> (w2144:dbl[][])  [unwired: 2 in]
        n487 = Insert Into Array(array=w2144, new element=w2143) -> (w2110:dbl[][])  [unwired: 2 in]
        n488 = call <vilib>:"compatOverwrite.vi"("overwrite (F)"=TRUE) -> ("overwrite?"=w2109:T8)
        n489 = Open/Create/Replace File(file path (use dialog)=w2130, error in=w2132, operation (0:open)=w2109) -> (refnum out=w2127:refnum<file>, error out=w2128:errorcluster)  [unwired: 3 in, 1 out]
        n490 = Array To Spreadsheet String(array=w2118, 3:w2122) -> (spreadsheet string=w2124:string)  [unwired: 1 in]
        n491 = Transpose 2D Array(2D array=w2110) -> (transposed array=w2142:dbl[][])
        n492 = Search and Replace String(replace all?=TRUE ("replace all? (F)"), input string=w2124, search string="VgVd", replace string=w2136) -> (result string=w2120:string)  [unwired: 4 in, 3 out]
        n493 = Spreadsheet String To Array(format string=w2122, spreadsheet string=w2120, array type (2D Dbl)=w2118) -> (array=w2119:string[])  [unwired: 1 in]
        n494 = call "4155C Write array to file.vi"("Byte Stream File Refnum"=w2127, "Header"=w2119, "Data Array"=w2142, "error in (no error)"=w2128) -> ("dup refnum"=w2125:refnum<file>, "error out"=w2126:errorcluster)  [unwired: 1 in]
        n495 = Close File(refnum=w2125, error in=w2126) -> (error out=w2114:errorcluster)  [unwired: 1 out]
      }
      frame "serial" {
        n496 = local read "Termination char\n(0xA = '\\n' = LF)\n(0xD = '\\r' = CR)"() -> (w2195:u8)
        n497 = local read "Enable Termination\nChar (T)"() -> (w2196:bool)
        n498 = Index Array(array=w2203, index=0 ("Index")) -> (element=w2202:string)
        n499 = local read "parity"() -> (w2186:u16)
        n500 = local read "Delay before read (ms)"() -> (w2197:u32)
        n501 = local read "byte count"() -> (w2194:u32)
        n502 = local read "Timeout (ms)"() -> (w2193:u32)
        n503 = local read "VISA resource name"() -> (w2190:refnum<visa-resource-name>)
        n504 = local read "baud rate"() -> (w2189:u32)
        n505 = local read "Serial End Mode for Reads"() -> (w2188:u16)
        n506 = local read "data bits"() -> (w2187:u16)
        n507 = local read "stop bits"() -> (w2192:u16)
        n508 = local read "flow control"() -> (w2191:u16)
        n509 = call "Serial write and read v0.5.vi"("Delay before read (ms)"=w2197, "Termination char\n(0xA = '\\n' = LF)\n(0xD = '\\r' = CR)"=w2195, "Enable Termination\nChar (T)"=w2196, "parity"=w2186, "stop bits"=w2192, "string to write"=w2202, "flow control"=w2191, "byte count"=w2194, "Serial Settings:Serial End Mode for Reads"=w2188, "Timeout (ms)"=w2193, "error in (no error)"=w2208, "VISA resource name"=w2190, "baud rate"=w2189, "data bits"=w2187) -> ("Serial port output"=w2198:string, "error out"=w2207:errorcluster)
        n510 = Build Array (concatenate)(w2198, w2199) -> (w2200:string[])
      }
      frame "pump" {
        # "Time array for valve position"
        # "Time array for absolute plunger position"
        # "Valve position"
        # "Absolute plunger position"
        # "Remove \"_\""
        # "Check if hard stop is pressed."
        # "Check if halt is pressed."
        # "Check if pump is idle. Else halt."
        n511 = Index Array(array=w2278, index=0 ("Index")) -> (element=w2255:string)
        n512 = case shown="\"No error\", Default" w2253 {
          tunnel: w2255 -> [w2314 _ w2316 w2317 w2318 w2319 _ _ w2322 w2323 _]
          tunnel: [w2314 "/1H" w2316 w2317 w2318 w2319 "/1H" "/1H" w2322 w2323 "/1H"] -> w2254
          frame "No error", Default {
          }
          frame "Initialization" {
          }
          frame "Invalid command" {
          }
          frame "Invalid operand" {
          }
          frame "Device not initialized" {
          }
          frame "Internal failure" {
          }
          frame "Plunger overload" {
          }
          frame "Valve overload" {
          }
          frame "Plunger move not allowed" {
          }
          frame "A/D converter failure" {
          }
          frame "Command overflow" {
          }
        }
        n513 = local read "Hard stop pump"() -> (w2257:bool)
        n514 = local read "Halt pump"() -> (w2260:bool)
        n515 = local read "Serial End Mode for Reads"() -> (w2266:u16)
        n516 = local read "flow control"() -> (w2269:u16)
        n517 = local read "stop bits"() -> (w2270:u16)
        n518 = local read "parity"() -> (w2264:u16)
        n519 = local read "Delay before read (ms)"() -> (w2275:u32)
        n520 = local read "byte count"() -> (w2272:u32)
        n521 = local read "Timeout (ms)"() -> (w2271:u32)
        n522 = local read "VISA resource name"() -> (w2268:refnum<visa-resource-name>)
        n523 = local read "baud rate"() -> (w2267:u32)
        n524 = local read "Enable Termination\nChar (T)"() -> (w2274:bool)
        n525 = local read "Termination char\n(0xA = '\\n' = LF)\n(0xD = '\\r' = CR)"() -> (w2273:u8)
        n526 = case shown="True" w2260 {
          tunnel: [w2328 "/1H"] -> w2259
          tunnel: w2254 -> [w2328 _]
          frame False {
          }
          frame True {
            n527 = local write "Halt pump"(FALSE) -> ()
          }
        }
        n528 = case shown="True" w2257 {
          tunnel: [w2325 "/1T"] -> w2258
          tunnel: w2259 -> [w2325 _]
          frame False {
          }
          frame True {
            n529 = local write "Hard stop pump"(FALSE) -> ()
          }
        }
        n530 = local read "data bits"() -> (w2265:u16)
        n531 = String Subset(string=w2249, offset (0)=1) -> (substring=w2247:string)  [unwired: 1 in]
        n532 = call "SPM Pump v0.6.vi"("Termination char\n(0xA = '\\n' = LF)\n(0xD = '\\r' = CR)"=w2273, "Enable Termination\nChar (T)"=w2274, "Timeout (ms)"=w2271, "Serial Settings:Serial End Mode for Reads"=w2266, "byte count"=w2272, "Delay before read (ms)"=w2275, "Time <input>"=w2252, "error in (no error)"=w2283, "Serial port input"=w2258, "VISA resource name"=w2268, "parity"=w2264, "baud rate"=w2267, "stop bits"=w2270, "data bits"=w2265, "flow control"=w2269, "Time units <input>"=w2247) -> ("Input command"=w2246:string, "Serial port data"=w2236:string[], "Pump status"=w2242:string, "Valve position"=w2244:i32, "Absolute plunger position"=w2256:i32, "Serial port"=w2251:string, "error out"=w2282:errorcluster)  [unwired: 1 in, 4 out]
        n533 = case shown="\"?6\"" w2246 {
          tunnel: [w2295 w2303 w2309] -> w2263
          tunnel: w2262 -> [w2295 w2302 w2309]
          tunnel: w2256 -> [_ w2301 _]
          tunnel: w2243 -> [w2294 w2300 w2310]
          tunnel: [w2294 w2300 w2312] -> w2245
          tunnel: w2244 -> [_ _ w2311]
          tunnel: w2241 -> [_ w2299 w2307]
          tunnel: w2240 -> [w2293 w2298 w2308]
          tunnel: [w2293 w2297 w2308] -> w2239
          tunnel: [w2292 w2296 w2306] -> w2238
          tunnel: w2237 -> [w2292 w2296 w2305]
          frame "Q", Default {
          }
          frame "?" {
            n534 = Build Array (concatenate)(w2302, w2301) -> (w2303:i32[])
            n535 = Build Array (concatenate)(w2298, w2299) -> (w2297:i32[])
            n536 = call "4155C Split array.vi"("X data in"=w2297, "Y1 data in"=w2303) -> ("Array of clusters"=w2304:cluster{"Y data in":dbl[], "X data in":dbl[]}[])  [unwired: 5 in, 1 out]
            n537 = local write "Absolute plunger position vs time"(w2304) -> ()
          }
          frame "?6" {
            n538 = Build Array (concatenate)(w2310, w2311) -> (w2312:i32[])
            n539 = Build Array (concatenate)(w2305, w2307) -> (w2306:i32[])
            n540 = call "4155C Split array.vi"("X data in"=w2306, "Y1 data in"=w2312) -> ("Array of clusters"=w2313:cluster{"Y data in":dbl[], "X data in":dbl[]}[])  [unwired: 5 in, 1 out]
            n541 = local write "Valve position vs time"(w2313) -> ()
          }
        }
        n542 = Build Array (concatenate)(w2234, w2236) -> (w2235:string[][])
        n543 = Build Array (concatenate)(w2250, w2251) -> (w2276:string[])
      }
      frame "filename" {
        n544 = Index Array(array=w2337, index=0 ("Index")) -> (element=w2336:string)
      }
    }
    n545 = local read "Time Units"() -> (w103:u16)
    n546 = case shown="0" w103 {
      tunnel: ["Time (Seconds)" ("element") "Time (Minutes)" ("element") "Time (Hours)" ("element")] -> w81
      frame 0 {
      }
      frame 1, Default {
      }
      frame 2 {
      }
    }
    n547 = Build Array(w177, w110, w120, w119, w118, w117, w116, w115, w114, w113, w112, w111, w109) -> (w215:dbl[][])
    n548 = Transpose 2D Array(2D array=w215) -> (transposed array=w214:dbl[][])
    n549 = Concatenate Strings(w74, w73, "Imax_Imin_Ion_Ioff_vs_time.txt" ("Suffix (Imax,Imin,Ion,Ioff)")) -> (w225:string)
    n550 = Build Array(w81, "Is max (A)" ("VAR2 Name"), "Is min (A)" ("VAR2 Name"), "Id max (A)" ("VAR2 Name"), "Id min (A)" ("VAR2 Name"), "Ig max (A)" ("VAR2 Name"), "Ig min (A)" ("VAR2 Name"), "Is on (A)" ("VAR2 Name"), "Is off (A)" ("VAR2 Name"), "Id on (A)" ("VAR2 Name"), "Id off (A)" ("VAR2 Name"), "Ig on (A)" ("VAR2 Name"), "Ig off (A)" ("VAR2 Name")) -> (w220:string[])
    n551 = Array To Spreadsheet String(array=w214, 3:"%e" ("format string")) -> (spreadsheet string=w218:string)  [unwired: 1 in]
    n552 = Array To Spreadsheet String(array=w220, 3:"" ("format string")) -> (spreadsheet string=w219:string)  [unwired: 1 in]
    n553 = String To Path(string=w225) -> (path=w224:path)
    n554 = Build Array(w219, w218) -> (w217:string[])
    n555 = Write to Text File(file (use dialog)=w224, text=w217, error in=w174) -> (refnum out=w226:refnum<file>, error out=w216:errorcluster)  [unwired: 1 in, 1 out]
    n556 = Close File(refnum=w226, error in=w216) -> (error out=w158:errorcluster)  [unwired: 1 out]
    n557 = Build Array(w155, w178) -> (w183:i32[][])
    n558 = Build Array(w81, "Absolute plunger position" ("VAR2 Name")) -> (w186:string[])
    n559 = Transpose 2D Array(2D array=w183) -> (transposed array=w176:i32[][])
    n560 = Array To Spreadsheet String(array=w186, 3:"" ("format string")) -> (spreadsheet string=w185:string)  [unwired: 1 in]
    n561 = Array To Spreadsheet String(array=w176, 3:"%e" ("format string")) -> (spreadsheet string=w182:string)  [unwired: 1 in]
    n562 = Build Array(w185, w182) -> (w188:string[])
    n563 = Concatenate Strings(w74, w73, "plunger_vs_time.txt" ("Suffix (plunger)")) -> (w180:string)
    n564 = String To Path(string=w180) -> (path=w179:path)
    n565 = Write to Text File(file (use dialog)=w179, text=w188, error in=w158) -> (refnum out=w181:refnum<file>, error out=w190:errorcluster)  [unwired: 1 in, 1 out]
    n566 = Close File(refnum=w181, error in=w190) -> (error out=w157:errorcluster)  [unwired: 1 out]
    n567 = Concatenate Strings(w74, w73, "serial_port_output.txt" ("Suffix (serial port log)")) -> (w196:string)
    n568 = String To Path(string=w196) -> (path=w195:path)
    n569 = Build Array(w81, "Serial port input" ("VAR2 Name"), "Pump status" ("VAR2 Name"), "Serial port output: ") -> (w145:string[])
    n570 = Array To Spreadsheet String(array=w151, 3:"" ("format string")) -> (spreadsheet string=w142:string)  [unwired: 1 in]
    n571 = Array To Spreadsheet String(array=w145, 3:"" ("format string")) -> (spreadsheet string=w143:string)  [unwired: 1 in]
    n572 = Array To Spreadsheet String(array=w150, 3:"" ("format string")) -> (spreadsheet string=w201:string)  [unwired: 1 in]
    n573 = Build Array(w143, w142) -> (w144:string[])
    n574 = Write to Text File(file (use dialog)=w195, text=w144, error in=w157) -> (refnum out=w197:refnum<file>, error out=w198:errorcluster)  [unwired: 1 in, 1 out]
    n575 = local write "Serial port data"(w201) -> ()
    n576 = Close File(refnum=w197, error in=w198) -> (error out=w156:errorcluster)  [unwired: 1 out]
    n577 = Build Array(w154, w160) -> (w166:i32[][])
    n578 = Build Array(w81, "Valve port" ("VAR2 Name")) -> (w169:string[])
    n579 = Transpose 2D Array(2D array=w166) -> (transposed array=w161:i32[][])
    n580 = Array To Spreadsheet String(array=w169, 3:"" ("format string")) -> (spreadsheet string=w168:string)  [unwired: 1 in]
    n581 = Array To Spreadsheet String(array=w161, 3:"%e" ("format string")) -> (spreadsheet string=w165:string)  [unwired: 1 in]
    n582 = Build Array(w168, w165) -> (w171:string[])
    n583 = Concatenate Strings(w74, w73, "valve_port_vs_time.txt" ("Suffix (valve)")) -> (w163:string)
    n584 = String To Path(string=w163) -> (path=w162:path)
    n585 = Write to Text File(file (use dialog)=w162, text=w171, error in=w156) -> (refnum out=w164:refnum<file>, error out=w173:errorcluster)  [unwired: 1 in, 1 out]
    n586 = Close File(refnum=w164, error in=w173) -> (error out=w76:errorcluster)  [unwired: 1 out]
    n587 = Build Array(w72, w71, w70, w69) -> (w87:dbl[][])
    n588 = Build Array("Time (Seconds)" ("element"), "Is (A)" ("VAR2 Name"), "Id (A)" ("VAR2 Name"), "Ig (A)" ("VAR2 Name")) -> (w83:string[])
    n589 = Transpose 2D Array(2D array=w87) -> (transposed array=w86:dbl[][])
    n590 = Concatenate Strings(w74, w73, "sample_vs_time.txt" ("Suffix (Imax,Imin,Ion,Ioff)")) -> (w93:string)
    n591 = Array To Spreadsheet String(array=w83, 3:"" ("format string")) -> (spreadsheet string=w82:string)  [unwired: 1 in]
    n592 = Array To Spreadsheet String(array=w86, 3:"%e" ("format string")) -> (spreadsheet string=w90:string)  [unwired: 1 in]
    n593 = String To Path(string=w93) -> (path=w92:path)
    n594 = Build Array(w82, w90) -> (w89:string[])
    n595 = Write to Text File(file (use dialog)=w92, text=w89, error in=w76) -> (refnum out=w94:refnum<file>, error out=w88:errorcluster)  [unwired: 1 in, 1 out]
    n596 = Close File(refnum=w94, error in=w88) -> (error out=w75:errorcluster)  [unwired: 1 out]
  }
  "error out" <- w32
  "Timings Indicator" <- w17
  "SMU4 Indicator" <- w3
  "Is max" <- w15
  "Id max" <- w15
  "Ig max" <- w15
  "Imax vs time" <- w1
  "I vs Vg" <- w1
  "Imin vs time" <- w1
  "I vs Vd" <- w1
  "Serial port data" <- "" ("Serial port data")
  "Valve position vs time" <- cluster{"Y data in":dbl[], "X data in":dbl[]}[] [] ("Valve position vs time")
  "Is min" <- w14
  "Id min" <- w14
  "Ig min" <- w14
  "Ion vs time" <- w1
  "Ioff vs time" <- w1
  "Is on" <- w13
  "Id on" <- w13
  "Ig on" <- w13
  "Is off" <- w12
  "Id off" <- w12
  "Ig off" <- w12
  "I vs time (Bias Stress)" <- w1
